vi "WVDIAL_Main_1.0.vi"() -> ()   [LabVIEW 2012]
uses:
  <vilib>/DAQmx/write.llb/DAQmx Write (Digital 1D Bool NChan 1Samp 1Line).vi
  <vilib>/DAQmx/miscellaneous.llb/DAQmx Fill In Error Info.vi
  under_development/AMCS_Data.vi
  <vilib>/Analysis/baseanly.llb/Mean (DBL).vi
  H2O_DIAL/LabVIEW-2012/Scalar_Data.vi
  H2O_DIAL/LabVIEW-2012/Bristol WM V2_31b/CLDevIFace.dll
  <vilib>/Analysis/NI_AALBase.lvlib
panel:
  out "AMCS_Profile":i32
  out "FileHour":i32=18
  out "L_Count":i32=12
  out "sigma_off_total":dbl[](array[numeric])=[4.888035870829203e-25, 4.854608115475229e-25, 4.821315130033936e-25, 4.788157195692115e-25, 4.755134589463832e-25, 4.722247583943701e-25, 4.689496446877888e-25, 4.656881440910823e-25, 4.6244028232034e-25, 4.592060845167014e-25, 4.55985575212019e-25, 4.527787783052784e-25, 4.495857170275024e-25, 4.4640641392417e-25, 4.432408908236268e-25, 4.400891688098754e-25, 4.369512682080274e-25, 4.338272085590705e-25, 4.307170085904759e-25, 4.276206862115827e-25, 4.245382584820222e-25, 4.214697415991576e-25, 4.184151508878279e-25, 4.153745007733512e-25, 4.123478047759034e-25, 4.093350754997215e-25, 4.0633632461153848e-25, 4.0335156284150834e-25, 4.0038079996697135e-25, 3.9742404480868766e-25, 3.9448130521677145e-25, 3.915525880745368e-25, 3.886378992858531e-25, 3.8573724377461643e-25, 3.8285062548278185e-25, 3.7997804736545024e-25, 3.7711951139370566e-25, 3.7427501855176308e-25, 3.7144456884042655e-25, 3.686281612771603e-25, 3.658257939015542e-25, 3.6303746377467797e-25, 3.602631669916555e-25, 3.5750289867515567e-25, 3.5475665299476097e-25, 3.5202442316525487e-25, 3.4930620145687864e-25, 3.466019792025494e-25, 3.4391174681118262e-25, 3.412354937708723e-25, 3.385732086655022e-25, 3.3592487917865697e-25, 3.3329049211414267e-25, 3.306700333974482e-25, 3.280634880983416e-25, 3.2547084043508965e-25, 3.228920737922699e-25, 3.203271707354926e-25, 3.1777611302055785e-25, 3.1523888161216317e-25, 3.127154566968838e-25, 3.102058176967416e-25, 3.0770994328759967e-25, 3.0522781141008815e-25, 3.0275939928903318e-25, 3.0030468344607627e-25, 2.9786363971981933e-25, 2.9543624327416916e-25, 2.930224686195949e-25, 2.906222896311306e-25, 2.882356795584999e-25, 2.8586261104367467e-25, 2.835030561394528e-25, 2.811569863239953e-25, 2.788243725123392e-25, 2.7650518508047145e-25, 2.741993938722939e-25, 2.719069682202312e-25, 2.696278769575161e-25, 2.673620884356008e-25, 2.651095705348542e-25, 2.628702906852776e-25, 2.6064421587391947e-25, 2.584313126623251e-25, 2.562315472013588e-25, 2.540448852422533e-25, 2.518712921495533e-25, 2.4971073291533783e-25, 2.475631721705256e-25, 2.454285741983474e-25, 2.433069029434547e-25, 2.411981220251513e-25, 2.3910219474927565e-25, 2.370190841148622e-25, 2.3494875282985535e-25, 2.3289116331441013e-25, 2.3084627771705737e-25, 2.2881405791714577e-25, 2.2679446553956784e-25, 2.2478746195897673e-25, 2.22793008307951e-25, 2.208110654850464e-25, 2.188415941625169e-25, 2.168845547931586e-25, 2.149399076143407e-25, 2.1300761265550973e-25, 2.110876297449633e-25, 2.0917991851171733e-25, 2.072844383934657e-25, 2.054011486389122e-25, 2.0353000831508104e-25, 2.016709763077787e-25, 1.998240113264655e-25, 1.979890719093385e-25, 1.9616611642341368e-25, 1.943551030698017e-25, 1.925559898865328e-25, 1.9076873474916518e-25, 1.8899329537437417e-25, 1.8722962932379024e-25, 1.8547769400210756e-25, 1.8373744666260693e-25, 1.8200884440825555e-25, 1.8029184419330962e-25, 1.785864028250439e-25, 1.768924769659363e-25, 1.7521002313557632e-25, 1.735389977127581e-25, 1.7187935693766226e-25, 1.702310569139568e-25, 1.6859405361114919e-25, 1.6696830286658545e-25, 1.6535376038945889e-25, 1.6375038176257498e-25, 1.621581224454772e-25, 1.6057693777875647e-25, 1.5900678298637916e-25, 1.5744761318177563e-25, 1.558993833699771e-25, 1.543620484527584e-25, 1.5283556323523553e-25, 1.513198824282104e-25, 1.498149606572178e-25, 1.4832075246641388e-25, 1.4683721232497087e-25, 1.4536429463567547e-25, 1.4390195374017408e-25, 1.424501439277071e-25, 1.4100881944445769e-25, 1.3957793449837002e-25, 1.381574432716146e-25, 1.3674729992776922e-25, 1.353474586215468e-25, 1.3395787350844606e-25, 1.325784987569173e-25, 1.3120928855546477e-25, 1.2985019712580151e-25, 1.2850117873277534e-25, 1.2716218769548856e-25, 1.2583317839794236e-25, 1.2451410530256942e-25, 1.2320492295860694e-25, 1.2190558601549445e-25, 1.2061604923388985e-25, 1.1933626749670006e-25, 1.1806619582041493e-25, 1.1680578936635882e-25, 1.1555500345124245e-25, 1.1431379355845816e-25, 1.130821153462839e-25, 1.11859924660529e-25, 1.106471775420178e-25, 1.094438302366916e-25, 1.0824983920307019e-25, 1.0706516112017506e-25, 1.0588975289648329e-25, 1.0472357167332237e-25, 1.0356657483440625e-25, 1.024187200079566e-25, 1.0127996507244631e-25, 1.0015026816012569e-25, 9.902958765939357e-26, 9.791788221702149e-26, 9.68151107381336e-26, 9.572123238770103e-26, 9.463620658860708e-26, 9.355999302019208e-26, 9.249255161638679e-26, 9.143384256042965e-26, 9.038382628274446e-26, 8.934246345371541e-26, 8.830971497843464e-26, 8.728554198992872e-26, 8.62699058411531e-26, 8.526276809671997e-26, 8.426409052334914e-26, 8.327383508075767e-26, 8.229196391044237e-26, 8.131843932536565e-26, 8.035322379788044e-26, 7.939627994867628e-26, 7.844757053335767e-26, 7.750705843063878e-26, 7.65747066289159e-26, 7.565047821351042e-26, 7.47343363532067e-26, 7.382624428699225e-26, 7.292616531039518e-26, 7.203406276287137e-26, 7.114990001406464e-26, 7.027364045059868e-26, 6.940524746389362e-26, 6.85446844368123e-26, 6.769191473247965e-26, 6.684690168165317e-26, 6.600960857107768e-26, 6.517999863394936e-26, 6.435803503717334e-26, 6.354368087372936e-26, 6.273689915185572e-26, 6.193765278681275e-26, 6.114590459282069e-26, 6.036161727495792e-26, 5.958475342308923e-26, 5.881527550516134e-26, 5.805314586163766e-26, 5.729832670099857e-26, 5.655078009533302e-26, 5.581046797662917e-26, 5.507735213469193e-26, 5.435139421405333e-26, 5.36325557132649e-26, 5.292079798345033e-26, 5.221608222852683e-26, 5.1518369505608076e-26, 5.0827620725253844e-26, 5.014379665432141e-26, 4.9466857916821155e-26, 4.879676499724133e-26, 4.8133478243835596e-26, 4.7476957871630115e-26, 4.6827163967351294e-26, 4.618405649298157e-26, 4.554759529166947e-26, 4.491774009265494e-26, 4.4294450516974745e-26, 4.3677686083139524e-26, 4.306740621440293e-26, 4.2463570244387956e-26, 4.1866137424661286e-26, 4.127506693180156e-26, 4.069031787434629e-26, 4.011184930095246e-26, 3.953962020783545e-26, 3.8973589546741365e-26, 3.84137162332915e-26, 3.785995915494e-26, 3.7312277179583384e-26, 3.677062916385059e-26, 3.623497396187796e-26, 3.5705270434125054e-26, 3.518147745597146e-26, 3.4663553926918453e-26, 3.4151458779350305e-26, 3.3645150987763337e-26, 3.3144589578214325e-26, 3.264973363720337e-26, 3.216054232151887e-26, 3.1676974867802074e-26, 3.119899060201809e-26, 3.072654894964087e-26, 3.025960944534977e-26, 2.979813174386497e-26, 2.9342075629720175e-26, 2.889140102874887e-26, 2.8446068018571114e-26, 2.800603684031854e-26]
  out "sigma_on_total":dbl[](array[numeric])=[3.490042879585289e-23, 3.4896341790922685e-23, 3.4889762071158304e-23, 3.488068250151699e-23, 3.486909676211499e-23, 3.48549993542674e-23, 3.4838385609191393e-23, 3.4819251695340833e-23, 3.479759462007997e-23, 3.477341223906918e-23, 3.4746703260906816e-23, 3.47174672467967e-23, 3.4685704618961385e-23, 3.465141665984221e-23, 3.461460551401806e-23, 3.457527419211947e-23, 3.453342656969817e-23, 3.448906738624602e-23, 3.4442202246214284e-23, 3.4392837616682326e-23, 3.434098082430858e-23, 3.428664005432775e-23, 3.422982434615018e-23, 3.417054358917814e-23, 3.4108808516072814e-23, 3.4044630702817483e-23, 3.397802255409811e-23, 3.390899730392353e-23, 3.383756900435442e-23, 3.376375251923111e-23, 3.368756351057052e-23, 3.360901843775463e-23, 3.3528134537865166e-23, 3.344492982272624e-23, 3.335942306183597e-23, 3.3271633776370865e-23, 3.318158221993735e-23, 3.3089289371486604e-23, 3.299477691788866e-23, 3.2898067243876535e-23, 3.279918341157314e-23, 3.269814915144566e-23, 3.259498884386024e-23, 3.24897275031573e-23, 3.238239076130052e-23, 3.227300485415394e-23, 3.21615965972714e-23, 3.204819337748524e-23, 3.193282312695606e-23, 3.181551430802064e-23, 3.169629589879774e-23, 3.157519736729644e-23, 3.1452248655446696e-23, 3.132748016189897e-23, 3.120092272051889e-23, 3.107260757867697e-23, 3.094256638256482e-23, 3.081083115312845e-23, 3.0677434265982754e-23, 3.054240843226174e-23, 3.0405786681460624e-23, 3.0267602333919474e-23, 3.012788898770482e-23, 2.99866804931177e-23, 2.984401093546342e-23, 2.9699914613734513e-23, 2.955442601832349e-23, 2.940757981602586e-23, 2.925941082278427e-23, 2.9109953991996763e-23, 2.895924438752617e-23, 2.8807317167162414e-23, 2.865420756317372e-23, 2.849995086407571e-23, 2.834458239150023e-23, 2.818813748548795e-23, 2.803065148592016e-23, 2.787215971116496e-23, 2.771269744109115e-23, 2.755229990137636e-23, 2.739100224507032e-23, 2.7228839532475316e-23, 2.706584671843548e-23, 2.690205863490408e-23, 2.673750997388079e-23, 2.657223527172833e-23, 2.6406268893866064e-23, 2.6239645021831286e-23, 2.607239763477325e-23, 2.5904560500280996e-23, 2.5736167156696623e-23, 2.5567250898853516e-23, 2.539784477107411e-23, 2.5227981549794207e-23, 2.5057693731555458e-23, 2.4887013522394087e-23, 2.471597282956038e-23, 2.454460324501361e-23, 2.437293603900355e-23, 2.4201002150211167e-23, 2.402883217538624e-23, 2.385645635851179e-23, 2.3683904585127427e-23, 2.351120637608329e-23, 2.3338390871505237e-23, 2.3165486834754068e-23, 2.2992522636352133e-23, 2.2819526251359127e-23, 2.2646525256153023e-23, 2.2473546815634482e-23, 2.230061768719921e-23, 2.2127764207900367e-23, 2.195501229556526e-23, 2.1782387440441194e-23, 2.160991470701159e-23, 2.143761872556912e-23, 2.1265523693862868e-23, 2.109365337122134e-23, 2.0922031077433445e-23, 2.0750679694496088e-23, 2.0579621658458087e-23, 2.0408878965264313e-23, 2.0238473165015015e-23, 2.0068425366661072e-23, 1.9898756232137357e-23, 1.9729485980000502e-23, 1.9560634386795936e-23, 1.9392220786262192e-23, 1.9224264070473828e-23, 1.9056782690457042e-23, 1.8889794661029254e-23, 1.8723317558719184e-23, 1.855736852629747e-23, 1.8391964275893473e-23, 1.8227121088478705e-23, 1.806285481900235e-23, 1.7899180898616018e-23, 1.773611433861678e-23, 1.7573669732317703e-23, 1.741186125936493e-23, 1.7250702690911692e-23, 1.7090207391268152e-23, 1.6930388321237217e-23, 1.6771258046596068e-23, 1.661282873734126e-23, 1.6455112174985683e-23, 1.6298119756367283e-23, 1.614186249828583e-23, 1.598635104155938e-23, 1.5831595657904855e-23, 1.567760625211793e-23, 1.552439236910916e-23, 1.5371963196965152e-23, 1.522032757473284e-23, 1.5069493995606855e-23, 1.4919470612189036e-23, 1.477026524242552e-23, 1.4621885376172283e-23, 1.4474338176755096e-23, 1.4327630490148282e-23, 1.4181768849089416e-23, 1.403675947667607e-23, 1.3892608295456937e-23, 1.3749320929216795e-23, 1.3606902710831856e-23, 1.3465358687081003e-23, 1.332469362175979e-23, 1.3184912006315121e-23, 1.304601805945408e-23, 1.2908015735995458e-23, 1.2770908731077424e-23, 1.2634700487137352e-23, 1.2499394195353328e-23, 1.2364992805313888e-23, 1.2231499026968916e-23, 1.2098915337982155e-23, 1.1967243987797148e-23, 1.1836487002238083e-23, 1.1706646189619215e-23, 1.1577723145735427e-23, 1.1449719257807597e-23, 1.1322635710406168e-23, 1.1196473489796478e-23, 1.1071233389221606e-23, 1.0946916011717084e-23, 1.0823521778637897e-23, 1.0701050929498414e-23, 1.0579503530345327e-23, 1.0458879477268549e-23, 1.0339178499011404e-23, 1.0220400163641383e-23, 1.0102543881484885e-23, 9.985608910260597e-24, 9.869594358367067e-24, 9.754499189862458e-24, 9.640322227217557e-24, 9.527062156995094e-24, 9.414717532061861e-24, 9.303286777093004e-24, 9.192768189885375e-24, 9.083159948714375e-24, 8.974460112323461e-24, 8.866666625126608e-24, 8.759777321083854e-24, 8.653789926727215e-24, 8.548702063774183e-24, 8.444511253202335e-24, 8.341214918838909e-24, 8.238810389419842e-24, 8.137294903148705e-24, 8.036665608577946e-24, 7.936919569739024e-24, 7.838053767973498e-24, 7.740065104792213e-24, 7.642950405338446e-24, 7.546706420091712e-24, 7.451329828211826e-24, 7.356817239808839e-24, 7.263165198494959e-24, 7.170370184815645e-24, 7.078428616460998e-24, 6.987336853161977e-24, 6.897091197425113e-24, 6.8076878974105e-24, 6.719123148241058e-24, 6.631393095931324e-24, 6.54449383712704e-24, 6.4584214234832185e-24, 6.3731718616386814e-24, 6.288741117137584e-24, 6.205125113814784e-24, 6.1223197384036285e-24, 6.040320840135283e-24, 5.959124233842455e-24, 5.878725700858363e-24, 5.79912099094532e-24, 5.720305824157253e-24, 5.64227589189973e-24, 5.565026858473326e-24, 5.4885543637702884e-24, 5.412854022527149e-24, 5.3379214276707424e-24, 5.263752150713538e-24, 5.190341743319676e-24, 5.1176857383675426e-24, 5.045779651873086e-24, 4.974618983303745e-24, 4.9041992172131e-24, 4.8345158245928204e-24, 4.765564263342602e-24, 4.697339979783611e-24, 4.629838410103098e-24, 4.563054980342238e-24, 4.496985108006421e-24, 4.431624203399418e-24, 4.36696766956464e-24, 4.3030109039670755e-24, 4.2397492991573704e-24, 4.177178243062485e-24, 4.115293120908651e-24, 4.054089314905932e-24, 3.993562205740054e-24, 3.933707172949696e-24, 3.8745195958165464e-24, 3.815994853553171e-24, 3.7581283271459395e-24, 3.700915398498208e-24, 3.644351452219004e-24, 3.5884318755724674e-24, 3.533152059539341e-24, 3.4785073989091114e-24, 3.4244932929904e-24, 3.371105146433994e-24, 3.3183383692901385e-24, 3.2661883776563498e-24, 3.2146505942936803e-24, 3.1637204489385725e-24]
  out "background start":u32=269
  in  "Tab Control 2":enum32{"WV ND far", "WV ND near"}(tab)
  out "Water Vapor Number Density":dbl[][](graph)=[[0.5267745722096372, 1.0816655502265025, 0.7857849169072013, 0.7477019555239035, 1.1563560837736724, 1.3171998032055208, 1.3231734283890237, 1.0229480459758586, 0.8099310805147446, 1.0288102942698314, 1.0490255634819494, 0.8954092055648583, 0.9324215101778409, 0.8762260068675822, 0.7790591099414911, 0.8327406457641141, 0.7704082202159364, 0.5844811914297862, 0.6547568349937917, 0.8309364506920026, 0.8146764873524291, 0.7795089686669525, 0.7138471934895959, 0.6391289574628901, 0.6939700094906176, 0.7387482811512458, 0.5462573277969212, 0.33740432735257525, 0.524099558332941, 0.5415332827292677, 0.25587531060911606, 0.32034867927546745, 0.3575458365147231, 0.19987909534956147, -0.04398480306339893, -0.3018841632955589, -0.08562036624041874, 0.3956793663354093, 0.316745841175725, -0.17952793102078793, 0.10063267322036752, 0.11266719606812724, 0.029212134890287074, -0.005416362214295599, -0.001903108817248135, 0.024827606151215636, 0.09438149063711843, 0.13636686041364063, 0.09853184491889724, 0.02006830264986938, -0.1100190870486176, -0.011423208972600938, 0.22560075143987507, 0.23855203986244836, 0.18772422030911864, 0.1248592220030643, -0.1159789262566526, -0.09672114603628404, -0.002076973429409002, 0.07764150511111109, 0.08671851842324418, 0.010370500718089025, -0.04877001832258952, -0.09879008518513611, 0.196069456255276, 0.16890990444127219, 0.2027158700169282, 0.47342868266577487, 0.2732503005639838, -0.21673756779330117, -0.009709955271929215, 0.1780787605318169, -0.18035544514716292, -0.09516280572167025, -0.210624930189063, 0.15126704138773134, 0.37711181552750694, -0.2407750842687604, -0.06818293330208619, 0.4479847852605204, 0.15992717017361327, -0.026875771508593577, 0.33346537041116026, 0.6057422007030442, 0.2837007114383953, -0.387948288010905, -0.430868484135778, 0.1171368056605578, 0.2825750335377916, 0.25290766375296486, 0.3235685707096946, 0.294635786603805, 0.15630875076023204, -0.17215583026651332, 0.07190604755466319, 0.5111632653992029, 0.4545339946147383, 0.1397417212111138, -0.379868786050122, -0.8200386753384453, 0.9689769619728654, 1.2154721509976958, 0.027706077248837634, -0.451600315057674, -0.18393792610598184, 0.26802923421484454, 0.06982906738396868, 0.008175721206703183, 0.34464584312575747, 0.775324515204279, -0.9206634231342339, -1.054693026338104, 0.05417378371590325, 0.3787930859671527, 0.1528806900268664, -0.17890474033164738, -0.03290798453116943, 0.17150327086091385, 0.10226783329265791, 0.026323152799793855, 0.14546580088898983, 0.15324308143002588, 0.1999669318893245, -0.3505358779777044, -0.6040003896777243, -0.19197175189892304, 0.41483200698530504, 0.25996478520600325, 0.1901900371465814, -0.7004410472584591, 0.03417523868208899, 0.9773516762567699, 0.9501600424919857, 3.8179055985644914, -0.7387811622909695, -1.292310093419745, -3.4707865579805204, -4.806919839772366, -3.2236942041133716, -0.2798646999882494, -0.5041588894213339, 0.15387554509916093, -2.286184189921483, -6.1689901157875, 0.4414912597114918, -1.0941982539352222, 4.107096638589786, 7.0494086102953135, 5.093420412613982, -1.186817248260524, -2.4693646495361077, 17.233690686949487, 0.16757072698059172, 0.7104219413732543, 11.659803406100098, 0.9497546635922111, -4.150373043253479, -4.099503865718477, -20.766083051079526, -9.002561009044582, 8.821221493764776, -17.7174813523336, -1.1751756583085076, -6.409331662715958, -12.307070884759122, 3.2739376460348315, -0.16355277685023256, -1.7278023908845879, 20.244230401911185, 8.261047619107535, -11.304691487958216, -8.357847181177188, -0.683969220017551, 25.576749641541674, 0.03888795481451756, -3.5614818406988205, 7.989633180877991, 10.328796990583767, -2.196067163503004, -3.4876165534276327, -5.383896494369181, -15.158339724766968, -9.002865651652682, -16.098176364767838, 7.287929865782665, 1.9677812793929124, 5.186685665765197, -0.8233271906171977, 1.5188061622709401, 9.881681545336587, 13.354340316245327, 17.543981154187094, 2.971290702331586, -13.18169395475072, -15.400954328693494, -13.957629394095024, -31.075136408591785, -26.935662472931995, -8.138951564843802, -7.326056577513869, -3.502353752083309, 3.911699212234371, -4.294086845093831, 23.18118721705451, 14.987899790461576, 6.437164591458738, -2.523411218458799, 6.497127824545888, -1.9683154922323156, 0.7529285854770654, -25.600648943018182, -10.52685287943841, 20.134382483909995, -6.0244636268000615, 21.12692930038622, 2.144915244484192, 47.75224805371796, 3.818730797626004, -6.536865277783475, 13.099227893812442, 48.22712037716169, 45.290460164779205, 3.60781654357059, 15.912476957433306, -33.947777326737814, 21.4727068022259, -34.11700126806532, 5.3665409079956214, 33.86809985241948, -37.57424460030235, -85.7767439605924, -52.75415349112659, -34.88803865506797, -22.239237234636768, 19.69441058235572, -105.06374008086121, -8.755512075683884, -6.4485892955900175, -1.0583048975403269, 23.788435843550058, 62.07659802333474, 22.437904657032785, 7.423763482952456, -1.4124692383830593, -51.624147123828145, 45.16870976535536, 28.56129984362196, -2.639584028437023, -24.22307764432475, 7.240569189963771, -7.739305471169459, -37.35816143994053, 1.0244452934635038, -10.305504179883442, 16.74709280360141, 1.888878380765623, -16.968743658232242, 13.056677566409775, 17.44799599784629, -7.35298759849147, -0.1908743950074914, -11.436677267617473, 4.855902298247621, -10.394570497652436, 14.487727137462723, 26.002729568728288, -31.076998008605173, -112.89098296015568, -50.76728953266004, -8.064309931248644, -18.781235808776238, 16.929688279117574, -17.58011679033343, -5.052252895180237, -20.3864023129576, -12.830066550660884, 0.0, 0.0, 0.0, 0.0]]
  out "Water Vapor Number Density 2":dbl[][](graph)=[[1.1482348388286592, 2.017982964091594, 1.3682209057856505, 0.9162759140798291, 0.8730221012994673, 0.9800120948533376, 0.9568537175790923, 0.866174390917249, 0.8322568386031581, 0.9145888482232154, 0.9995806717132666, 0.9531087725615546, 1.0027170536110341, 0.9780362537283204, 0.8214444226402221, 0.7374418214571511, 0.728929939395368, 0.8703742010291748, 1.071802251618865, 1.067496178736125, 0.9632781842428743, 0.5850509830524605, 0.5299677426827336, 1.232228916363148, 1.1947823041340582, 0.5755124205878246, 0.24107527679833016, 0.36120813676368274, 1.857720171772897, 2.0226877693479377, 0.08008274693316024, 0.21246078901144208, -0.38825066117973206, -0.6512609902264878, 2.4697972044926857, 3.05183936691486, 1.3210540191735825, 1.5010114687713463, 1.5841384087891783, -1.5431482483032921, 0.7537197793292203, 0.0142388790717362, 0.6151589653849325, 0.7709348719560961, 0.14508807566929505, 0.8473160303976256, 2.9128420979360485, 1.2361887916417282, 0.30367357027724207, -0.31756832810140895, 0.5175885514437972, 3.1255462584899183, -0.04741866121062809, -0.4465986867615582, 1.973698376075153, 2.084298847160525, -1.1989514112505324, 3.207256643769982, 5.084149530819217, -0.9930683196577749, -1.4840633762509645, -1.7903252900489475, 0.09525360963538727, 2.021893560647792, -3.6857123070952897, -2.4863589570055713, 5.377983282689115, -4.4837626044312735, -7.170301852225106, -1.5988976164601776, -0.6472380955667218, -0.17486017044227684, -1.807472441762057, -5.807871907238444, -1.8194438056280375, -1.6378718054314585, -8.08715743525793, -3.5276357892740404, -1.448942460179607, -0.3828715269407209, -3.906520032128574, -6.188436108313037, -1.5053386433922895, 0.8478303538029819, -1.0624702577421266, -3.424309784862931, -4.162092350147047, -2.045289494277629, 0.3427998595393124, 6.183381896974018, 5.087306891745131, 4.657546326812751, 2.1698725029395725, 1.9822046828495878, 3.733444191959902, 4.407445010510418, 5.407381709221487, 5.77186598747299, 0.1744940060694488, -9.538408364233964, -5.225557667222109, -3.4750634711519623, -1.332858938900355, -0.43613205023126805, -5.567981458980698, -3.6656128441263354, 0.13805919420361193, 0.15591842248018312, 4.25351494330367, 8.58621786113748, 6.014221100385406, 5.493699084832289, 5.124620087499465, 2.220464139386139, 7.982407875894793, 8.860414085357473, 11.457583755603755, 11.990190824053256, 3.5235722536705074, 2.662910069631187, 3.734703453366167, 3.0373461568850852, 0.6773280687838767, -1.6342998299530764, -4.416478062077773, -9.14817150589161, -18.369883547739253, -16.998585716560267, -7.623625250864538, -34.78753621623293, -17.462034998576804, -16.181966218859696, -16.69591012751227, -10.342960592270106, -7.3153681405610085, -6.564954093999361, -4.874601216220289, -10.731216108408299, -7.353667743190857, 24.98585965038712, 4.387442673833919, 5.892704810900461, 0.7265435527596306, 1.6049835807593127, 14.828929983331067, 7.814113832945408, 11.56352961739801, 15.249123217630238, -1.9672780242029846, -3.238730845882112, -5.386418691339414, -3.256927254738442, 3.240335742201914, 1.0758432659412893, -10.791653002785928, -8.503377636088308, -13.626346267996807, -16.717338136517693, 2.092822808182948, -3.1255841458145244, 1.5041464075655948, 2.7461899514385597, -4.559881528359264, -7.512724382895494, -15.090641272222895, 0.4864987387567519, 5.860091651366822, 2.040121802031853, -8.644611780816092, -1.9955260024974544, 7.644719590093669, -4.2857183474271, 6.026072423617071, 12.338991043031633, 15.935813432274939, 6.935794704068874, 2.370316907310191, 12.804449889870984, 17.056330249490287, -7.141531043058103, 1.0309181815046982, 5.446204975309789, 2.929068924969034, -17.34022502189193, -4.520356657726189, -9.394904841373238, -5.704065411207677, -10.292661605158417, -1.6461826137905238, 13.596061247174136, -11.946912991702753, -1.0721465368957719, -2.315049684200968, -4.131898641063062, 18.2619381019155, 7.655880810498651, 14.32882718637709, 16.718018640743008, 6.9320430358992855, 7.933278564150358, 21.202651560733255, 12.54213142332888, 2.671162232018715, 9.435685473567505, -28.813035717756524, 0.2694192423490834, -9.46869876404097, -13.180732228133888, -17.101846176918887, -3.000370971183812, -19.892888505980086, -22.831318340260335, -19.702730534731067, 19.046722143789548, 9.278612919223075, 12.762128661997307, -16.82645445230673, -5.185296067643773, 4.971769835684121, -17.74768315072377, 9.174131935499624, 8.673827267138527, 18.97417971925629, 14.582965839362355, 9.173074771606416, -2.4830127571103247, 15.157228942776038, -3.1771316538481407, 20.188638904880687, 18.656336030733762, 7.1691301126291025, 21.64913513475193, -8.679041930587214, -20.824928136859096, 3.702289918633733, -8.050228239521887, 6.668136930501031, 3.540233933767305, -27.88252229180155, -4.517923708576304, -11.11151463093389, -42.3421237896053, 16.554738391364598, -0.29976193039047205, -15.090548270003252, -26.52314938964792, 8.921722883415631, -12.395945589138586, -2.9664183562583624, 28.894097539785346, -50.7751959690825, 14.215917783653273, 48.67748289843371, -13.981472248510729, -0.24275583657935043, 37.605111906152636, 40.03308160431177, 65.9972193016789, -31.176395411615765, -18.58261116176528, 75.01621451876315, 23.274997786719492, -19.37932577173951, 16.850317265784106, -11.2165756307649, -38.58812387391493, -105.91721045226694, -82.50134324417745, 48.5820651901375, -63.867352907328325, -28.14789674369646, -22.105991710093, -45.47034660589086, -13.255556485070557, 11.287337342159965, 17.814689816182348, 0.0, 0.0, 0.0, 0.0]] caption="Water Vapor Number Density"
  out "RingBuffer offline near":dbl[][](array[numeric])
  out "RingBuffer aerosol near":dbl[][](array[numeric])
  in  "LOWER DISPLAY TAB":T1(tab)=enum."Raw Counts far"
  out "NRB":dbl[][](graph)=[[0.00966033479932111, 0.027195908002200102, 0.00012534084631067143, 0.0002299139662858806, 0.00037820150832913377, 0.0005886583472799488, 0.0009404220364040007, 0.0015072912842579401, 0.0023358438081163297, 0.0032872937181813683, 0.00455665129407164, 0.0062647427585960785, 0.008357837083727199, 0.010660565396095646, 0.013078936151425151, 0.015466872769922287, 0.018037135401161412, 0.021332577302686045, 0.024089767965532607, 0.026816781528413887, 0.03010730387726353, 0.03309137070132408, 0.035865135040327595, 0.038321594053622864, 0.040813835620001314, 0.04245738157426946, 0.04407673957308234, 0.04695785113513908, 0.04791914724712515, 0.04746226016415504, 0.04845953561835384, 0.04879425868329584, 0.0486400429525818, 0.04807923477869758, 0.04814251466139775, 0.04810793443174457, 0.04685503122270601, 0.04762062594730987, 0.04803509765817138, 0.046175594679338544, 0.044460965750299605, 0.04501417164546444, 0.045062636793090055, 0.043976107037945, 0.043563648058121504, 0.04352891011695816, 0.043129774330031116, 0.04345346761335059, 0.04304918518157886, 0.04190336529265434, 0.041695314691605125, 0.04110088438296421, 0.04025541898004086, 0.03975491572536978, 0.0382604509453086, 0.03605405826501201, 0.03688567123319064, 0.03785613107966538, 0.036571983399793305, 0.03706514732277742, 0.038207986379640214, 0.038045704266900085, 0.03587855703300304, 0.0351000746806936, 0.03557430917918744, 0.03566500861893972, 0.03496561582376826, 0.0360171547269112, 0.03684718890396368, 0.033991905643973024, 0.031790661342134145, 0.03051285681902415, 0.030629302848660517, 0.032292147751852164, 0.032486202216154746, 0.02974761603892747, 0.027190243065387653, 0.02904532272325952, 0.03131388587368813, 0.031934642819108135, 0.02950789552835881, 0.027265496277769224, 0.02862046702355488, 0.026777379676977735, 0.028457783827368865, 0.03281325751645602, 0.031152468071345994, 0.03294361685880173, 0.03176876238034591, 0.024601486635277392, 0.021945160581454994, 0.02341318526869295, 0.02779971478932544, 0.031382000735252664, 0.031454232434717774, 0.05720221586563123, 0.22967498388491822, 0.9510227395678853, 2.1119385686025347, 2.676670216733895, 2.2115568417005607, 1.2990801737018083, 0.5077044140595494, 0.10459652743584678, 0.022692586198310667, 0.020330580865231453, 0.026857907595799334, 0.04168400733394855, 0.04574532879247362, 0.03721883908482395, 0.03006194171774844, 0.028524751842058396, 0.04386730590876011, 0.05550172009115171, 0.04945710486112076, 0.03975248154133065, 0.04551362519661975, 0.08018453542412719, 0.15536106525000654, 0.22812841351300397, 0.25610389240406606, 0.22788529863652693, 0.18364884221087582, 0.1932003071230838, 0.19044806456262492, 0.26750960179785915, 0.45761266702884473, 0.4905455206292651, 0.30942606018309043, 0.15725973786667324, 0.12180141332353024, 0.12347527105564035, 0.13562955188353212, 0.10846985185514085, 0.05253093056443529, 0.022624430385616387, 0.01787246073138078, 0.01750244387416274, 0.024915751940450582, 0.017796661333062406, -0.0006376163107507473, 0.010280402000023637, 0.01901987933413353, 0.0188281412960399, 0.02490402375397111, 0.012753722888290794, 0.003967068036500632, 0.0115308985485483, 0.022368245846969594, 0.016199424706321783, 0.002168591347604111, -0.0012520050243982888, 0.004685852481248283, 0.01209135160843883, 0.01650024955895803, 0.031113773705947225, 0.0379207176309806, 0.02598037286015007, 0.013867847967928667, 0.021262674110661562, 0.01737239150760298, 0.010477744854997934, 0.013399001630740232, 0.005383856138051768, 0.009514472292225217, 0.008563505227992546, 0.0011103499315003322, -0.002153724214534944, -0.0018635800265769922, 0.002429050927450199, -0.0036865374988006767, 0.002977307940900013, 0.015589988191279344, 0.0030469502169648745, 0.003251418667250475, 0.01048277603610767, -0.0015244813643492824, -0.007848876968540905, -0.0036852009506297156, 0.019564634882583143, 0.03681237705516316, 0.013224539726297502, -0.00014814460474804242, 0.00827476851975799, 0.003065870140649466, -0.0016834548591090606, -0.022391054460695663, -0.01500940196798429, 0.007940488489103548, 0.0054296574689305386, 0.012345756475117634, -0.012393501486067906, 0.0008650835533769395, 0.05415382822562538, 0.03515726576936434, 0.010238998945387065, 0.0260099973773606, 0.018470208562522086, 0.010554836454505239, 0.01840284432096861, 0.00987443652430123, 0.009521665895309318, 0.021921487217036056, 0.028351527896747192, 0.009574202129171185, -0.005350087387541653, -0.0020850490593699892, -0.009760604490086611, -0.024588070568491497, -0.01726469402339514, -0.008320935515068342, 0.0022864103118399276, 0.017109755143844475, 0.0066347577466083964, 0.010019832259967876, 5.159780963548357e-05, -0.020517855443308364, -0.0020497486054468664, 0.024452408268356172, 0.02574680242919132, 0.013827800654345853, -0.0013080985983945546, -0.0029697931894683205, 0.02558170257653174, 0.040647998285275266, 0.05004850853341707, 0.0641704661499282, 0.03311515869765881, 0.013687091981180738, 0.020827452991154405, 0.030746472978744513, 0.046192997568068384, 0.047492722316837425, 0.03548658303664799, 0.02601819375230289, 0.012072786967034522, 0.020561495773413797, 0.027626419854275688, -0.00025268500008399515, -0.0002548039425927088, 0.002633555430323123, -0.008031077396447879, -0.005485471785806571, 0.008625358922221972, -0.019516308335895818, -0.013652753821238938, 0.05573312001514799, 0.05244403510117128, 0.001782773950534994, 0.002488324096194588, 0.030030089581459644, 0.024300067708812014, 0.025201218119296827, 0.0307522302731298, 0.025960804724746253, 0.04029851162500861, 0.020160639558067944, -0.015753348236443386, 0.003412573205067065, 0.014279316781720553, -0.025161984761202537, -0.04623087103868022, -0.013310096115604273, 0.018190644013660544, 0.008620661162973784, 0.00868584551438053, -0.003468950556452362, -0.00548076417179556, -0.00472149134495073, -0.0063690823875805535, 0.005766629123306216, -0.008918380233906868, -0.019286812593432904, -0.004483504464045601, 0.03312011413462398, 0.00556015752018423, 0.015783370552987605, 0.0, 0.0, 0.0]] caption="Water Vapor Number Density"
  out "NRB 2":dbl[][](graph)=[[0.010066328750861737, 0.028437948160746983, 0.0002656381986401233, 0.0006683614001951439, 0.001499218193894854, 0.002573906423220097, 0.0037964163769247084, 0.005268321147310943, 0.007038776076792629, 0.009167370374030228, 0.011086348288138391, 0.012702595934183101, 0.014052312958287932, 0.01502926968691142, 0.01620019177314933, 0.016651469793176377, 0.017308096356940528, 0.018708481049867626, 0.01925210533123308, 0.01921984967320506, 0.01963137374954457, 0.02057302669413183, 0.0203932689814336, 0.021197783269397526, 0.02286003789601638, 0.02255968450417337, 0.02157423540759892, 0.022061575696229813, 0.0219683921875737, 0.022170430357128245, 0.02203756889068404, 0.021964782705618868, 0.021935588344671103, 0.02055660186057779, 0.019244556729830924, 0.01898052883438301, 0.019363530690844507, 0.02184739700764918, 0.02284107791255665, 0.017243700956712793, 0.018476276851429493, 0.020053927570951847, 0.017221012379873467, 0.017715271103476572, 0.018176307942604466, 0.018647713557250954, 0.017850928363072102, 0.015791748362570353, 0.01552423714696966, 0.016009583003722763, 0.014870624523226083, 0.015337771879127497, 0.016565656269019166, 0.019182302968780512, 0.020427085686063932, 0.02193555421017249, 0.020001548004371438, 0.011623494120125678, 0.012145272538100185, 0.017138341554770453, 0.01830064700708862, 0.015617883467987521, 0.014674175233444584, 0.013714877708238994, 0.013956645829494706, 0.013629633067923844, 0.011318173641317849, 0.009135196106928384, 0.008923741491916095, 0.015056087154273095, 0.016198382539608154, 0.011728906351649323, 0.011937051013496833, 0.013652670346290387, 0.012631741505294085, 0.0037753411093709053, 0.006076577913689129, 0.01219071406151726, 0.008502827219011432, 0.013796029108238895, 0.015730272887832856, 0.015099703090061766, 0.01252478787951747, 0.015765864490924625, 0.010493748822589372, 0.0042517657872661934, 0.005330483290491611, 0.007980317271828363, 0.013242474765623204, 0.010443195579020128, 0.007508877948002532, -0.0019900298367020682, 0.010810432169561702, 0.007167150953875807, -0.007299681549398742, 0.01608147384161722, 0.09653065968226052, 0.4034603273240936, 0.8969391711019737, 1.144018655394251, 0.9523875487546432, 0.5634249635618747, 0.21991186115911918, 0.04023230884237633, 0.012539809112822308, 0.008228997853127898, 0.013537305020805527, 0.024749546421945153, 0.009369711263715746, 0.020092864998752864, 0.02427211075311975, 0.009257510451995344, 0.007843352521215246, 0.02311605589126513, 0.01876189753650916, -0.005510005349236035, 0.006175405857220577, 0.027821651075074488, 0.045742948508924915, 0.06701383278998783, 0.09829031332607632, 0.09481207764096314, 0.07449268021980301, 0.09145640875019888, 0.07324218732419052, 0.08531770937357783, 0.21069563189769255, 0.23340071735542642, 0.10675348960445874, 0.04717403095378305, 0.04645433920489944, 0.0669689168010332, 0.07555172143042496, 0.05810260639269271, 0.03210932446443566, 0.004806577264486242, 0.010050760921159179, 0.009555277595392615, 0.02806224512128018, 0.028026431700330603, -0.006128090662517846, -0.014494622293070662, 0.0019783988981582367, 0.008771255388039282, 0.0010880188012935635, 0.01201419772046282, -0.0017988984160091212, -0.01254218133833262, -0.006468580450346505, -0.008707149568575727, -0.009336625443514482, -0.03687940348284756, -0.02393706475911046, -0.0009071129774714162, 0.011649053886461763, 0.048078315843038316, -0.008706920425415933, -0.020612836475661787, 0.028612335229884947, 0.00262074514151426, -0.002886866592347311, -0.004989478459701897, -0.02044371409579717, -0.026443805456398226, -0.020182839811158374, 0.019871389803458924, 0.03595682487694968, 0.043692330236875736, 0.025415977786176026, -0.0054944340605618345, 0.007763372974566596, 0.02333082552190612, 0.021750981437440576, -0.010353993677721786, -0.0016881572942306813, -0.0020559752707081116, -0.018643767640562803, -0.011904789160820078, -0.0077136048281018915, 0.046147141525947954, 0.0586407728583584, 0.04401058318905229, 0.042423252247648244, 0.0009902644134859077, -0.036537013684471036, -0.0168907497126951, 0.0444948045840488, 0.042784887563892086, -0.001969066667990667, 0.00450789714190633, 0.053806703173063776, 0.018496416366128622, -0.03012807069623865, -0.04123683388917122, 0.009026043529006144, 0.05882178356162903, 0.03060593590047507, 0.03951821724898995, 0.01831038924861832, 0.0065698785203179896, 0.03595220470359223, 0.037458493692738376, 0.0294851357866592, -0.004400763733580146, -0.0425002766000521, -0.03766499443460818, -0.02887338092094355, 0.0007787331060656494, 0.08138165437229349, 0.07471955527116045, 0.05965423968165909, 0.10775512645492454, 0.03271683422823081, 0.0036578756836891818, 0.070778762628496, 0.07590062555117986, 0.10653982854799669, 0.1206249822266633, 0.0723576648558154, -0.0029402195250157813, 0.05280416052630273, 0.09653392588866005, 0.04900861177828946, 0.04013479271303853, 0.031665928430877816, 0.01729540972796543, 0.04875347808851532, 0.07257834861145533, 0.058171273195694935, 0.112544776246243, 0.07179924518404701, 0.02730881686505033, 0.07854513405955846, 0.041334134713995364, -0.04684186832406001, -0.03283120827504304, 0.036397533896756075, 0.0290582346591594, 0.019663680351469735, 0.07069845912315902, 0.038616653825470075, 0.04091438086102416, 0.07546654380081748, 0.06336226703406236, 0.06523333757484899, 0.08380958327014561, 0.12430510230292885, 0.10074754901796039, 0.07679782498387155, 0.0412031680820322, -0.05946136892699566, -0.10743891043699216, -0.11189321959939734, -0.06887427245777454, 0.06444881466325471, 0.07159118663548872, 0.07698172808702168, 0.09181110190195946, 0.05667553433990292, 0.05217058618696721, 0.032263605996648514, 0.10008621176788239, 0.07867265818819105, 0.09573896736910993, 0.14584808057377227, 0.15690239811321666, 0.15086526732086353, -0.020926954743736202, -0.05934166245033883, 0.043958648374962946, 0.08063969867389074, -0.027382244199822086, -0.04351353051191394, 0.020776991074964182, 0.028585962585297366, 0.060503173623026964, -0.06292376305125755, 0.0, 0.0, 0.0]] caption="Water Vapor Number Density"
  out "raw counts":dbl[][](graph)=[[17708.0, 57593.0, 96.0, 68.0, 98.0, 45.0, 90.0, 79.0, 126.0, 118.0, 106.0, 119.0, 146.0, 182.0, 139.0, 195.0, 252.0, 186.0, 235.0, 200.0, 219.0, 235.0, 237.0, 242.0, 188.0, 199.0, 252.0, 255.0, 243.0, 259.0, 203.0, 173.0, 180.0, 142.0, 134.0, 177.0, 178.0, 141.0, 160.0, 190.0, 131.0, 127.0, 143.0, 120.0, 90.0, 92.0, 145.0, 93.0, 70.0, 76.0, 63.0, 131.0, 77.0, 66.0, 58.0, 70.0, 40.0, 40.0, 87.0, 29.0, 52.0, 42.0, 76.0, 27.0, 63.0, 59.0, 52.0, 73.0, 35.0, 85.0, 60.0, 8.0, -8.0, 25.0, 56.0, 44.0, 44.0, 34.0, 22.0, 21.0, 49.0, 42.0, 22.0, 13.0, -10.0, 37.0, 52.0, 39.0, 29.0, 31.0, 7.0, 5.0, 55.0, 56.0, 21.0, -10.0, 5.0, 518.0, 2657.0, 4826.0, 5565.0, 4534.0, 2200.0, 522.0, 23.0, -20.0, -16.0, -5.0, 14.0, 1.0, 12.0, -14.0, 27.0, -12.0, 19.0, 7.0, -13.0, 7.0, 18.0, 80.0, 99.0, 40.0, 39.0, 68.0, 70.0, 71.0, 120.0, 212.0, 182.0, 10.0, 0.0, 24.0, 0.0, 10.0, 20.0, 4.0, -3.0, -19.0, 13.0, 11.0, -5.0, 9.0, 25.0, -1.0, 30.0, 22.0, 2.0, 12.0, -6.0, 10.0, 1.0, -13.0, -15.0, -20.0, 6.0, 9.0, 34.0, 32.0, 15.0, 10.0, 16.0, -5.0, -3.0, 1.0, 1.0, -22.0, 0.0, -7.0, -43.0, -25.0, 21.0, -13.0, -9.0, -9.0, -9.0, 51.0, 26.0, 15.0, -10.0, -10.0, 27.0, 27.0, 1.0, -7.0, -24.0, -9.0, 25.0, -45.0, -16.0, -13.0, -1.0, -21.0, -20.0, -3.0, 35.0, 4.0, -11.0, 21.0, 19.0, -8.0, 4.0, 13.0, 22.0, -3.0, 4.0, 5.0, -29.0, -13.0, -39.0, 5.0, -20.0, -27.0, 8.0, 25.0, 9.0, -17.0, -4.0, -44.0, 25.0, 18.0, -12.0, 20.0, -8.0, -2.0, 19.0, -7.0, 13.0, 49.0, -18.0, 5.0, -4.0, 33.0, 17.0, 36.0, 29.0, 4.0, -1.0, 2.0, 30.0, -18.0, 19.0, -1.0, 34.0, -12.0, -18.0, -7.0, 4.0, 28.0, 8.0, 19.0, -17.0, -4.0, 17.0, 2.0, -8.0, 8.0, 7.0, -8.0, -15.0, 23.0, -9.0, 27.0, -3.0, 16.0, 4.0, 19.0, 17.0, -11.0, -1.0, 38.0, 11.0, -15.0, -3.0, -14.0, -22.0, 14.0, -18.0, 36.0, -27.0, 0.0]] caption="Water Vapor Number Density"
  out "raw counts near":dbl[][](graph)=[[15237.6, 56742.6, 103.59999999999991, 115.59999999999991, 179.5999999999999, 240.5999999999999, 248.5999999999999, 325.5999999999999, 338.5999999999999, 357.5999999999999, 281.5999999999999, 325.5999999999999, 305.5999999999999, 221.5999999999999, 194.5999999999999, 273.5999999999999, 253.5999999999999, 244.5999999999999, 274.5999999999999, 213.5999999999999, 116.59999999999991, 207.5999999999999, 108.59999999999991, 142.5999999999999, 113.59999999999991, 129.5999999999999, 149.5999999999999, 66.59999999999991, 108.59999999999991, 98.59999999999991, 195.5999999999999, 52.59999999999991, 51.59999999999991, 0.599999999999909, 82.59999999999991, 1.599999999999909, 132.5999999999999, -9.400000000000091, 120.59999999999991, -46.40000000000009, 5.599999999999909, 73.59999999999991, 6.599999999999909, 36.59999999999991, -13.400000000000091, -9.400000000000091, 128.5999999999999, 72.59999999999991, 35.59999999999991, 7.599999999999909, 56.59999999999991, -11.400000000000091, 58.59999999999991, 23.59999999999991, 29.59999999999991, 11.599999999999909, 113.59999999999991, 93.59999999999991, -50.40000000000009, 68.59999999999991, 38.59999999999991, 4.599999999999909, 54.59999999999991, 8.599999999999909, -91.40000000000009, 32.59999999999991, 60.59999999999991, -37.40000000000009, 15.599999999999909, -111.40000000000009, 73.59999999999991, 4.599999999999909, 70.59999999999991, 2.599999999999909, 1.599999999999909, -3.400000000000091, -74.40000000000009, 65.59999999999991, -33.40000000000009, 113.59999999999991, 0.599999999999909, 42.59999999999991, -53.40000000000009, -38.40000000000009, 89.59999999999991, -92.40000000000009, 48.59999999999991, -59.40000000000009, -64.40000000000009, 28.59999999999991, 0.599999999999909, -95.40000000000009, 24.59999999999991, 23.59999999999991, 2.599999999999909, -10.400000000000091, -79.40000000000009, 238.5999999999999, 1173.6, 2065.6, 2314.6, 1954.6, 950.5999999999999, 190.5999999999999, -53.40000000000009, -49.40000000000009, -71.40000000000009, -17.40000000000009, -108.40000000000009, 1.599999999999909, 63.59999999999991, -28.40000000000009, -21.40000000000009, -37.40000000000009, -61.40000000000009, -28.40000000000009, -2.400000000000091, 1.599999999999909, -51.40000000000009, 33.59999999999991, -91.40000000000009, 97.59999999999991, 96.59999999999991, 13.599999999999909, -30.40000000000009, -64.40000000000009, 66.59999999999991, 135.5999999999999, 25.59999999999991, -37.40000000000009, 2.599999999999909, 77.59999999999991, 22.59999999999991, -121.40000000000009, 66.59999999999991, -67.40000000000009, 16.59999999999991, -18.40000000000009, -16.40000000000009, 54.59999999999991, -27.40000000000009, -48.40000000000009, 14.599999999999909, -28.40000000000009, -62.40000000000009, -74.40000000000009, 2.599999999999909, 57.59999999999991, 48.59999999999991, 15.599999999999909, 20.59999999999991, -75.40000000000009, -5.400000000000091, 10.599999999999909, -120.40000000000009, -36.40000000000009, 45.59999999999991, -65.40000000000009, 1.599999999999909, -52.40000000000009, 3.599999999999909, 54.59999999999991, -49.40000000000009, 56.59999999999991, -53.40000000000009, 55.59999999999991, 31.59999999999991, -5.400000000000091, -50.40000000000009, -55.40000000000009, 46.59999999999991, 38.59999999999991, -21.40000000000009, 3.599999999999909, -50.40000000000009, -7.400000000000091, -23.40000000000009, -34.40000000000009, -64.40000000000009, 10.599999999999909, -0.40000000000009095, -136.4000000000001, 49.59999999999991, 79.59999999999991, -63.40000000000009, -88.40000000000009, -20.40000000000009, 100.59999999999991, -31.40000000000009, 22.59999999999991, 63.59999999999991, 20.59999999999991, 24.59999999999991, -43.40000000000009, 48.59999999999991, 85.59999999999991, -55.40000000000009, 0.599999999999909, 14.599999999999909, -51.40000000000009, -27.40000000000009, -41.40000000000009, -44.40000000000009, 54.59999999999991, 5.599999999999909, -11.400000000000091, 27.59999999999991, 74.59999999999991, -58.40000000000009, 92.59999999999991, 2.599999999999909, 83.59999999999991, -25.40000000000009, 34.59999999999991, -13.400000000000091, -2.400000000000091, -66.40000000000009, -7.400000000000091, -32.40000000000009, -21.40000000000009, -77.40000000000009, -14.400000000000091, -3.400000000000091, 78.59999999999991, -20.40000000000009, -7.400000000000091, 27.59999999999991, 89.59999999999991, 21.59999999999991, -12.400000000000091, 34.59999999999991, -45.40000000000009, 80.59999999999991, -50.40000000000009, -36.40000000000009, -56.40000000000009, -72.40000000000009, -42.40000000000009, 48.59999999999991, -23.40000000000009, -45.40000000000009, -59.40000000000009, 54.59999999999991, 117.59999999999991, 55.59999999999991, 15.599999999999909, -10.400000000000091, -20.40000000000009, 65.59999999999991, 47.59999999999991, 1.599999999999909, -111.40000000000009, -65.40000000000009, -43.40000000000009, -68.40000000000009, -74.40000000000009, 3.599999999999909, -92.40000000000009, -17.40000000000009, 44.59999999999991, 10.599999999999909, 29.59999999999991, -60.40000000000009, 14.599999999999909, 61.59999999999991, -37.40000000000009, 75.59999999999991, -36.40000000000009, -1.400000000000091, 20.59999999999991, -18.40000000000009, 70.59999999999991, 52.59999999999991, 32.59999999999991, -48.40000000000009, 59.59999999999991, 2.599999999999909, -146.4000000000001, -25.40000000000009, 0.0]] caption="Water Vapor Number Density"
  out "Aerosol Smoothed 2":dbl[](array[numeric])=[37670.00588235294, 29029.417647058825, 154.15294117647062, 218.06470588235297, 312.8294117647058, 372.7999999999999, 403.8882352941175, 429.03529411764697, 452.8294117647058, 477.6235294117646, 477.35882352941167, 459.6529411764705, 433.35882352941167, 399.74117647058813, 375.41764705882343, 339.24117647058813, 312.41764705882343, 301.24117647058824, 278.27058823529416, 250.77058823529413, 232.35882352941175, 221.88823529411764, 201.27058823529413, 192.15294117647062, 190.97647058823532, 174.2705882352941, 154.56470588235294, 146.9764705882353, 136.4470588235294, 128.68235294117648, 119.8, 112.06470588235294, 105.24117647058824, 92.91764705882352, 82.0941176470588, 76.53529411764703, 73.91764705882349, 79.06470588235291, 78.47647058823527, 56.32941176470585, 57.44705882352938, 59.417647058823505, 48.68235294117645, 47.82941176470585, 46.917647058823505, 46.06470588235291, 42.24117647058821, 35.82941176470585, 33.79999999999997, 33.47647058823526, 29.888235294117617, 29.65294117647056, 30.829411764705853, 34.38823529411762, 35.29999999999997, 36.56470588235291, 32.18235294117644, 18.06470588235291, 18.241176470588208, 24.88823529411762, 25.711764705882324, 21.241176470588208, 19.329411764705853, 17.505882352941146, 17.27058823529409, 16.358823529411737, 13.182352941176442, 10.329411764705853, 9.799999999999972, 16.06470588235291, 16.79999999999997, 11.829411764705853, 11.711764705882324, 13.03529411764703, 11.741176470588206, 3.4176470588235004, 5.358823529411736, 10.476470588235266, 7.123529411764677, 11.270588235294088, 12.53529411764703, 11.741176470588208, 9.505882352941148, 11.682352941176442, 7.594117647058795, 3.005882352941147, 3.6823529411764415, 5.388235294117618, 8.741176470588206, 6.741176470588206, 4.741176470588206, -1.2294117647059113, 6.53529411764703, 4.241176470588207, -4.229411764705911, 9.123529411764677, 53.623529411764686, 219.3, 476.79999999999995, 595.5058823529412, 486.3882352941175, 282.5647058823529, 108.29999999999998, 19.447058823529378, 5.947058823529383, 3.8294117647058536, 6.182352941176442, 11.094117647058795, 4.123529411764677, 8.682352941176442, 10.299999999999972, 3.858823529411736, 3.211764705882324, 9.29999999999997, 7.4176470588235, -2.141176470588264, 2.358823529411736, 10.447058823529382, 16.888235294117617, 24.329411764705853, 35.094117647058795, 33.29999999999997, 25.741176470588208, 31.094117647058795, 24.505882352941146, 28.09411764705879, 68.27058823529408, 74.44705882352937, 33.53529411764703, 14.594117647058795, 14.15294117647056, 20.094117647058795, 22.329411764705853, 16.917647058823498, 9.211764705882324, 1.358823529411736, 2.7999999999999714, 2.623529411764677, 7.594117647058795, 7.476470588235265, -1.6117647058823816, -3.758823529411793, 0.5058823529411478, 2.211764705882324, 0.27058823529408893, 2.9470588235293826, -0.4352941176470879, -2.9941176470588524, -1.5235294117647347, -2.0235294117647347, -2.141176470588264, -8.34705882352944, -5.347058823529441, -0.20000000000002882, 2.5352941176470303, 10.329411764705853, -1.8470588235294407, -4.3176470588235585, 5.917647058823501, 0.5352941176470303, -0.5823529411764994, -0.9941176470588524, -4.023529411764735, -5.141176470588264, -3.876470588235323, 3.770588235294089, 6.741176470588206, 8.094117647058795, 4.652941176470559, -0.9941176470588522, 1.3882352941176184, 4.123529411764677, 3.799999999999971, -1.7882352941176758, -0.2882352941176758, -0.34705882352944073, -3.111764705882382, -1.96470588235297, -1.2588235294117935, 7.4470588235293835, 9.358823529411737, 6.9470588235293835, 6.623529411764677, 0.1529411764705595, -5.582352941176499, -2.552941176470617, 6.652941176470559, 6.329411764705854, -0.2882352941176758, 0.6529411764705595, 7.711764705882324, 2.623529411764677, -4.229411764705912, -5.729411764705912, 1.241176470588206, 8.005882352941148, 4.123529411764677, 5.270588235294089, 2.417647058823501, 0.858823529411736, 4.652941176470559, 4.799999999999971, 3.7411764705882065, -0.5529411764706171, -5.288235294117676, -4.641176470588264, -3.523529411764734, 0.09411764705879477, 9.741176470588206, 8.858823529411735, 7.005882352941148, 12.53529411764703, 3.770588235294089, 0.41764705882350084, 8.005882352941148, 8.505882352941148, 11.829411764705855, 13.270588235294088, 7.888235294117618, -0.3176470588235585, 5.652941176470559, 10.241176470588206, 5.152941176470559, 4.1823529411764415, 3.2705882352940887, 1.770588235294089, 4.9470588235293835, 7.299999999999971, 5.799999999999971, 11.123529411764677, 7.035294117647029, 2.6529411764705597, 7.5647058823529125, 3.947058823529383, -4.4352941176470875, -3.082352941176499, 3.3882352941176186, 2.682352941176442, 1.7999999999999714, 6.417647058823501, 3.4764705882352653, 3.6529411764705593, 6.6823529411764415, 5.5647058823529125, 5.6823529411764415, 7.241176470588206, 10.65294117647056, 8.564705882352913, 6.476470588235266, 3.447058823529383, -4.9352941176470875, -8.84705882352944, -9.141176470588263, -5.5823529411765, 5.1823529411764415, 5.711764705882324, 6.094117647058795, 7.211764705882325, 4.4176470588235, 4.03529411764703, 2.4764705882352653, 7.623529411764677, 5.9470588235293835, 7.182352941176442, 10.858823529411737, 11.594117647058795, 11.064705882352913, -1.5235294117647347, -4.288235294117676, 3.1529411764705593, 5.741176470588206, -1.935294117647088, -3.0529411764706174, 1.4470588235293829, 1.9764705882352651, 4.152941176470559, -4.288235294117676]
  out "Off-Line Smoothed 2":dbl[](array[numeric])=[37328.52390109891, 28783.346703296702, 137.9373626373627, 209.6118131868131, 300.3302197802196, 353.8384615384614, 370.59945054945047, 389.7326923076923, 417.02527472527464, 435.19148351648334, 439.81785714285706, 430.36593406593397, 411.6365384615384, 389.01840659340655, 368.05137362637345, 344.90851648351634, 323.843956043956, 302.09807692307686, 279.4002747252746, 260.6186813186812, 245.25879120879108, 232.28763736263727, 217.4483516483516, 202.46071428571432, 188.85494505494518, 180.2560439560441, 169.7065934065935, 158.8604395604396, 149.65851648351656, 138.5142857142858, 129.47719780219788, 120.63516483516489, 111.5225274725275, 102.29587912087916, 91.92087912087916, 86.35631868131873, 82.3398351648352, 76.87005494505496, 73.15027472527476, 66.97857142857146, 61.50054945054948, 57.034890109890135, 51.67774725274724, 47.58296703296698, 44.63653846153839, 44.26565934065927, 40.87417582417576, 36.272527472527415, 33.65989010989004, 34.38104395604388, 33.42087912087905, 31.530769230769167, 30.67774725274719, 26.91263736263731, 25.85631868131864, 26.290384615384575, 26.04862637362634, 23.914010989010976, 21.40302197802198, 19.680494505494508, 18.69972527472528, 18.081593406593413, 18.886538461538464, 17.393406593406603, 14.71346153846154, 14.278021978021975, 13.48543956043956, 12.680494505494508, 12.573351648351654, 11.260164835164842, 9.375549450549457, 10.702472527472533, 10.97582417582418, 10.151648351648355, 10.793131868131873, 10.657142857142862, 10.712087912087913, 11.75329670329671, 9.486813186813194, 6.832967032967034, 7.338461538461539, 7.912637362637365, 8.49505494505495, 7.51978021978022, 6.874175824175822, 6.184615384615382, 3.692857142857138, 3.614560439560437, 5.187362637362634, 5.125549450549449, 4.37554945054945, 4.11318681318681, 4.685989010989007, 5.092582417582415, 6.7436813186813165, 17.673626373626362, 151.15302197802197, 445.54587912087914, 637.2368131868134, 552.2024725274727, 353.039010989011, 194.84807692307692, 84.31373626373625, 23.305494505494497, 5.4964285714285674, 2.756043956043952, 2.801373626373622, 4.195604395604393, 4.96208791208791, 4.224450549450546, 2.6296703296703274, 4.209340659340658, 9.224450549450554, 19.22994505494502, 29.056868131868065, 27.795879120879057, 25.022527472527408, 27.495054945054875, 28.532142857142787, 23.9112637362637, 19.194230769230764, 19.294505494505486, 20.008791208791198, 19.25741758241758, 16.121428571428577, 17.00879120879121, 23.316483516483515, 22.804120879120877, 12.951098901098899, 6.529395604395601, 4.754670329670327, 3.1804945054945044, 3.6914835164835145, 3.588461538461537, 1.1887362637362624, -0.006318681318682443, -0.6615384615384626, -0.37445054945055056, -0.2480769230769242, -0.8043956043956058, 0.5802197802197788, -0.32637362637362777, -0.9568681318681332, -0.6038461538461553, -1.5557692307692321, -1.4582417582417597, 0.9098901098901089, 2.6173076923076906, 0.7752747252747234, -1.0667582417582429, -1.1917582417582433, -1.1354395604395617, -1.4170329670329675, -1.5379120879120887, 0.478571428571427, 1.8412087912087896, 0.573351648351647, 2.022527472527472, 1.3604395604395596, -1.3277472527472542, -1.3881868131868147, 0.19972527472527324, 0.37142857142857, 0.2999999999999986, 1.5802197802197788, 1.2175824175824161, 0.757417582417581, 0.15989010989010827, 0.16675824175824044, 0.1543956043956034, 0.0815934065934053, 0.3879120879120865, -0.8016483516483531, -0.4980769230769245, -0.2535714285714299, -0.2851648351648365, 1.1049450549450535, 0.7931318681318666, 0.821978021978021, 2.56098901098901, 2.654395604395603, 2.272527472527471, 1.6461538461538447, 1.5115384615384606, 2.345329670329669, 0.17774725274725112, -2.915659340659342, -1.4651098901098916, 1.1324175824175806, -0.10796703296703469, -0.8634615384615398, -0.5626373626373641, -0.4568681318681333, 0.1557692307692292, 1.2807692307692293, 1.540384615384614, 0.32747252747252603, 1.1791208791208776, 1.8796703296703279, -0.13956043956044106, -1.437637362637364, -0.6010989010989025, -1.6189560439560453, -1.617582417582419, 1.0815934065934052, 2.0733516483516468, 1.0156593406593393, 0.6282967032967018, 1.6557692307692293, 0.1887362637362623, -0.2728021978021992, 2.039010989010988, 0.7560439560439551, -0.5722527472527488, -0.21236263736263883, -0.11346153846153995, 0.8439560439560425, 0.5651098901098887, 0.05274725274725131, -1.3359890109890125, 0.4085164835164823, 2.37142857142857, 0.2752747252747238, 0.805494505494504, 1.6983516483516468, 0.5939560439560425, 1.5156593406593393, 0.3370879120879109, -0.4953296703296717, 1.7752747252747239, 1.8659340659340646, 1.363186813186812, 1.7340659340659326, 0.29313186813186665, -1.0104395604395617, 0.6640109890109878, 0.6598901098901085, 0.34258241758241603, 0.5802197802197788, -1.3497252747252761, -1.0159340659340672, 0.9552197802197788, 1.6296703296703283, 0.8755494505494492, 0.5129120879120864, 1.5541208791208776, 0.7065934065934051, 0.10082417582417438, 0.801373626373625, 1.1351648351648338, 0.32884615384615246, -0.10247252747252888, 0.6901098901098887, -0.1821428571428586, 0.49917582417582274, 1.2821428571428557, 0.029395604395602966, 0.30686813186813044, 1.73131868131868, 0.8357142857142843, 0.9923076923076903, 2.4648351648351627, 2.1557692307692293, 0.6708791208791199, -0.19313186813186922, 1.4799450549450537, 1.702472527472526, 0.76153846153846, -0.8689560439560454, -0.992582417582419, -0.4293956043956058, -0.3002747252747267, -0.12857142857143, 0.2120879120879106, 0.6392857142857128, 0.19697802197802056, 0.5651098901098887]
  out "Off-Line Bin Readings 2":dbl[](array[numeric])=[17884.0, 59389.0, 2750.0, 2762.0, 2826.0, 2887.0, 2895.0, 2972.0, 2985.0, 3004.0, 2928.0, 2972.0, 2952.0, 2868.0, 2841.0, 2920.0, 2900.0, 2891.0, 2921.0, 2860.0, 2763.0, 2854.0, 2755.0, 2789.0, 2760.0, 2776.0, 2796.0, 2713.0, 2755.0, 2745.0, 2842.0, 2699.0, 2698.0, 2647.0, 2729.0, 2648.0, 2779.0, 2637.0, 2767.0, 2600.0, 2652.0, 2720.0, 2653.0, 2683.0, 2633.0, 2637.0, 2775.0, 2719.0, 2682.0, 2654.0, 2703.0, 2635.0, 2705.0, 2670.0, 2676.0, 2658.0, 2760.0, 2740.0, 2596.0, 2715.0, 2685.0, 2651.0, 2701.0, 2655.0, 2555.0, 2679.0, 2707.0, 2609.0, 2662.0, 2535.0, 2720.0, 2651.0, 2717.0, 2649.0, 2648.0, 2643.0, 2572.0, 2712.0, 2613.0, 2760.0, 2647.0, 2689.0, 2593.0, 2608.0, 2736.0, 2554.0, 2695.0, 2587.0, 2582.0, 2675.0, 2647.0, 2551.0, 2671.0, 2670.0, 2649.0, 2636.0, 2567.0, 2885.0, 3820.0, 4712.0, 4961.0, 4601.0, 3597.0, 2837.0, 2593.0, 2597.0, 2575.0, 2629.0, 2538.0, 2648.0, 2710.0, 2618.0, 2625.0, 2609.0, 2585.0, 2618.0, 2644.0, 2648.0, 2595.0, 2680.0, 2555.0, 2744.0, 2743.0, 2660.0, 2616.0, 2582.0, 2713.0, 2782.0, 2672.0, 2609.0, 2649.0, 2724.0, 2669.0, 2525.0, 2713.0, 2579.0, 2663.0, 2628.0, 2630.0, 2701.0, 2619.0, 2598.0, 2661.0, 2618.0, 2584.0, 2572.0, 2649.0, 2704.0, 2695.0, 2662.0, 2667.0, 2571.0, 2641.0, 2657.0, 2526.0, 2610.0, 2692.0, 2581.0, 2648.0, 2594.0, 2650.0, 2701.0, 2597.0, 2703.0, 2593.0, 2702.0, 2678.0, 2641.0, 2596.0, 2591.0, 2693.0, 2685.0, 2625.0, 2650.0, 2596.0, 2639.0, 2623.0, 2612.0, 2582.0, 2657.0, 2646.0, 2510.0, 2696.0, 2726.0, 2583.0, 2558.0, 2626.0, 2747.0, 2615.0, 2669.0, 2710.0, 2667.0, 2671.0, 2603.0, 2695.0, 2732.0, 2591.0, 2647.0, 2661.0, 2595.0, 2619.0, 2605.0, 2602.0, 2701.0, 2652.0, 2635.0, 2674.0, 2721.0, 2588.0, 2739.0, 2649.0, 2730.0, 2621.0, 2681.0, 2633.0, 2644.0, 2580.0, 2639.0, 2614.0, 2625.0, 2569.0, 2632.0, 2643.0, 2725.0, 2626.0, 2639.0, 2674.0, 2736.0, 2668.0, 2634.0, 2681.0, 2601.0, 2727.0, 2596.0, 2610.0, 2590.0, 2574.0, 2604.0, 2695.0, 2623.0, 2601.0, 2587.0, 2701.0, 2764.0, 2702.0, 2662.0, 2636.0, 2626.0, 2712.0, 2694.0, 2648.0, 2535.0, 2581.0, 2603.0, 2578.0, 2572.0, 2650.0, 2554.0, 2629.0, 2691.0, 2657.0, 2676.0, 2586.0, 2661.0, 2708.0, 2609.0, 2722.0, 2610.0, 2645.0, 2667.0, 2628.0, 2717.0, 2699.0, 2679.0, 2598.0, 2706.0, 2649.0, 2500.0, 2621.0]
  out "On-Line Smoothed 2":dbl[](array[numeric])=[37645.22032967034, 29055.970329670334, 123.55824175824173, 171.80686813186816, 233.59120879120883, 263.8549450549451, 263.41950549450553, 262.6846153846154, 268.57609890109893, 268.28076923076924, 259.99093406593414, 241.47582417582427, 219.5623626373627, 197.91263736263735, 177.11181318681315, 158.72307692307686, 143.25879120879117, 128.9153846153846, 114.72307692307692, 101.75879120879121, 90.2793956043956, 81.35494505494505, 72.57472527472527, 66.81785714285714, 59.73681318681318, 52.51840659340658, 47.576098901098895, 43.675000000000004, 40.94972527472528, 36.72582417582419, 29.414010989011004, 26.125549450549464, 25.131043956043953, 21.69285714285713, 21.52390109890109, 19.536263736263727, 15.109065934065926, 12.871428571428567, 11.787637362637359, 9.68186813186813, 8.488186813186811, 9.57884615384615, 8.771153846153842, 6.349450549450545, 6.337087912087906, 5.563736263736258, 5.198351648351645, 6.007417582417578, 4.036263736263733, 3.4469780219780173, 4.305494505494503, 3.529395604395604, 1.317857142857141, 2.0046703296703265, 3.154395604395601, 3.8027472527472503, 2.592582417582415, 0.926373626373624, 2.5939560439560423, 2.4085164835164816, 0.9717032967032938, -0.7810439560439595, -1.4239010989011025, 0.30961538461538096, -0.18214285714286027, -3.073626373626377, -2.5214285714285736, 1.1008241758241746, 1.4236263736263715, -0.5571428571428595, -2.4170329670329695, -1.3813186813186842, -0.08324175824176039, -1.2961538461538487, -3.04203296703297, -4.3387362637362665, -2.561263736263739, -1.1148351648351675, -2.2755494505494527, -3.8826923076923103, -3.889560439560442, -2.0241758241758268, -2.0241758241758268, -4.127197802197805, -3.4719780219780247, -2.8936813186813213, -4.2041208791208815, -4.2151098901098925, -2.334615384615387, -2.0873626373626397, -3.481593406593409, -4.072252747252749, -5.743956043956047, -6.145054945054947, -3.0750000000000024, -0.8524725274725298, 25.151648351648358, 88.79038461538462, 129.11593406593406, 109.07060439560439, 69.45659340659341, 36.95659340659341, 13.692857142857143, 3.280769230769228, -2.2082417582417606, -3.967857142857145, -2.8936813186813213, -2.8181318681318706, -1.636813186813189, -1.0063186813186835, -3.4651098901098925, -2.853846153846157, 1.5499999999999965, 2.813736263736261, 2.9813186813186787, 2.312362637362636, 3.4744505494505464, 3.022527472527469, 1.8247252747252714, 2.7931318681318658, 1.8398351648351625, 0.7656593406593376, -0.09972527472527709, 0.07197802197802022, 0.5431318681318654, -0.6093406593406625, -0.97747252747253, -0.9445054945054976, -0.6436813186813217, -1.0928571428571459, -1.4596153846153876, -1.6409340659340683, -3.697252747252749, -1.8909340659340677, -0.3620879120879146, -3.2027472527472556, -3.6931318681318706, -1.470604395604398, -1.3181318681318703, -2.466483516483519, -1.4142857142857166, -1.0543956043956069, -3.6862637362637383, -5.654670329670331, -3.807142857142859, -1.0461538461538487, -1.6574175824175847, -2.4032967032967054, -3.2384615384615407, -2.1931318681318706, 0.08846153846153602, -0.5585164835164858, -0.34423076923077156, 0.36043956043955816, -1.6326923076923099, -2.743956043956046, -3.202747252747255, -3.804395604395607, -2.4582417582417606, -2.011813186813189, -1.304395604395607, -0.6409340659340684, -1.834615384615387, -2.716483516483519, -3.4376373626373655, -3.603846153846157, -2.9239010989011014, -0.18076923076923324, 0.7615384615384593, -1.066758241758244, -1.569505494505497, -1.1711538461538484, -1.3002747252747278, -2.8346153846153874, -2.8538461538461566, -1.263186813186816, -1.0969780219780247, -2.183516483516486, -1.290659340659343, -1.9431318681318703, -2.716483516483519, -2.0461538461538487, -1.8318681318681342, -0.9115384615384639, -1.2934065934065955, -2.184890109890112, -2.5241758241758268, -1.5640109890109914, -1.0873626373626397, -1.265934065934068, -1.8428571428571452, -2.246703296703299, -1.265934065934068, -0.4939560439560462, -1.0543956043956066, -2.209615384615387, -1.720604395604398, -1.5997252747252768, -2.761813186813188, -2.4417582417582433, -0.2590659340659366, 0.7917582417582393, -0.63269230769231, -0.5200549450549474, -0.37582417582417826, -1.0365384615384639, 0.297252747252745, -0.1642857142857167, -1.5804945054945083, -0.7054945054945082, -1.8167582417582442, -2.4431318681318706, -0.9760989010989033, -0.9582417582417605, 0.5980769230769206, -0.08873626373626631, -2.738461538461541, -2.2989010989011014, -0.47747252747252983, -0.6134615384615405, -0.884065934065936, -0.7851648351648375, -2.1052197802197825, -2.3469780219780243, -2.7961538461538487, -3.0681318681318706, -1.9225274725274748, -0.5475274725274748, -0.6038461538461561, -0.23983516483516715, 1.628296703296701, -0.6725274725274748, -2.689010989010991, -1.0131868131868154, -0.2673076923076946, -0.5461538461538484, -0.42802197802198033, -0.0804945054945077, -1.3510989010989034, -1.25769230769231, 0.6516483516483492, 0.959340659340657, -1.3813186813186837, -1.9060439560439584, -1.345604395604398, -1.849725274725277, -1.121703296703299, 0.6667582417582394, 0.5307692307692284, -1.1395604395604417, -0.680769230769233, 0.6956043956043934, -0.3524725274725299, -0.8950549450549474, 1.5348901098901075, 0.24368131868131626, -1.264560439560442, 0.709340659340657, 0.06236263736263492, -2.1120879120879144, -2.021428571428574, -1.4293956043956069, -0.11620879120879357, -0.055769230769233125, -2.892307692307695, -0.9870879120879146, 0.6461538461538439, 0.40302197802197565, 0.12967032967032732, 0.8260989010988987, 1.2972527472527449, -1.2714285714285738, -2.187637362637365, -1.61758241758242, 0.6475274725274702, 3.2725274725274702, 1.0513736263736233]
  out "On-Line Bin Readings 2":dbl[](array[numeric])=[18280.0, 59794.0, 2762.0, 2660.0, 2847.0, 2742.0, 2784.0, 2926.0, 2855.0, 2911.0, 2810.0, 2758.0, 2732.0, 2752.0, 2850.0, 2745.0, 2650.0, 2652.0, 2748.0, 2732.0, 2826.0, 2748.0, 2667.0, 2645.0, 2640.0, 2728.0, 2703.0, 2716.0, 2667.0, 2623.0, 2597.0, 2636.0, 2596.0, 2557.0, 2723.0, 2639.0, 2606.0, 2654.0, 2675.0, 2644.0, 2674.0, 2635.0, 2640.0, 2622.0, 2703.0, 2683.0, 2568.0, 2734.0, 2645.0, 2622.0, 2685.0, 2721.0, 2666.0, 2625.0, 2658.0, 2653.0, 2615.0, 2677.0, 2631.0, 2556.0, 2637.0, 2593.0, 2664.0, 2561.0, 2691.0, 2668.0, 2588.0, 2613.0, 2600.0, 2735.0, 2662.0, 2645.0, 2620.0, 2693.0, 2692.0, 2648.0, 2715.0, 2648.0, 2614.0, 2686.0, 2632.0, 2558.0, 2658.0, 2650.0, 2696.0, 2625.0, 2632.0, 2627.0, 2578.0, 2648.0, 2572.0, 2634.0, 2660.0, 2547.0, 2457.0, 2647.0, 2642.0, 2600.0, 2903.0, 3014.0, 3056.0, 3122.0, 2921.0, 2776.0, 2599.0, 2606.0, 2666.0, 2636.0, 2644.0, 2665.0, 2661.0, 2675.0, 2678.0, 2641.0, 2645.0, 2661.0, 2679.0, 2605.0, 2620.0, 2739.0, 2638.0, 2627.0, 2583.0, 2637.0, 2606.0, 2617.0, 2662.0, 2735.0, 2595.0, 2671.0, 2596.0, 2637.0, 2625.0, 2713.0, 2722.0, 2748.0, 2654.0, 2696.0, 2711.0, 2622.0, 2651.0, 2635.0, 2622.0, 2658.0, 2661.0, 2593.0, 2633.0, 2633.0, 2568.0, 2631.0, 2676.0, 2664.0, 2637.0, 2758.0, 2708.0, 2627.0, 2613.0, 2595.0, 2608.0, 2614.0, 2531.0, 2613.0, 2567.0, 2616.0, 2608.0, 2682.0, 2660.0, 2710.0, 2588.0, 2686.0, 2625.0, 2612.0, 2596.0, 2622.0, 2643.0, 2730.0, 2668.0, 2628.0, 2676.0, 2724.0, 2600.0, 2649.0, 2612.0, 2586.0, 2664.0, 2709.0, 2593.0, 2619.0, 2620.0, 2589.0, 2577.0, 2673.0, 2617.0, 2735.0, 2626.0, 2615.0, 2705.0, 2698.0, 2648.0, 2783.0, 2632.0, 2617.0, 2675.0, 2689.0, 2732.0, 2615.0, 2716.0, 2660.0, 2605.0, 2628.0, 2705.0, 2665.0, 2654.0, 2721.0, 2621.0, 2633.0, 2659.0, 2762.0, 2722.0, 2759.0, 2622.0, 2565.0, 2682.0, 2690.0, 2689.0, 2557.0, 2664.0, 2629.0, 2622.0, 2713.0, 2652.0, 2667.0, 2641.0, 2563.0, 2609.0, 2637.0, 2619.0, 2732.0, 2603.0, 2650.0, 2637.0, 2692.0, 2666.0, 2664.0, 2706.0, 2666.0, 2696.0, 2616.0, 2751.0, 2584.0, 2612.0, 2715.0, 2652.0, 2578.0, 2650.0, 2650.0, 2699.0, 2710.0, 2597.0, 2632.0, 2622.0, 2721.0, 2635.0, 2656.0, 2645.0, 2714.0, 2678.0, 2594.0, 2771.0, 2706.0, 2652.0, 2664.0, 2693.0, 2633.0, 2675.0, 2572.0, 2667.0, 2700.0, 2662.0]
  in  "stop":bool
  in  "Reset Average":bool=TRUE
  in  "Save Data?":bool=TRUE
  in  "Collect Data?":bool=TRUE
  in  "Tab Control":T2(tab)=enum."OD"
  out "Water Vapor Number Density  2":cluster{"Y":dbl[], "Y":dbl[]}[](graph)
  out "Absolute Humidity":cluster{"Y":dbl[], "Y":dbl[]}[](graph)
  out "NRB plot":cluster{"Y":dbl[], "Y":dbl[]}[](graph)
  in  "background length":i32=10
  out "Correction":cluster{"Y":dbl[], "Y":dbl[]}[](graph)
  in  "dead time":dbl=3.7e-08
  out "Optical Depth":cluster{"Y":dbl[], "Y":dbl[]}[](graph) caption="XY Graph"
  out "RingBuffer offline far":dbl[][](array[numeric])
  out "RingBuffer aerosol far":dbl[][](array[numeric])
  in  "Weather":T3(tab)=enum."Pulse Energy (Micro Joule)"
  out "Temperature (C)":dbl(graph)=21.93147130647131
  out "Pressure (mb)":dbl(graph)=836.0714285714286
  out "Relative Humdity (%)":dbl(graph)=18.27075702075702
  out "Pulse Energy (Micro Joule)":cluster{dbl}(graph)={5.057142857142857}
  in  "PRF (kHz)":dbl=7.0
  out "?":cluster{"mean":dbl, "mean":dbl}(graph)={"mean"=72800.0, "mean"=529280.0}
  out "Index":i32=13
  out "Aerosol Smoothed":dbl[](array[numeric])=[37200.06470588235, 28512.652941176468, 74.03529411764707, 76.38823529411766, 80.41764705882353, 86.91764705882353, 102.00588235294119, 125.1529411764706, 153.2117647058824, 174.6235294117647, 200.0058823529412, 231.0058823529412, 262.535294117647, 288.6823529411764, 308.47647058823526, 320.5941176470588, 331.15294117647056, 349.29999999999995, 354.00588235294117, 355.65294117647056, 362.15294117647056, 362.6823529411764, 359.65294117647056, 352.94705882352935, 346.44705882352935, 333.2411764705882, 320.8294117647058, 317.8294117647058, 302.38823529411764, 279.9176470588235, 267.6823529411764, 252.97647058823526, 237.15294117647056, 220.85882352941175, 208.71176470588236, 197.1529411764706, 181.8, 175.18235294117648, 167.77058823529416, 153.32941176470592, 140.53529411764708, 135.59411764705885, 129.5058823529412, 120.71176470588237, 114.3294117647059, 109.3294117647059, 103.77058823529414, 100.24117647058826, 95.30000000000001, 89.09411764705884, 85.21176470588236, 80.80000000000001, 76.18235294117648, 72.4764705882353, 67.24117647058824, 61.1235294117647, 60.358823529411765, 59.82941176470589, 55.858823529411765, 54.74117647058824, 54.59411764705882, 52.62352941176471, 48.06470588235294, 45.56470588235294, 44.77058823529411, 43.535294117647055, 41.417647058823526, 41.41764705882352, 41.15294117647059, 36.88823529411765, 33.535294117647055, 31.3, 30.564705882352943, 31.358823529411765, 30.711764705882352, 27.38823529411765, 24.38823529411765, 25.38823529411765, 26.68235294117647, 26.53529411764706, 23.91764705882353, 21.564705882352943, 22.094117647058823, 20.18235294117647, 20.947058823529414, 23.594117647058823, 21.88823529411765, 22.623529411764707, 21.329411764705885, 16.15294117647059, 14.094117647058825, 14.711764705882356, 17.094117647058823, 18.88823529411765, 18.535294117647062, 33.00588235294118, 129.71176470588236, 524.6529411764706, 1136.4764705882353, 1408.829411764706, 1143.358823529412, 660.8882352941176, 254.0647058823529, 51.41764705882354, 10.947058823529414, 9.623529411764707, 12.476470588235296, 19.00588235294118, 20.476470588235294, 16.358823529411765, 12.976470588235294, 12.094117647058825, 18.27058823529412, 22.711764705882352, 19.88823529411765, 15.711764705882356, 17.68235294117647, 30.623529411764707, 58.32941176470588, 84.21176470588236, 92.9764705882353, 81.38823529411766, 64.53529411764706, 66.8, 64.8, 89.56470588235294, 150.74117647058824, 159.06470588235294, 98.82941176470588, 49.47647058823529, 37.741176470588236, 37.682352941176475, 40.77058823529411, 32.1235294117647, 15.329411764705883, 6.505882352941178, 5.064705882352943, 4.888235294117648, 6.858823529411766, 4.829411764705884, -0.17058823529411588, 2.7117647058823544, 4.947058823529413, 4.829411764705884, 6.300000000000002, 3.182352941176472, 0.9764705882352959, 2.8000000000000016, 5.358823529411766, 3.829411764705884, 0.5058823529411782, -0.2882352941176453, 1.064705882352943, 2.711764705882355, 3.6529411764705895, 6.800000000000001, 8.182352941176472, 5.5352941176470605, 2.917647058823531, 4.4176470588235315, 3.5647058823529427, 2.1235294117647077, 2.682352941176472, 1.064705882352943, 1.8588235294117665, 1.65294117647059, 0.2117647058823547, -0.4058823529411747, -0.34705882352941, 0.4470588235294135, -0.6705882352941159, 0.5352941176470605, 2.7705882352941194, 0.5352941176470606, 0.5647058823529428, 1.8000000000000016, -0.25882352941176295, -1.3176470588235278, -0.6117647058823514, 3.2117647058823544, 5.976470588235296, 2.123529411764708, -0.023529411764704133, 1.3000000000000016, 0.47647058823529587, -0.25882352941176295, -3.405882352941175, -2.258823529411763, 1.1823529411764724, 0.8000000000000017, 1.8000000000000016, -1.7882352941176456, 0.12352941176470722, 7.6529411764705895, 4.917647058823531, 1.4176470588235313, 3.5647058823529427, 2.505882352941178, 1.4176470588235313, 2.4470588235294137, 1.3000000000000016, 1.241176470588237, 2.829411764705884, 3.6235294117647077, 1.2117647058823549, -0.6705882352941158, -0.25882352941176295, -1.1999999999999984, -2.9941176470588218, -2.0823529411764685, -0.994117647058822, 0.27058823529411924, 2.0058823529411782, 0.7705882352941195, 1.1529411764705901, 0.005882352941178226, -2.317647058823528, -0.22941176470588065, 2.711764705882355, 2.829411764705884, 1.5058823529411782, -0.14117647058823357, -0.3176470588235276, 2.7117647058823544, 4.2705882352941185, 5.211764705882354, 6.623529411764707, 3.388235294117649, 1.3882352941176488, 2.0941176470588254, 3.0647058823529427, 4.564705882352943, 4.6529411764705895, 3.447058823529413, 2.5058823529411782, 1.15294117647059, 1.9470588235294133, 2.594117647058825, -0.023529411764704078, -0.023529411764704078, 0.24117647058823707, -0.7294117647058805, -0.4941176470588218, 0.7705882352941194, -1.729411764705881, -1.1999999999999986, 4.858823529411766, 4.5352941176470605, 0.15294117647059002, 0.21176470588235496, 2.535294117647061, 2.0352941176470605, 2.094117647058825, 2.5352941176470605, 2.1235294117647077, 3.2705882352941194, 1.6235294117647077, -1.258823529411763, 0.27058823529411913, 1.1235294117647074, -1.9647058823529395, -3.582352941176469, -1.023529411764704, 1.3882352941176488, 0.65294117647059, 0.6529411764705898, -0.25882352941176323, -0.4058823529411748, -0.3470588235294101, -0.4647058823529395, 0.41764705882353115, -0.6411764705882335, -1.3764705882352923, -0.31764705882352773, 2.329411764705884, 0.38823529411764857, 1.0941176470588252]
  out "Off-Line  Bin Readings":dbl[](array[numeric])=[18072.0, 57957.0, 460.0, 432.0, 462.0, 409.0, 454.0, 443.0, 490.0, 482.0, 470.0, 483.0, 510.0, 546.0, 503.0, 559.0, 616.0, 550.0, 599.0, 564.0, 583.0, 599.0, 601.0, 606.0, 552.0, 563.0, 616.0, 619.0, 607.0, 623.0, 567.0, 537.0, 544.0, 506.0, 498.0, 541.0, 542.0, 505.0, 524.0, 554.0, 495.0, 491.0, 507.0, 484.0, 454.0, 456.0, 509.0, 457.0, 434.0, 440.0, 427.0, 495.0, 441.0, 430.0, 422.0, 434.0, 404.0, 404.0, 451.0, 393.0, 416.0, 406.0, 440.0, 391.0, 427.0, 423.0, 416.0, 437.0, 399.0, 449.0, 424.0, 372.0, 356.0, 389.0, 420.0, 408.0, 408.0, 398.0, 386.0, 385.0, 413.0, 406.0, 386.0, 377.0, 354.0, 401.0, 416.0, 403.0, 393.0, 395.0, 371.0, 369.0, 419.0, 420.0, 385.0, 354.0, 369.0, 882.0, 3021.0, 5190.0, 5929.0, 4898.0, 2564.0, 886.0, 387.0, 344.0, 348.0, 359.0, 378.0, 365.0, 376.0, 350.0, 391.0, 352.0, 383.0, 371.0, 351.0, 371.0, 382.0, 444.0, 463.0, 404.0, 403.0, 432.0, 434.0, 435.0, 484.0, 576.0, 546.0, 374.0, 364.0, 388.0, 364.0, 374.0, 384.0, 368.0, 361.0, 345.0, 377.0, 375.0, 359.0, 373.0, 389.0, 363.0, 394.0, 386.0, 366.0, 376.0, 358.0, 374.0, 365.0, 351.0, 349.0, 344.0, 370.0, 373.0, 398.0, 396.0, 379.0, 374.0, 380.0, 359.0, 361.0, 365.0, 365.0, 342.0, 364.0, 357.0, 321.0, 339.0, 385.0, 351.0, 355.0, 355.0, 355.0, 415.0, 390.0, 379.0, 354.0, 354.0, 391.0, 391.0, 365.0, 357.0, 340.0, 355.0, 389.0, 319.0, 348.0, 351.0, 363.0, 343.0, 344.0, 361.0, 399.0, 368.0, 353.0, 385.0, 383.0, 356.0, 368.0, 377.0, 386.0, 361.0, 368.0, 369.0, 335.0, 351.0, 325.0, 369.0, 344.0, 337.0, 372.0, 389.0, 373.0, 347.0, 360.0, 320.0, 389.0, 382.0, 352.0, 384.0, 356.0, 362.0, 383.0, 357.0, 377.0, 413.0, 346.0, 369.0, 360.0, 397.0, 381.0, 400.0, 393.0, 368.0, 363.0, 366.0, 394.0, 346.0, 383.0, 363.0, 398.0, 352.0, 346.0, 357.0, 368.0, 392.0, 372.0, 383.0, 347.0, 360.0, 381.0, 366.0, 356.0, 372.0, 371.0, 356.0, 349.0, 387.0, 355.0, 391.0, 361.0, 380.0, 368.0, 383.0, 381.0, 353.0, 363.0, 402.0, 375.0, 349.0, 361.0, 350.0, 342.0, 378.0, 346.0, 400.0, 337.0]
  out "Off-Line Smoothed":dbl[](array[numeric])=[37318.48516483516, 28568.595054945043, 72.0483516483517, 74.17884615384622, 84.30109890109898, 92.84093406593416, 102.44120879120888, 120.40274725274728, 147.23241758241755, 175.94945054945046, 206.38076923076915, 237.39313186813177, 264.77087912087893, 291.3354395604393, 316.207692307692, 338.2667582417579, 358.0923076923074, 374.6348901098898, 387.8491758241755, 397.47554945054924, 403.549725274725, 405.8615384615382, 405.1458791208789, 401.0950549450547, 392.6472527472524, 381.7489010989008, 370.08956043956016, 356.51813186813155, 339.5153846153843, 321.63351648351613, 304.3752747252744, 286.32307692307666, 269.7310439560438, 254.21868131868115, 237.50989010988997, 221.43983516483507, 207.01813186813177, 194.44807692307688, 182.3958791208791, 171.5167582417582, 159.19120879120877, 146.9563186813187, 138.01126373626374, 129.52087912087913, 121.69670329670332, 115.2461538461539, 109.7447802197803, 104.15824175824184, 98.2914835164836, 92.82994505494514, 88.85467032967043, 85.50714285714295, 81.19258241758249, 77.67884615384622, 74.54697802197809, 70.31071428571434, 66.75576923076929, 63.55521978021983, 60.780494505494545, 58.676098901098925, 56.28736263736266, 53.47829670329672, 50.471428571428596, 48.04835164835167, 46.06483516483518, 44.11291208791211, 42.7379120879121, 40.84368131868132, 39.00302197802198, 37.79148351648352, 35.73653846153846, 34.30796703296703, 32.739285714285714, 30.90137362637362, 30.242032967032955, 29.51675824175822, 28.688461538461517, 27.49203296703295, 26.261263736263718, 24.976923076923057, 23.902747252747236, 23.58543956043954, 22.946703296703276, 22.299725274725255, 21.707692307692287, 20.10604395604394, 18.960439560439546, 18.821703296703284, 18.470054945054933, 18.270879120879105, 17.328571428571415, 16.261263736263725, 16.215934065934057, 16.97280219780219, 19.29010989010988, 47.01675824175825, 365.0895604395605, 1051.5002747252747, 1483.4673076923073, 1279.6980769230768, 823.9631868131871, 458.2516483516483, 200.10604395604392, 56.29285714285714, 13.82994505494505, 8.540109890109889, 8.772252747252747, 9.726923076923075, 11.331318681318681, 12.373901098901095, 12.961813186813178, 18.42472527472526, 31.901373626373626, 51.71181318681323, 68.43983516483524, 69.73653846153856, 65.58681318681329, 67.92472527472536, 68.92197802197809, 60.68021978021982, 51.44120879120882, 49.21043956043958, 49.498901098901115, 47.31208791208793, 41.39725274725275, 43.310714285714276, 56.50439560439561, 55.33131868131869, 32.24340659340658, 14.524999999999997, 11.412362637362637, 11.691208791208787, 13.149999999999995, 12.460439560439559, 7.913736263736267, 4.275000000000003, 3.1458791208791244, 3.1760989010989062, 3.2777472527472575, 3.023626373626377, 2.525000000000002, 2.529120879120881, 2.185714285714287, 2.277747252747254, 2.9467032967032982, 2.70357142857143, 2.8354395604395624, 3.042857142857145, 2.6184065934065948, 2.242032967032968, 1.9824175824175838, 2.049725274725276, 2.257142857142859, 1.7942307692307708, 1.6293956043956053, 2.1870879120879128, 2.0675824175824187, 2.2489010989011, 2.1912087912087923, 1.431593406593407, 1.4934065934065934, 2.068956043956045, 2.7695054945054975, 1.6802197802197827, -0.005219780219780708, 0.2653846153846147, 1.077197802197802, 1.5263736263736263, 1.0332417582417586, 0.5359890109890115, 1.6458791208791212, 2.222802197802198, 2.046978021978022, 1.4631868131868127, 0.5208791208791199, 1.2159340659340652, 1.483791208791208, 1.0098901098901092, 1.1898351648351648, 1.5167582417582424, 1.3972527472527472, 1.2255494505494502, 1.5483516483516486, 1.5579670329670336, 1.2420329670329668, 1.2021978021978015, 0.5565934065934064, 0.10192307692307713, 0.5085164835164838, 0.6500000000000002, 1.228296703296704, 1.3697802197802205, 1.3890109890109892, 1.7214285714285715, 2.1280219780219785, 1.8107142857142857, 0.7969780219780216, 1.1087912087912086, 1.1184065934065934, 1.2241758241758238, 1.4384615384615382, 0.722802197802198, 0.3024725274725277, 0.07445054945054966, 0.2612637362637366, 0.5442307692307695, 1.0263736263736272, 0.40824175824175896, 0.19120879120879147, 1.2846153846153847, 1.4343406593406596, 0.6142857142857147, -0.14807692307692286, 0.3519230769230772, 0.6184065934065935, 0.4288461538461538, 0.05247252747252748, 0.5002747252747255, 1.3052197802197802, 1.0153846153846153, 0.8491758241758244, 0.4961538461538462, 0.5840659340659339, 1.0579670329670328, 0.37802197802197823, 0.14175824175824195, 0.4920329670329673, 0.7008241758241759, 1.6060439560439566, 1.7763736263736267, 1.1898351648351646, 1.2887362637362636, 0.6596153846153848, 0.659615384615384, 0.714560439560439, 0.12527472527472555, -0.002472527472527325, -0.3184065934065933, -0.10137362637362611, 0.7543956043956045, 1.3684065934065934, 0.0016483516483521976, -0.6096153846153842, 0.5524725274725276, 0.8656593406593407, 0.3587912087912086, 0.5538461538461539, 1.4741758241758247, 0.5538461538461543, -0.1412087912087909, 0.12664835164835195, 0.10741758241758262, 0.4769230769230771, 0.6802197802197805, 0.7131868131868135, -0.1494505494505492, -0.27032967032967004, 0.11153846153846178, -0.22912087912087886, 0.29697802197802237, 0.19807692307692343, -0.07252747252747227, 0.7118131868131871, 0.9164835164835167, 0.7516483516483518, 0.29697802197802214, 0.3010989010989011, 0.03598901098901092, -0.6178571428571428, -0.34725274725274713, -0.3898351648351647, -0.2524725274725272, -0.045054945054944756, -0.0024725274725272903, 0.18159340659340684, 0.4123626373626377, 0.29423076923076963]
  out "On-Line  Smoothed":dbl[](array[numeric])=[37948.59450549449, 29052.410439560423, 69.3870879120879, 67.46538461538461, 74.86236263736262, 78.16868131868128, 80.74148351648348, 88.49835164835159, 101.2483516483516, 116.38846153846148, 130.56703296703287, 141.25796703296692, 150.37747252747243, 158.11785714285708, 163.19752747252738, 167.80879120879112, 170.63571428571422, 170.66730769230762, 170.8170329670329, 170.5821428571428, 166.2552197802197, 160.05054945054934, 153.64395604395597, 146.13708791208785, 138.5107142857142, 130.37884615384607, 121.71675824175816, 113.02307692307687, 105.68791208791205, 98.5670329670329, 89.90357142857137, 83.11923076923074, 77.66181318681316, 71.48461538461538, 65.99835164835166, 61.04642857142858, 57.77445054945056, 55.2236263736264, 51.33489010989014, 46.85961538461541, 43.43653846153848, 40.856868131868154, 38.30741758241761, 35.85274725274728, 33.365109890109906, 31.458516483516497, 29.17967032967034, 28.006593406593417, 27.259340659340673, 25.428296703296716, 24.268956043956063, 23.484615384615402, 21.55054945054946, 20.164560439560447, 19.51346153846154, 19.005219780219782, 18.681043956043958, 17.182417582417585, 15.189285714285713, 14.404945054945053, 14.101373626373622, 13.856868131868126, 14.102747252747246, 13.029945054945047, 12.072527472527469, 11.507967032967025, 11.47912087912087, 10.976373626373618, 9.977747252747244, 9.71401098901098, 8.24423076923076, 8.268956043956036, 8.356868131868126, 6.832142857142851, 7.04505494505494, 8.414560439560434, 7.709890109890106, 6.836263736263733, 7.229120879120876, 6.6686813186813145, 6.039560439560437, 5.360989010989011, 5.025824175824177, 5.466758241758243, 5.21813186813187, 4.76346153846154, 4.760714285714286, 4.726373626373627, 4.435164835164837, 3.8362637362637386, 3.9104395604395625, 4.295054945054947, 4.204395604395606, 3.977747252747254, 4.171428571428573, 10.141208791208792, 81.0065934065934, 235.8239010989011, 335.5766483516484, 287.59725274725275, 181.43653846153842, 99.91456043956042, 43.75109890109891, 12.513461538461542, 3.420054945054947, 2.4543956043956072, 1.3980769230769245, 1.4392857142857152, 2.52857142857143, 3.225000000000001, 3.031318681318683, 3.6755494505494526, 6.810164835164832, 11.437912087912085, 14.984615384615388, 15.281318681318687, 14.296428571428578, 14.421428571428574, 15.110989010989012, 13.881593406593403, 11.415934065934056, 10.437912087912078, 10.692032967032956, 9.92967032967032, 8.78681318681318, 9.40906593406593, 11.796428571428569, 11.249725274725272, 6.661813186813186, 3.6521978021978043, 2.99835164835165, 2.6247252747252756, 2.5354395604395603, 2.4420329670329672, 1.5972527472527478, 1.1219780219780215, 0.653571428571428, 0.5010989010989009, 0.5285714285714284, 0.2758241758241757, 0.7799450549450548, 0.7799450549450548, 1.02032967032967, 1.5107142857142861, 1.352747252747253, 0.7620879120879119, 0.6824175824175821, 0.4859890109890106, 0.7662087912087913, 0.9832417582417583, 0.5560439560439557, 0.8211538461538458, 0.3967032967032964, -0.2214285714285716, -0.22417582417582435, 0.7895604395604392, 0.8596153846153842, -0.008516483516483812, -0.586813186813187, -0.4920329670329671, -0.03324175824175846, 0.6082417582417579, 1.1206043956043954, 0.4887362637362636, 0.05054945054945029, 0.5684065934065933, 0.07390109890109886, -0.2901098901098904, 0.35686813186813143, 0.6398351648351644, 0.5175824175824172, 0.3706043956043954, 0.8678571428571428, 0.6164835164835162, 0.09038461538461492, 0.4804945054945054, 0.8994505494505495, 0.9049450549450547, 0.47225274725274696, 0.0189560439560435, 0.42829670329670283, 0.39258241758241735, -0.1637362637362639, 0.11098901098901076, 0.31428571428571406, 0.7840659340659344, 0.7222527472527476, 0.8884615384615385, 0.8129120879120879, 0.1425824175824174, 0.12884615384615364, -0.3354395604395606, 0.07802197802197794, 0.16593406593406582, 0.45027472527472523, 0.264835164835165, -0.1307692307692307, 0.5478021978021976, 0.9392857142857141, 1.6412087912087916, 1.355494505494506, 1.1906593406593406, 1.3225274725274727, 0.3046703296703297, -0.18571428571428586, 0.25109890109890093, 0.3225274725274723, 0.13434065934065909, 0.27857142857142836, -0.09780219780219807, 0.21538461538461517, 0.420054945054945, -0.6912087912087913, -0.5414835164835166, 0.5368131868131868, 0.18653846153846138, 0.31291208791208774, 0.5848901098901098, -0.19807692307692312, -0.1925824175824176, 0.01620879120879103, -0.2653846153846156, 0.014835164835164671, 0.9159340659340658, 0.5642857142857142, 0.016208791208791234, 0.017582417582417603, 0.007967032967032828, -0.1664835164835166, 0.0697802197802197, 0.6604395604395603, -0.07994505494505505, -0.4467032967032969, -0.2832417582417585, 0.03956043956043953, 0.37747252747252746, -0.17197802197802217, -0.4906593406593408, -0.24065934065934086, -0.2695054945054946, -0.1609890109890112, 0.6576923076923074, 0.9365384615384611, 0.47637362637362607, -0.08269230769230788, -0.1678571428571433, 0.22499999999999945, 0.40906593406593394, 0.6686813186813187, -0.0620879120879122, -0.74478021978022, -0.847802197802198, -0.09505494505494527, 0.6824175824175822, 0.4502747252747251, -0.046978021978022144, 0.19890109890109886, 0.3925824175824175, -0.25576923076923097, 0.2799450549450548, 0.3348901098901098, 0.387087912087912, 0.4873626373626373, 0.4365384615384615, 0.1865384615384614, -0.16510989010989022, 0.23324175824175822, 0.1989010989010988, -0.5263736263736266, -0.5771978021978024, 0.2895604395604395, 0.2771978021978021, -0.1554945054945056, 0.37747252747252735, 0.7401098901098899, 0.42142857142857126, -0.6664835164835164]
  out "On-Line Bin Readings":dbl[](array[numeric])=[18414.0, 58735.0, 405.0, 441.0, 407.0, 421.0, 413.0, 430.0, 426.0, 464.0, 433.0, 470.0, 449.0, 471.0, 460.0, 459.0, 453.0, 484.0, 468.0, 431.0, 434.0, 471.0, 436.0, 428.0, 439.0, 481.0, 455.0, 477.0, 444.0, 410.0, 432.0, 406.0, 423.0, 440.0, 416.0, 413.0, 430.0, 445.0, 388.0, 396.0, 438.0, 401.0, 415.0, 419.0, 369.0, 387.0, 364.0, 405.0, 413.0, 381.0, 379.0, 412.0, 410.0, 391.0, 382.0, 413.0, 371.0, 408.0, 417.0, 348.0, 370.0, 351.0, 391.0, 389.0, 364.0, 370.0, 376.0, 375.0, 360.0, 370.0, 386.0, 384.0, 370.0, 375.0, 371.0, 373.0, 373.0, 363.0, 379.0, 363.0, 346.0, 394.0, 373.0, 344.0, 339.0, 406.0, 377.0, 379.0, 379.0, 409.0, 401.0, 357.0, 402.0, 387.0, 362.0, 353.0, 339.0, 419.0, 996.0, 1423.0, 1623.0, 1390.0, 867.0, 500.0, 346.0, 355.0, 357.0, 385.0, 380.0, 364.0, 378.0, 404.0, 405.0, 354.0, 380.0, 366.0, 381.0, 329.0, 385.0, 373.0, 350.0, 369.0, 371.0, 353.0, 371.0, 374.0, 392.0, 445.0, 429.0, 352.0, 377.0, 395.0, 369.0, 366.0, 342.0, 380.0, 356.0, 384.0, 360.0, 357.0, 396.0, 361.0, 376.0, 372.0, 335.0, 341.0, 380.0, 365.0, 368.0, 403.0, 387.0, 429.0, 362.0, 410.0, 377.0, 319.0, 329.0, 344.0, 371.0, 383.0, 378.0, 366.0, 356.0, 363.0, 353.0, 371.0, 387.0, 369.0, 374.0, 387.0, 369.0, 329.0, 368.0, 417.0, 322.0, 394.0, 378.0, 338.0, 369.0, 340.0, 352.0, 336.0, 359.0, 381.0, 384.0, 369.0, 351.0, 389.0, 397.0, 373.0, 394.0, 379.0, 350.0, 383.0, 350.0, 368.0, 380.0, 398.0, 377.0, 383.0, 414.0, 307.0, 374.0, 356.0, 354.0, 420.0, 369.0, 361.0, 373.0, 347.0, 385.0, 366.0, 373.0, 380.0, 364.0, 349.0, 373.0, 365.0, 347.0, 382.0, 379.0, 388.0, 412.0, 357.0, 369.0, 371.0, 380.0, 399.0, 351.0, 371.0, 370.0, 363.0, 371.0, 368.0, 366.0, 376.0, 370.0, 368.0, 348.0, 317.0, 378.0, 353.0, 367.0, 362.0, 363.0, 385.0, 389.0, 389.0, 376.0, 399.0, 378.0, 396.0, 354.0, 426.0, 364.0, 372.0, 322.0, 326.0, 366.0, 359.0, 359.0, 406.0, 364.0, 382.0, 377.0, 375.0, 356.0, 380.0, 363.0, 335.0, 340.0, 343.0, 364.0, 358.0, 366.0, 361.0, 355.0, 359.0, 351.0]
  out "Range Corrected Altitude Array":dbl[](array[numeric])=[5625.0, 22500.0, 50625.0, 90000.0, 140625.0, 202500.0, 275625.0, 360000.0, 455625.0, 562500.0, 680625.0, 810000.0, 950625.0, 1102500.0, 1265625.0, 1440000.0, 1625625.0, 1822500.0, 2030625.0, 2250000.0, 2480625.0, 2722500.0, 2975625.0, 3240000.0, 3515625.0, 3802500.0, 4100625.0, 4410000.0, 4730625.0, 5062500.0, 5405625.0, 5760000.0, 6125625.0, 6502500.0, 6890625.0, 7290000.0, 7700625.0, 8122500.0, 8555625.0, 9000000.0, 9455625.0, 9922500.0, 10400625.0, 10890000.0, 11390625.0, 11902500.0, 12425625.0, 12960000.0, 13505625.0, 14062500.0, 14630625.0, 15210000.0, 15800625.0, 16402500.0, 17015625.0, 17640000.0, 18275625.0, 18922500.0, 19580625.0, 20250000.0, 20930625.0, 21622500.0, 22325625.0, 23040000.0, 23765625.0, 24502500.0, 25250625.0, 26010000.0, 26780625.0, 27562500.0, 28355625.0, 29160000.0, 29975625.0, 30802500.0, 31640625.0, 32490000.0, 33350625.0, 34222500.0, 35105625.0, 36000000.0, 36905625.0, 37822500.0, 38750625.0, 39690000.0, 40640625.0, 41602500.0, 42575625.0, 43560000.0, 44555625.0, 45562500.0, 46580625.0, 47610000.0, 48650625.0, 49702500.0, 50765625.0, 51840000.0, 52925625.0, 54022500.0, 55130625.0, 56250000.0, 57380625.0, 58522500.0, 59675625.0, 60840000.0, 62015625.0, 63202500.0, 64400625.0, 65610000.0, 66830625.0, 68062500.0, 69305625.0, 70560000.0, 71825625.0, 73102500.0, 74390625.0, 75690000.0, 77000625.0, 78322500.0, 79655625.0, 81000000.0, 82355625.0, 83722500.0, 85100625.0, 86490000.0, 87890625.0, 89302500.0, 90725625.0, 92160000.0, 93605625.0, 95062500.0, 96530625.0, 98010000.0, 99500625.0, 101002500.0, 102515625.0, 104040000.0, 105575625.0, 107122500.0, 108680625.0, 110250000.0, 111830625.0, 113422500.0, 115025625.0, 116640000.0, 118265625.0, 119902500.0, 121550625.0, 123210000.0, 124880625.0, 126562500.0, 128255625.0, 129960000.0, 131675625.0, 133402500.0, 135140625.0, 136890000.0, 138650625.0, 140422500.0, 142205625.0, 144000000.0, 145805625.0, 147622500.0, 149450625.0, 151290000.0, 153140625.0, 155002500.0, 156875625.0, 158760000.0, 160655625.0, 162562500.0, 164480625.0, 166410000.0, 168350625.0, 170302500.0, 172265625.0, 174240000.0, 176225625.0, 178222500.0, 180230625.0, 182250000.0, 184280625.0, 186322500.0, 188375625.0, 190440000.0, 192515625.0, 194602500.0, 196700625.0, 198810000.0, 200930625.0, 203062500.0, 205205625.0, 207360000.0, 209525625.0, 211702500.0, 213890625.0, 216090000.0, 218300625.0, 220522500.0, 222755625.0, 225000000.0, 227255625.0, 229522500.0, 231800625.0, 234090000.0, 236390625.0, 238702500.0, 241025625.0, 243360000.0, 245705625.0, 248062500.0, 250430625.0, 252810000.0, 255200625.0, 257602500.0, 260015625.0, 262440000.0, 264875625.0, 267322500.0, 269780625.0, 272250000.0, 274730625.0, 277222500.0, 279725625.0, 282240000.0, 284765625.0, 287302500.0, 289850625.0, 292410000.0, 294980625.0, 297562500.0, 300155625.0, 302760000.0, 305375625.0, 308002500.0, 310640625.0, 313290000.0, 315950625.0, 318622500.0, 321305625.0, 324000000.0, 326705625.0, 329422500.0, 332150625.0, 334890000.0, 337640625.0, 340402500.0, 343175625.0, 345960000.0, 348755625.0, 351562500.0, 354380625.0, 357210000.0, 360050625.0, 362902500.0, 365765625.0, 368640000.0, 371525625.0, 374422500.0, 377330625.0, 380250000.0, 383180625.0, 386122500.0, 389075625.0, 392040000.0, 395015625.0, 398002500.0, 401000625.0, 404010000.0, 407030625.0, 410062500.0, 413105625.0, 416160000.0, 419225625.0, 422302500.0, 425390625.0, 428490000.0, 431600625.0, 434722500.0, 437855625.0, 441000000.0]
  out "Altitude Array (km)":dbl[](array[numeric])=[0.075, 0.15, 0.22499999999999998, 0.3, 0.375, 0.45, 0.5249999999999999, 0.6, 0.6749999999999999, 0.7499999999999999, 0.825, 0.8999999999999999, 0.9749999999999999, 1.05, 1.125, 1.2, 1.275, 1.3499999999999999, 1.4249999999999998, 1.5, 1.575, 1.65, 1.7249999999999999, 1.7999999999999998, 1.8749999999999998, 1.95, 2.025, 2.1, 2.1750000000000003, 2.25, 2.325, 2.4, 2.475, 2.5500000000000003, 2.625, 2.7, 2.775, 2.85, 2.9250000000000003, 3.0, 3.075, 3.15, 3.225, 3.3000000000000003, 3.375, 3.45, 3.525, 3.6, 3.675, 3.75, 3.825, 3.9, 3.975, 4.05, 4.125, 4.2, 4.275, 4.35, 4.425, 4.5, 4.575, 4.65, 4.725, 4.8, 4.875, 4.95, 5.025, 5.1, 5.175, 5.25, 5.325, 5.4, 5.475, 5.55, 5.625, 5.7, 5.775, 5.85, 5.925, 6.0, 6.075, 6.15, 6.225, 6.3, 6.375, 6.45, 6.525, 6.6, 6.675, 6.75, 6.825, 6.9, 6.975, 7.05, 7.125, 7.2, 7.2749999999999995, 7.35, 7.425, 7.5, 7.575, 7.6499999999999995, 7.725, 7.8, 7.875, 7.95, 8.024999999999999, 8.1, 8.174999999999999, 8.249999999999998, 8.325, 8.399999999999999, 8.475, 8.549999999999999, 8.624999999999998, 8.7, 8.774999999999999, 8.85, 8.924999999999999, 8.999999999999998, 9.075, 9.149999999999999, 9.225, 9.299999999999999, 9.374999999999998, 9.45, 9.524999999999999, 9.6, 9.674999999999999, 9.749999999999998, 9.825, 9.899999999999999, 9.975, 10.049999999999999, 10.124999999999998, 10.2, 10.274999999999999, 10.35, 10.424999999999999, 10.499999999999998, 10.575, 10.649999999999999, 10.725, 10.799999999999999, 10.874999999999998, 10.95, 11.024999999999999, 11.1, 11.174999999999999, 11.249999999999998, 11.325, 11.399999999999999, 11.475, 11.549999999999999, 11.624999999999998, 11.7, 11.774999999999999, 11.85, 11.924999999999999, 11.999999999999998, 12.075, 12.149999999999999, 12.225, 12.299999999999999, 12.374999999999998, 12.45, 12.524999999999999, 12.6, 12.674999999999999, 12.749999999999998, 12.825, 12.899999999999999, 12.975, 13.049999999999999, 13.124999999999998, 13.2, 13.274999999999999, 13.35, 13.424999999999999, 13.499999999999998, 13.575, 13.649999999999999, 13.725, 13.799999999999999, 13.874999999999998, 13.95, 14.024999999999999, 14.1, 14.174999999999999, 14.249999999999998, 14.325, 14.399999999999999, 14.474999999999998, 14.549999999999999, 14.624999999999998, 14.7, 14.774999999999999, 14.849999999999998, 14.924999999999999, 14.999999999999998, 15.075, 15.149999999999999, 15.224999999999998, 15.299999999999999, 15.374999999999998, 15.45, 15.524999999999999, 15.599999999999998, 15.674999999999999, 15.749999999999998, 15.825, 15.899999999999999, 15.974999999999998, 16.05, 16.125, 16.2, 16.275, 16.349999999999998, 16.424999999999997, 16.5, 16.575, 16.65, 16.724999999999998, 16.799999999999997, 16.875, 16.95, 17.025, 17.099999999999998, 17.174999999999997, 17.25, 17.325, 17.4, 17.474999999999998, 17.549999999999997, 17.625, 17.7, 17.775, 17.849999999999998, 17.924999999999997, 18.0, 18.075, 18.15, 18.224999999999998, 18.299999999999997, 18.375, 18.45, 18.525, 18.599999999999998, 18.674999999999997, 18.75, 18.825, 18.9, 18.974999999999998, 19.049999999999997, 19.125, 19.2, 19.275, 19.349999999999998, 19.424999999999997, 19.5, 19.575, 19.65, 19.724999999999998, 19.799999999999997, 19.875, 19.95, 20.025, 20.099999999999998, 20.174999999999997, 20.25, 20.325, 20.4, 20.474999999999998, 20.549999999999997, 20.625, 20.7, 20.775, 20.849999999999998, 20.924999999999997, 21.0]
  in  "Instrument Control":T4(tab)
  out "Readings":T5={"OnLineTEC"=19.5939884, "OnLineLD"=0.148085952, "OffLineTEC"=17.2781925, "OffLineLD"=0.152316406, "EtalonTEC"=27.988678, "TSOA-TEC"=18.008997, "Pro8000"=TRUE, "OnLine TEC"=TRUE, "OnLine LD"=TRUE, "OffLine TEC"=TRUE, "OffLine LD"=TRUE, "Etalon TEC"=TRUE, "TSOA TEC"=TRUE} {"OffLineLD" format="%.4g"; "OnLineLD" format="%.4g"; "TSOA-TEC" format="%.3g"; "EtalonTEC" format="%.3g"; "OffLineTEC" format="%.3g"; "OnLineTEC" format="%.3g"}
  in  "Settings":T6={"Module"=enum."On Line LD", "OnLineTEC"=19.62, "OnLineLD"=0.14788300000000185, "OffLineTEC"=17.28, "OffLineLD"=0.15256600000000475, "EtalonTEC"=28.0, "TSOA-TEC"=18.0} {"OffLineLD" min=0.0 max=0.175 step=0.001 format="%.3p"; "OnLineLD" min=0.0 max=0.175 step=0.001 format="%.3p"; "TSOA-TEC" format="%.2g"; "EtalonTEC" format="%.2g"; "OffLineTEC" min=0.0 max=30.0 step=0.1 format="%.2g"; "OnLineTEC" min=0.0 max=30.0 step=0.1 format="%.2g"}
  in  "Pulse B Polarity":enum32{"Low", "High"}(ring)=enum."High"
  in  "Pulse A Delay(ns)":u32=1040 min=80 max=327600
  in  "Pulse B Delay(ns)":u32=170000 min=80 max=327600 step=1
  in  "Accumulation Delay(ns)":u32=10 min=10 max=1270 step=1
  in  "Sync Pulse Polarity":enum32{"Low", "High"}(ring)=enum."High"
  in  "Pulse A Polarity":enum32{"Low", "High"}(ring)=enum."High"
  in  "Number of Bins":u32=280 min=2 max=4095 step=1
  in  "Number of Accumulates":u32=10000 min=1 max=32767 step=1
  in  "Time Resolution Per Bin(ns)":u32=500 min=5 max=1063 step=1
  out "WM Switch":bool
  in  "Cancel online":bool
  in  "Cancel Offline":bool
  in  "Lambda On Set (nm)":dbl=828.193 format="%.5f"
  out "Lambda On Read (nm)":dbl=828.1929805462469 format="%.5f"
  out "Lambda Off Read (nm)":dbl=828.2924989434316 format="%.5f"
  in  "Lambda Off Set (nm)":dbl=828.29245 format="%#.5f"
  in  "Bristol In":i32=5
  out "Bristol Out":i32=9
  in  "AB_DIF":dbl=5e-05 format="%#_15g"
  in  "NONAB_DIF":dbl=5e-05 format="%#_15g"
  out "Wavelength Lock Online":bool=TRUE
  out "Wavelength Lock Offline":bool=TRUE
  out "WL Difference":dbl=-1.94537531115202e-05 format="%_7g"
  out "WL Difference off":dbl=4.894343157957337e-05 format="%_7g"
  in  "calculate absorption cross sections":bool
  in  "Smoothing Range":dbl=150.0
  in  "Total DIAL Integration Time (Minutes)":i32=4
  in  "Data Reads (number of loops)":i32=1
  in  "Total Aerosol Integration Time (Minutes)":dbl=0.05
  in  "Scalar Wait Time":u32=1300
  out "Smoothed Bins":dbl=2.0
  out "OphirPM":T7={"Ophir-Ref"=refnum, "Ophir-Device"=1008, "Ophir-Channel"=0}
  out "Average Diode Power":dbl(knob)=0.00177 scale=0.0..0.002 scale format="%.1p"
  out "Ophir Samples":i32=24
  in  "Switch Comm Port":refnum<visa-resource-name>="COM3"
  out "FF_On_Ref":refnum<file>
  out "FF_On_Ptr":i64=64064 format="%.2p"
  out "FF_Off_Ref":refnum<file>
  out "FF_Off_Ptr":i64=64064 format="%.2p"
  out "NF_On_Ref":refnum<file>
  out "NF_On_Ptr":i64=64064 format="%.2p"
  out "NF_Off_Ref":refnum<file>
  out "NF_Off_Ptr":i64=64064 format="%.2p"
  out "DataOpen":bool=TRUE
  out "File Path_Far Field (out)":string="D:\\Micropulse_DIAL_data\\160216FF\\18"
  out "File Path_Near Field (out)":string="D:\\Micropulse_DIAL_data\\160216NF\\18"
  in  "Data File DIR (in)":string="D:\\Micropulse_DIAL_data\\"
  in  "WS visa":refnum<visa-resource-name>="LufftWS"
  out "TRHP":T8
  in  "bins":u32=280 min=2 max=4095 step=1
  out "y offset":u32=10
  in  "ns scale":u32=500
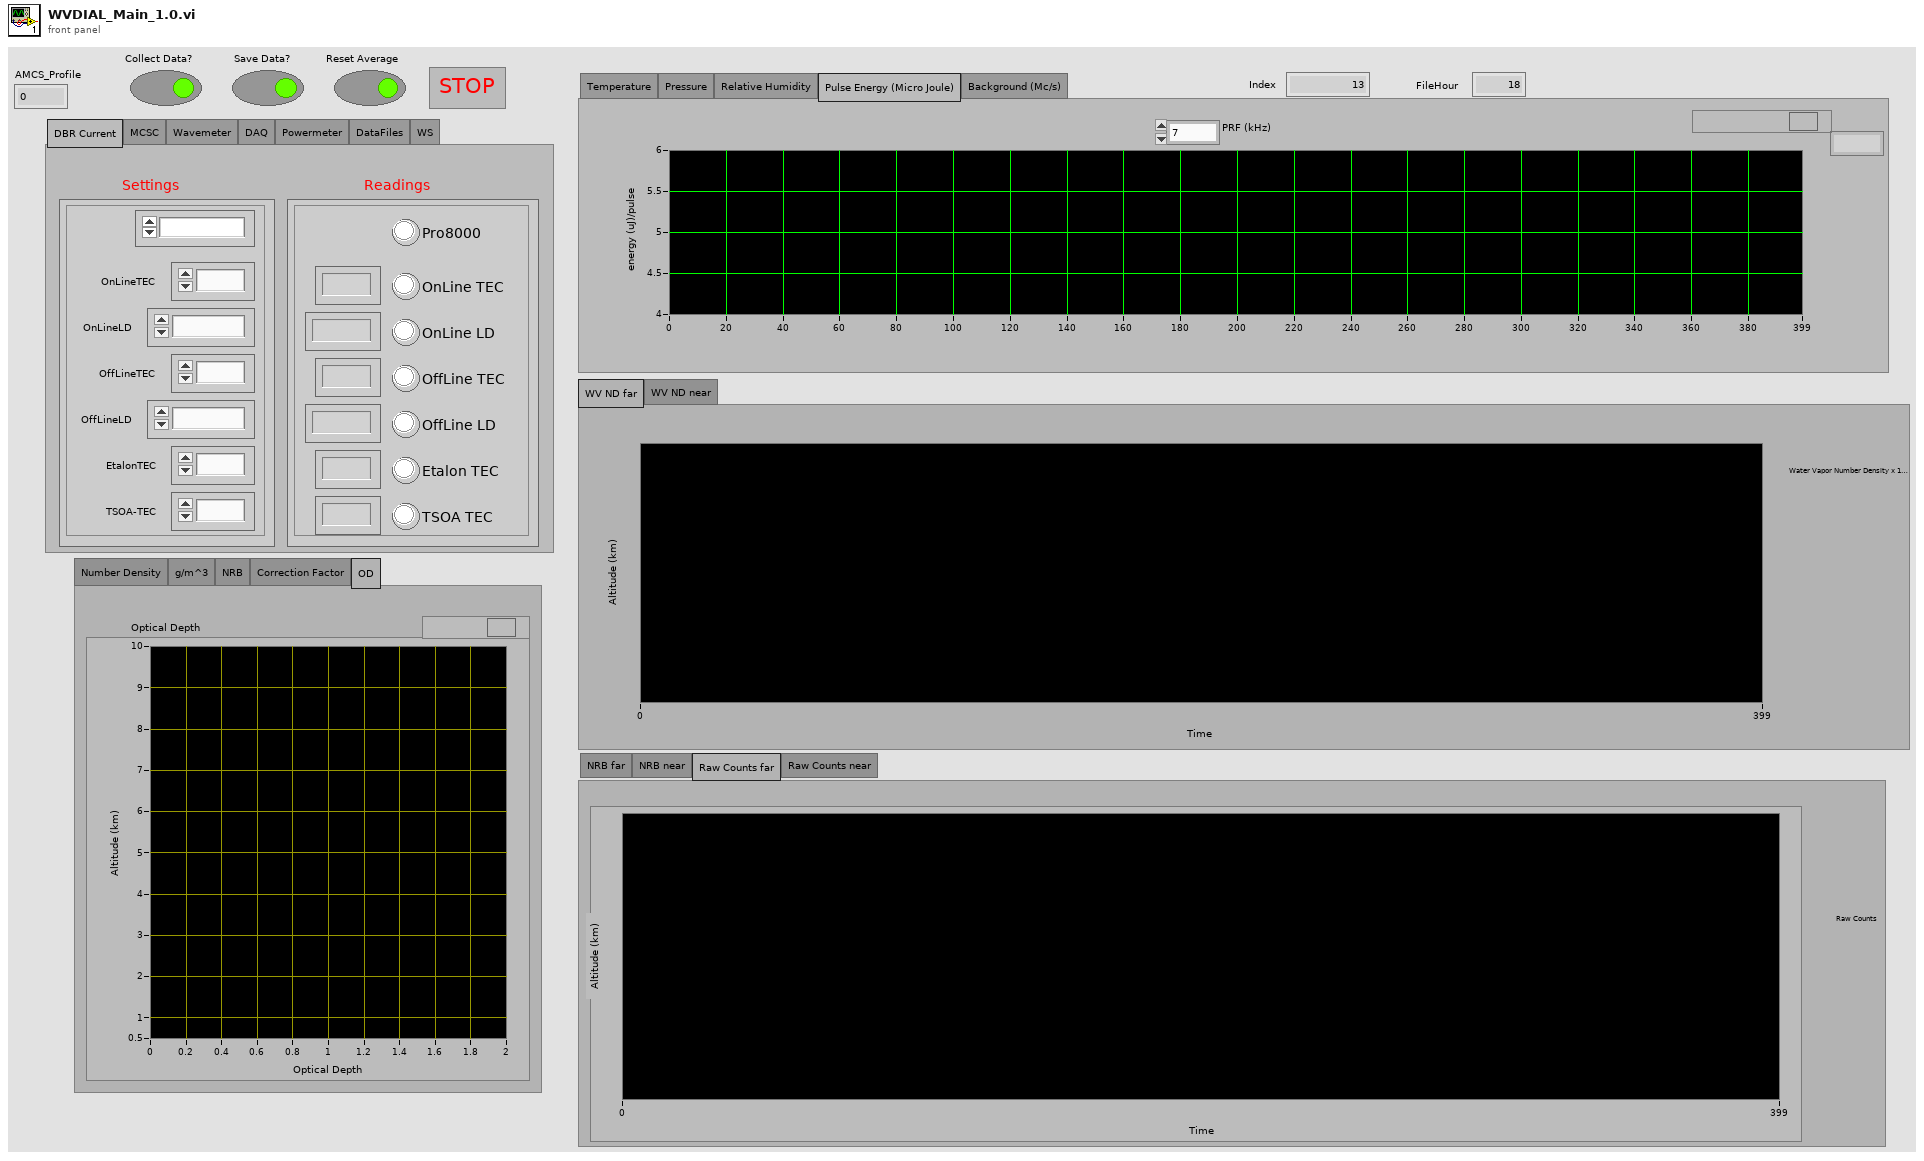
[diagram p1: front panel]
types:
  T1 = enum32{"NRB far", "NRB near", "Raw Counts far", "Raw Counts near"}
  T2 = enum32{"Number Density", "g/m^3", "NRB", "Correction Factor", "OD"}
  T3 = enum32{"Temperature", "Pressure", "Relative Humidity", "Pulse Energy (Micro Joule)", "Background (Mc/s)"}
  T4 = enum32{"DBR Current", "MCSC", "Wavemeter", "DAQ", "Powermeter", "DataFiles", "WS"}
  T5 = cluster{"OnLineTEC":dbl, "OnLineLD":dbl, "OffLineTEC":dbl, "OffLineLD":dbl, "EtalonTEC":dbl, "TSOA-TEC":dbl, "Pro8000":bool, "OnLine TEC":bool, "OnLine LD":bool, "OffLine TEC":bool, "OffLine LD":bool, "Etalon TEC":bool, "TSOA TEC":bool}
  T6 = cluster{"Module":enum16{"On Line TEC", "On Line LD", "Off Line TEC", "Off Line LD", "Etalon TEC", "TSOA TEC"}, "OnLineTEC":dbl, "OnLineLD":dbl, "OffLineTEC":dbl, "OffLineLD":dbl, "EtalonTEC":dbl, "TSOA-TEC":dbl}
  T7 = cluster{"Ophir-Ref":refnum<k7>, "Ophir-Device":i32, "Ophir-Channel":i32}
  T8 = cluster{"Temp":dbl, "RelH":dbl, "Press":dbl, "AbH":dbl}
  T9 = enum16{"Open_TL", "Close_TL", "Verify_ID", "TEC_Sensor", "SET", "READ", "ON", "OFF", "Set_Limits", "Read_Limits", "Enable_Status", "Read_Status"}
  T10 = enum16{"open", "replace", "create", "open or create", "replace or create", "replace or create with confirmation"}
  T11 = enum16{"On Line TEC", "On Line LD", "Off Line TEC", "Off Line LD", "Etalon TEC", "TSOA TEC"}
  T12 = typedef "LVDateTimeRec.ctl" = cluster{"fractional second":dbl, "second":i32, "minute":i32, "hour":i32, "day of month":i32, "month":i32, "year":i32, "day of week":i32, "day of year":i32, "DST":i32}
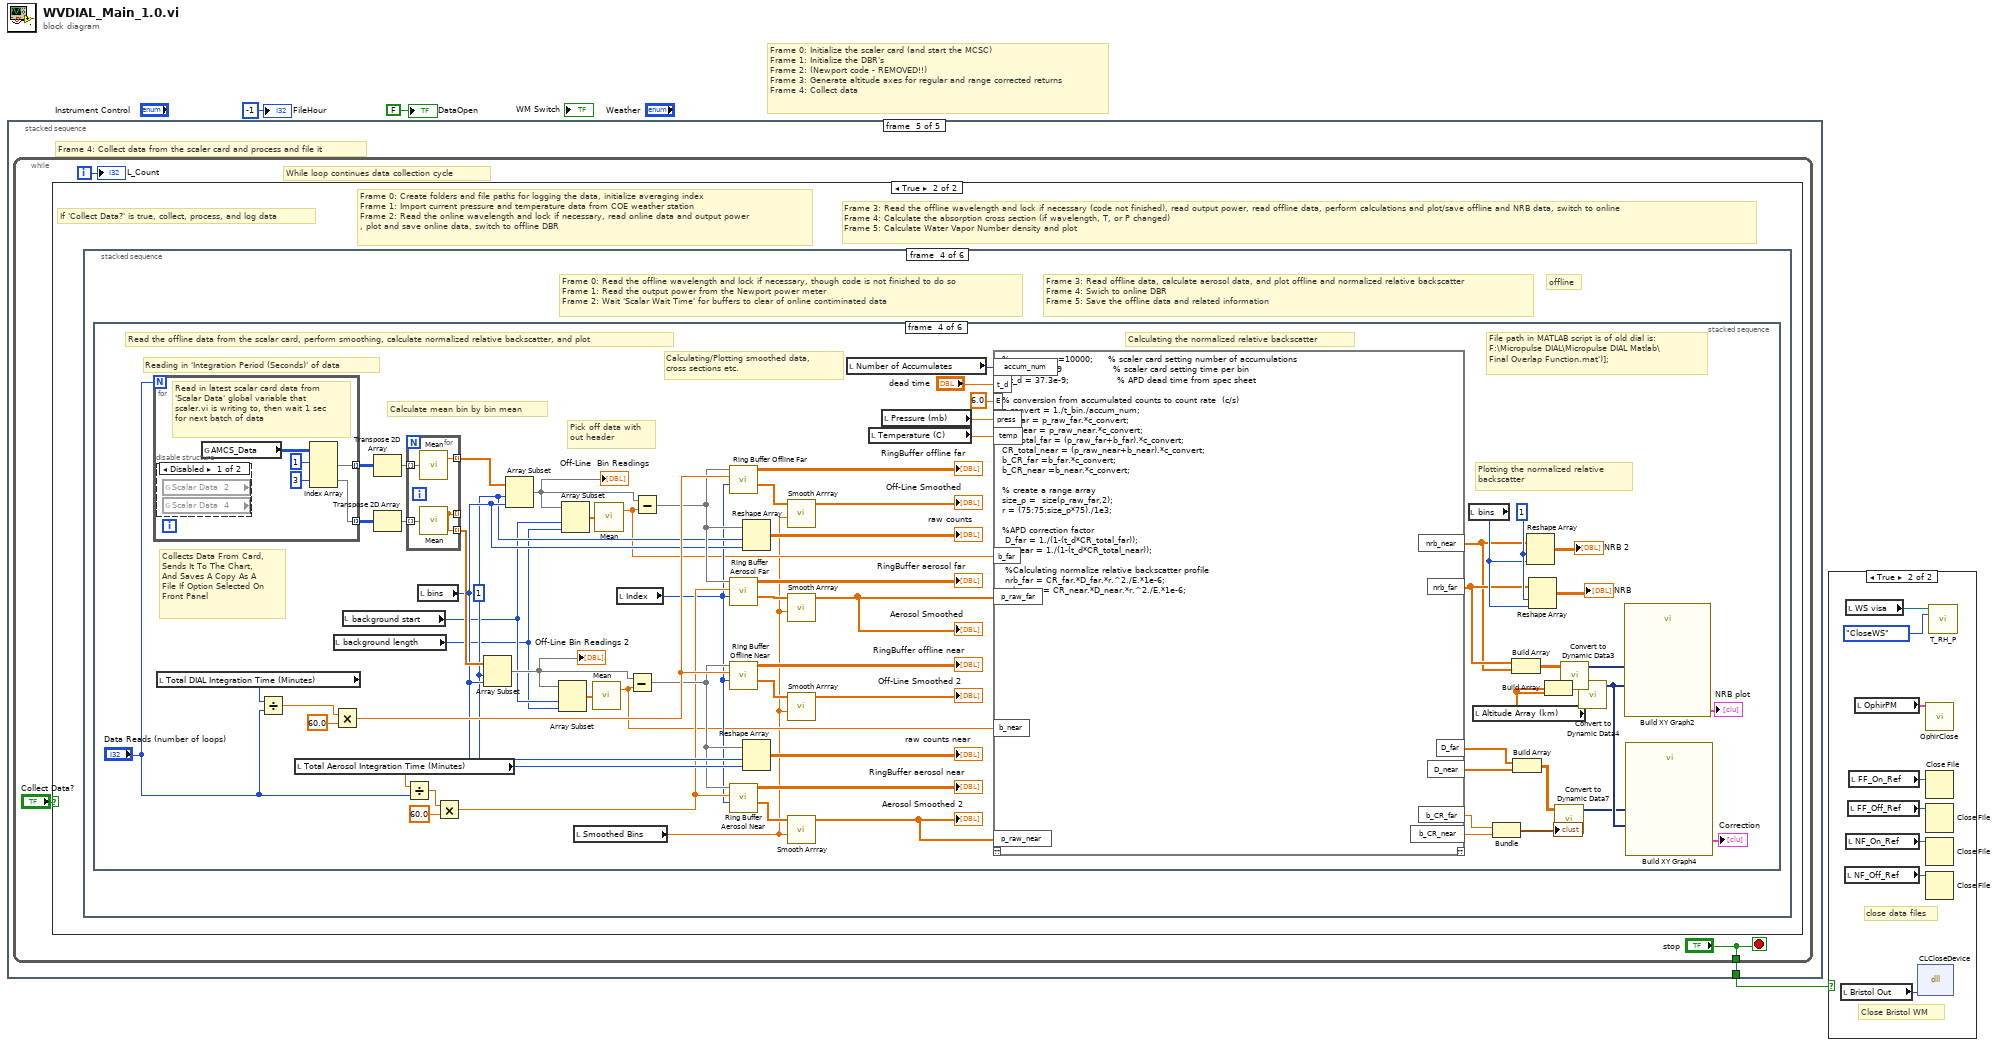
[diagram p0: block diagram]
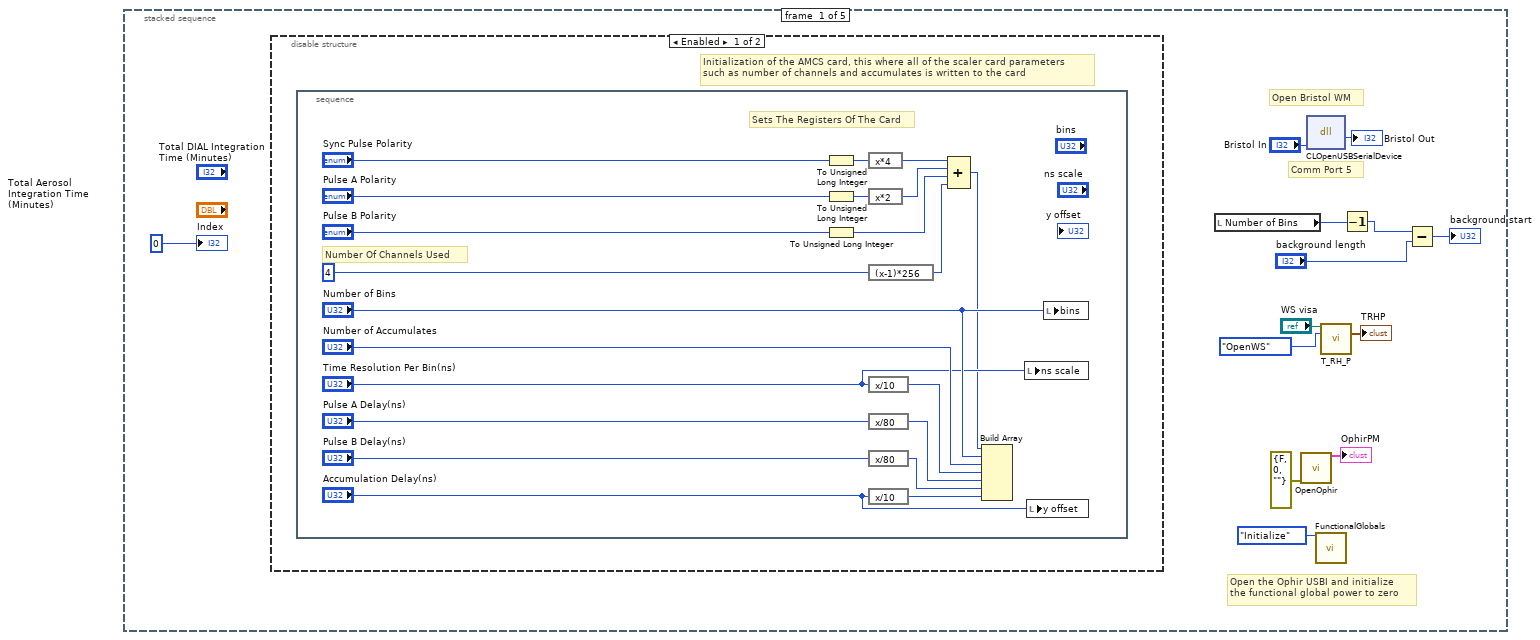
[diagram p3: hidden frame]
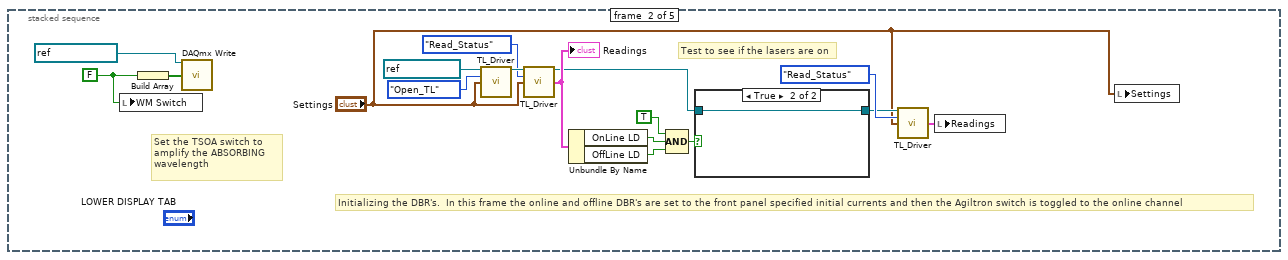
[diagram p5: hidden frame]
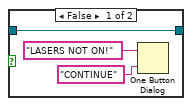
[diagram p6: hidden frame]
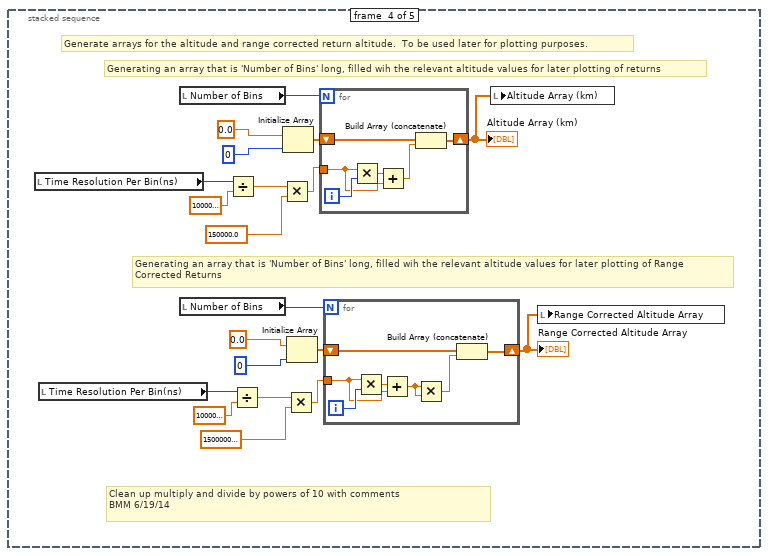
[diagram p8: hidden frame]
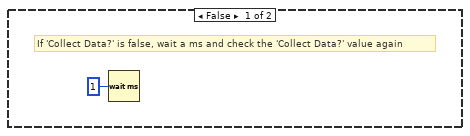
[diagram p9: hidden frame]
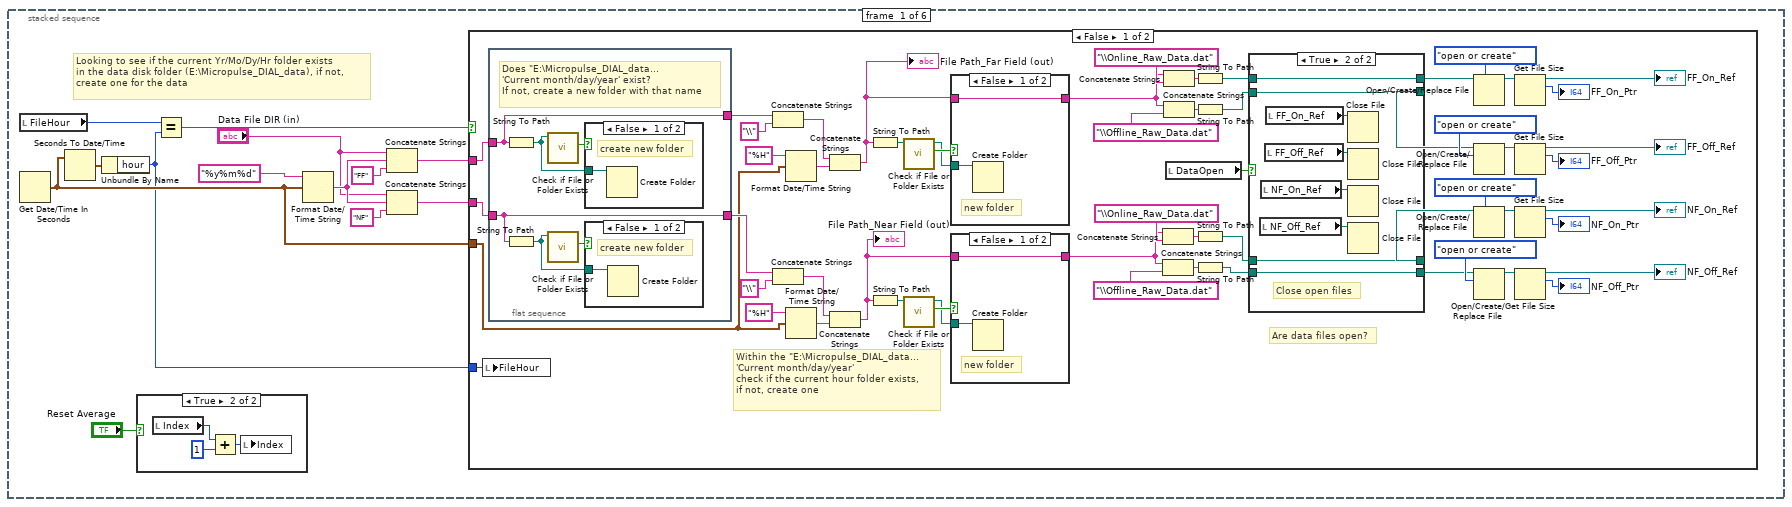
[diagram p10: hidden frame]
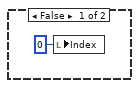
[diagram p17: hidden frame]
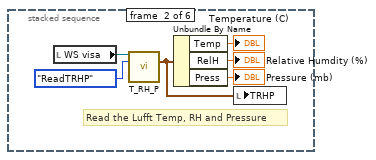
[diagram p18: hidden frame]
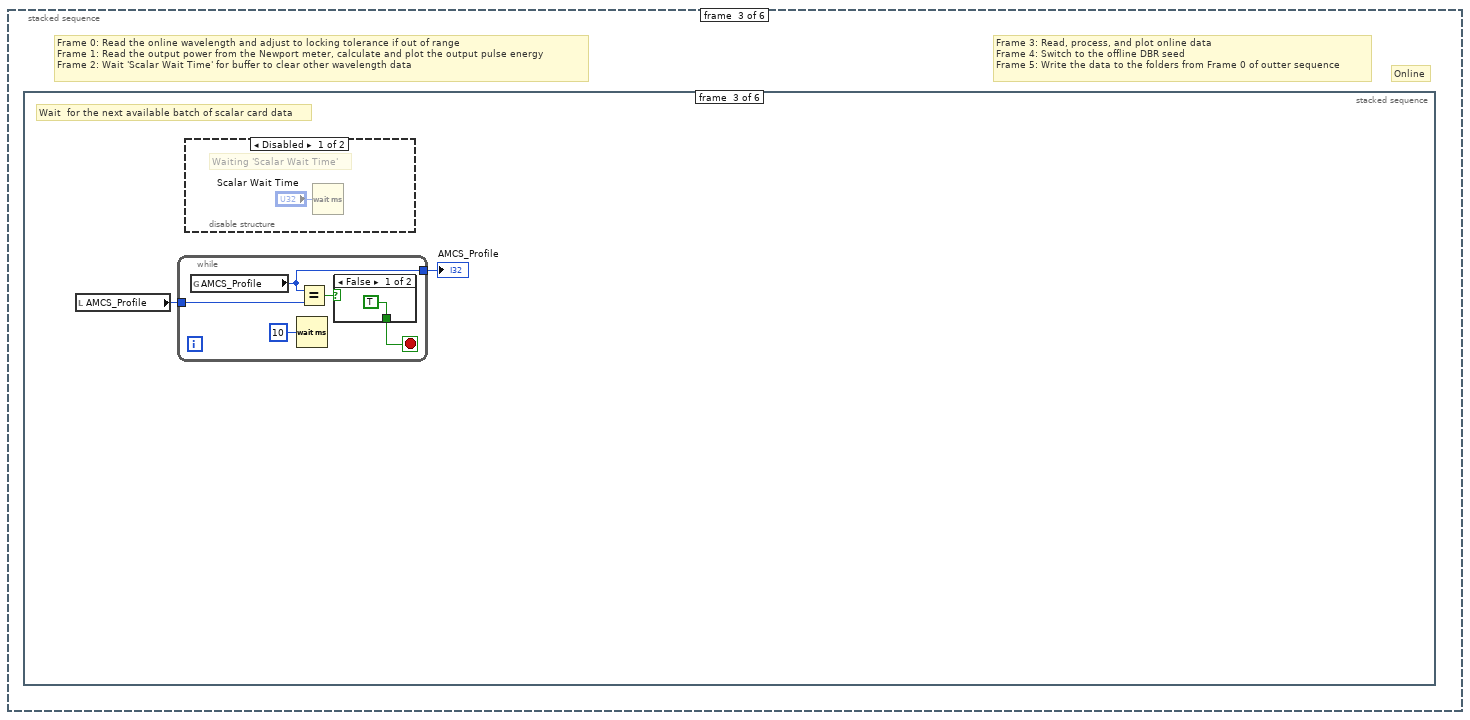
[diagram p19: hidden frame]
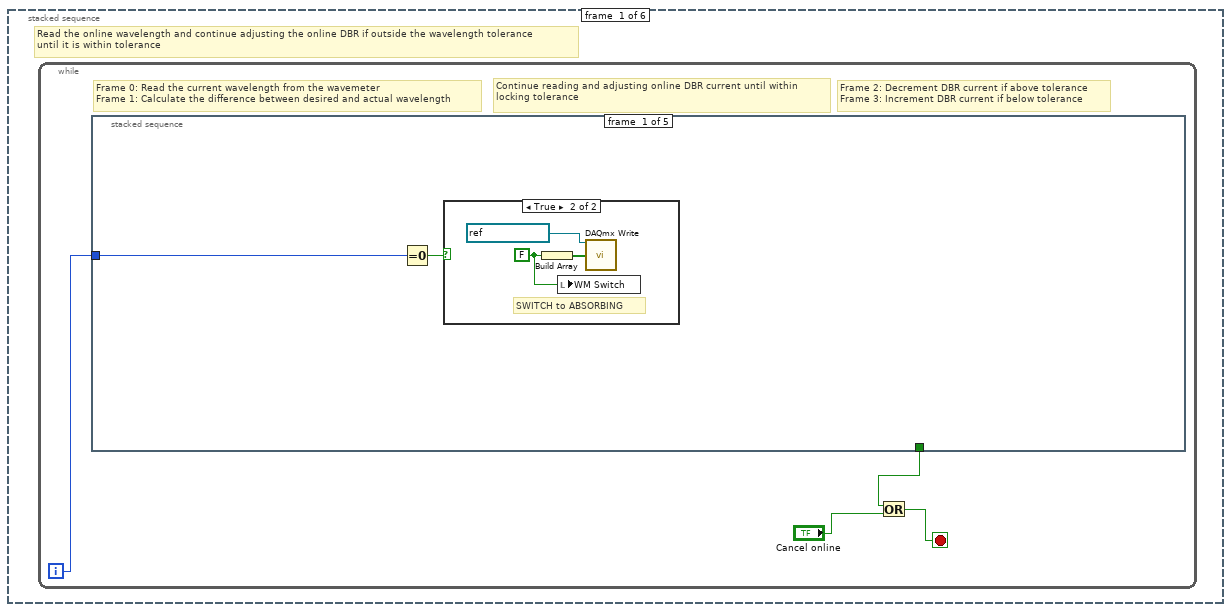
[diagram p20: hidden frame]
diagram:
  # "Frame 0: Initialize the scaler card (and start the MCSC)\nFrame 1: Initialize the DBR's\nFrame 2: (Newport code - REMOVED!!)\nFrame 3: Generate altitude axes for regular and range corrected returns\nFrame 4: Collect data"
  n1 = stacked-sequence {
    tunnel: [_ _ _ _ w92] -> w3
    frame #0 {
      # "Open the Ophir USBI and initialize\nthe functional global power to zero"
      # "Comm Port 5"
      # "Open Bristol WM"
      n2 = disable-structure shown="Enabled" {
        frame Enabled {
          # "Initialization of the AMCS card, this where all of the scaler card parameters\nsuch as number of channels and accumulates is written to the card"
          n3 = stacked-sequence {
            frame #0 {
              # "Sets The Registers Of The Card"
              # "Number Of Channels Used"
              n4 = To Unsigned Long Integer(number="Sync Pulse Polarity") -> (unsigned 32bit integer=w17:u32)
              n5 = To Unsigned Long Integer(number="Pulse A Polarity") -> (unsigned 32bit integer=w21:u32)
              n6 = To Unsigned Long Integer(number="Pulse B Polarity") -> (unsigned 32bit integer=w19:u32)
              n7 = expression code="x*4"(w17) -> (w26:u32)
              n8 = expression code="x*2"(w21) -> (w25:u32)
              n9 = expression code="(x-1)*256"(u32 4 ("Number of Channels Used")) -> (w24:u32)
              n10 = expression code="x/10"("Time Resolution Per Bin(ns)") -> (w28:u32)
              n11 = expression code="x/80"("Pulse A Delay(ns)") -> (w35:u32)
              n12 = expression code="x/80"("Pulse B Delay(ns)") -> (w37:u32)
              n13 = expression code="x/10"("Accumulation Delay(ns)") -> (w36:u32)
              n14 = Compound Arithmetic op=ADD(w26, w25, w19, w24) -> (w23:u32)
              n15 = Build Array(w23, "Number of Bins", "Number of Accumulates", w28, w35, w37, w36) -> ()  [unwired: 1 out]
              n16 = local write "ns scale"("Time Resolution Per Bin(ns)") -> ()
              n17 = local write "y offset"("Accumulation Delay(ns)") -> ()
              n18 = local write "bins"("Number of Bins") -> ()
            }
          }
        }
        frame Disabled {
        }
      }
      n19 = local read "Number of Bins"() -> (w13:u32)
      n20 = call "OpenOphir.vi"("error in (no error)"=errorcluster {"status"=FALSE, "code"=0, "source"=""}) -> ("OphirPM"=→"OphirPM":T7)  [unwired: 13 in, 1 out]
      n21 = dll-call lib="C:/H2O_DIAL/LabVIEW-2012/Bristol WM V2_31b/CLDevIface.dll" fn="CLOpenUSBSerialDevice"("commPort"="Bristol In") -> ("return type"=→"Bristol Out":i32)  [unwired: 4 in, 2 out]
      n22 = call "FunctionalGlobals.vi"("FG_Control"=enum16{"Initialize", "PowerRead", "PowerWrite"}."Initialize") -> ()  [unwired: 14 in, 1 out]
      n23 = call "T_RH_P.vi"("VISA in"="WS visa", "WS_Commands"=enum16{"OpenWS", "ReadTRHP", "CloseWS"}."OpenWS") -> ("TRHP"=→"TRHP":T8)  [unwired: 11 in, 2 out]
      n24 = Decrement(x=w13) -> (x-1=w12:u32)
      n25 = Subtract(x=w12, y="background length") -> (x-y=→"background start":u32)
      "Index" <- 0 ("Index")
    }
    frame #1 {
      w38 = FALSE ("Boolean")
      # "Test to see if the lasers are on"
      # "Set the TSOA switch to\namplify the ABSORBING\nwavelength"
      # "Initializing the DBR's.  In this frame the online and offline DBR's are set to the front panel specified initial currents and then the Agiltron switch is toggled to the online channel"
      n26 = local write "WM Switch"(w38) -> ()
      n27 = Build Array(w38) -> (w40:bool[])
      n28 = call-poly <vilib>:"DAQmx Write.vi"("task/channels in"=refnum<k21> "BristolWM", "data"=w40) -> ()  [unwired: 11 in, 3 out]
      n29 = call "TL_Driver.vi"("Device In"=refnum<visa-resource-name> "ThorLabs", "Commands"=T9."Open_TL", "Settings"="Settings") -> ("Device Out"=w52:refnum<visa-resource-name>)  [unwired: 9 in, 3 out]
      n30 = call "TL_Driver.vi"("Device In"=w52, "Commands"=T9."Read_Status", "Settings"="Settings") -> ("Device Out"=w49:refnum<visa-resource-name>, "Readings"=w50:T5)  [unwired: 9 in, 2 out]
      "Readings" <- w50
      n31 = Unbundle By Name(w50) -> ("OnLine LD"=w44:bool, "OffLine LD"=w45:bool)
      n32 = Compound Arithmetic op=AND(TRUE, w44, w45) -> (w43:bool)
      n33 = case shown="True" w43 {
        tunnel: w49 -> [w55 w58]
        tunnel: [w55 w58] -> w47
        frame False {
          n34 = One Button Dialog(message="LASERS NOT ON!", button name ("OK")="CONTINUE") -> ()  [unwired: 1 out]
        }
        frame True {
        }
      }
      n35 = call "TL_Driver.vi"("Device In"=w47, "Commands"=T9."Read_Status", "Settings"="Settings") -> ("Readings"=w39:T5)  [unwired: 9 in, 3 out]
      n36 = local write "Readings"(w39) -> ()
      n37 = local write "Settings"("Settings") -> ()
    }
    frame #2 {
      # "NEWPORT CODE REMOVED!!!!"
    }
    frame #3 {
      # "Clean up multiply and divide by powers of 10 with comments\nBMM 6/19/14"
      # "Generating an array that is 'Number of Bins' long, filled wih the relevant altitude values for later plotting of Range \nCorrected Returns"
      # "Generating an array that is 'Number of Bins' long, filled wih the relevant altitude values for later plotting of returns"
      # "Generate arrays for the altitude and range corrected return altitude.  To be used later for plotting purposes."
      n38 = local read "Time Resolution Per Bin(ns)"() -> (w71:u32)
      n39 = local read "Time Resolution Per Bin(ns)"() -> (w61:u32)
      n40 = local read "Number of Bins"() -> (w74:u32)
      n41 = local read "Number of Bins"() -> (w64:u32)
      n42 = Divide(x=w71, y=1000000000.0) -> (x/y=w69:dbl)
      n43 = Divide(x=w61, y=1000000000.0) -> (x/y=w59:dbl)
      n44 = Multiply(x=w69, y=150000.0) -> (x*y=w72:dbl)
      n45 = Initialize Array(0.0, 0) -> (w77:dbl[])
      n46 = Multiply(x=w59, y=150000000.0) -> (x*y=w62:dbl)
      n47 = Initialize Array(0.0, 0) -> (w67:dbl[])
      n48 = for {
        N: w74 -> [_]
        shift-right: [w90] -> w75
        shift-left: w77 -> [w91]
        tunnel: w72 -> [w87]
        i -> [w89]
        n49 = Multiply(x=w87, y=w89) -> (x*y=w88:dbl)
        n50 = Add(x=w88, y=w87) -> (x+y=w86:dbl)
        n51 = Build Array (concatenate)(w91, w86) -> (w90:dbl[])
      }
      "Altitude Array (km)" <- w75
      n52 = for {
        N: w64 -> [_]
        shift-right: [w84] -> w65
        shift-left: w67 -> [w85]
        tunnel: w62 -> [w80]
        i -> [w83]
        n53 = Multiply(x=w80, y=w83) -> (x*y=w81:dbl)
        n54 = Add(x=w81, y=w80) -> (x+y=w79:dbl)
        n55 = Multiply(x=w79, y=w79) -> (x*y=w82:dbl)
        n56 = Build Array (concatenate)(w85, w82) -> (w84:dbl[])
      }
      "Range Corrected Altitude Array" <- w65
      n57 = local write "Altitude Array (km)"(w75) -> ()
      n58 = local write "Range Corrected Altitude Array"(w65) -> ()
    }
    frame #4 {
      # "Frame 4: Collect data from the scaler card and process and file it"
      n59 = while {
        tunnel: ["stop"] -> w92
        i -> [w93]
        stop <- "stop" stop-if-true
        # "While loop continues data collection cycle"
        n60 = case shown="True" "Collect Data?" {
          frame False {
            # "If 'Collect Data?' is false, wait a ms and check the 'Collect Data?' value again"
            n61 = Wait (ms)(milliseconds to wait=u32 1) -> ()  [unwired: 1 out]
          }
          frame True {
            # "Frame 3: Read the offline wavelength and lock if necessary (code not finished), read output power, read offline data, perform calculations and plot/save offline and NRB data, switch to online\nFrame 4: Calculate the absorption cross section (if wavelength, T, or P changed)\nFrame 5: Calculate Water Vapor Number density and plot"
            # "Frame 0: Create folders and file paths for logging the data, initialize averaging index\nFrame 1: Import current pressure and temperature data from COE weather station\nFrame 2: Read the online wavelength and lock if necessary, read online data and output power\n, plot and save online data, switch to offline DBR"
            # "If 'Collect Data?' is true, collect, process, and log data"
            n62 = stacked-sequence {
              frame #0 {
                # "Looking to see if the current Yr/Mo/Dy/Hr folder exists\nin the data disk folder (E:\\Micropulse_DIAL_data), if not,\ncreate one for the data"
                n63 = local read "FileHour"() -> (w106:i32)
                n64 = Get Date/Time In Seconds() -> (seconds since 1Jan1904=w98:timestamp)
                n65 = Seconds To Date/Time(time stamp (now)=w98) -> (date time rec=w108:T12)  [unwired: 1 in]
                n66 = Unbundle By Name(w108) -> ("hour"=w97:i32)
                n67 = case shown="True" "Reset Average" {
                  frame False {
                    n68 = local write "Index"(0 ("Index")) -> ()
                  }
                  frame True {
                    n69 = local read "Index"() -> (w196:i32)
                    n70 = Add(x=w196, y=1) -> (x+y=w195:i32)
                    n71 = local write "Index"(w195) -> ()
                  }
                }
                n72 = Equal?(x=w106, y=w97) -> (x = y?=w107:bool)
                n73 = Format Date/Time String(time format string (%c)="%y%m%d", seconds (now)=w98) -> (date/time string=w102:string)  [unwired: 1 in]
                n74 = Concatenate Strings("Data File DIR (in)", w102, "FF" ("string")) -> (w104:string)
                n75 = Concatenate Strings("Data File DIR (in)", w102, "NF" ("string")) -> (w99:string)
                n76 = case shown="False" w107 {
                  tunnel: w104 -> [w166 _]
                  tunnel: w99 -> [w165 _]
                  tunnel: w98 -> [w152 _]
                  tunnel: w97 -> [w128 _]
                  frame False {
                    # "Are data files open?"
                    # "Within the \"E:\\Micropulse_DIAL_data...\n'Current month/day/year' \ncheck if the current hour folder exists,\nif not, create one"
                    n77 = local write "FileHour"(w128) -> ()
                    n78 = flat-sequence {
                      tunnel: [w186] -> w153
                      tunnel: w166 -> [w185]
                      tunnel: w165 -> [w186]
                      tunnel: [w185] -> w154
                      frame #0 {
                        # "Does \"E:\\Micropulse_DIAL_data...\n'Current month/day/year' exist?\nIf not, create a new folder with that name"
                        n79 = String To Path(string=w185) -> (path=w190:path)
                        n80 = String To Path(string=w186) -> (path=w188:path)
                        n81 = call <vilib>:"Check if File or Folder Exists.vi"("path"=w190) -> ("file or folder exists?"=w189:bool)  [unwired: 8 in, 2 out]
                        n82 = call <vilib>:"Check if File or Folder Exists.vi"("path"=w188) -> ("file or folder exists?"=w187:bool)  [unwired: 8 in, 2 out]
                        n83 = case shown="False" w189 {
                          tunnel: w190 -> [w192 _]
                          frame False {
                            # "create new folder"
                            n84 = Create Folder(path (use dialog)=w192) -> ()  [unwired: 2 in, 3 out]
                          }
                          frame True {
                            # "Folder exists\ndo nothing"
                          }
                        }
                        n85 = case shown="False" w187 {
                          tunnel: w188 -> [w191 _]
                          frame False {
                            # "create new folder"
                            n86 = Create Folder(path (use dialog)=w191) -> ()  [unwired: 2 in, 3 out]
                          }
                          frame True {
                            # "Folder exists\ndo nothing"
                          }
                        }
                      }
                    }
                    n87 = Concatenate Strings(w154, "\\" ("string")) -> (w161:string)
                    n88 = Concatenate Strings(w153, "\\" ("string")) -> (w156:string)
                    n89 = Format Date/Time String(time format string (%c)="%H", seconds (now)=w152) -> (date/time string=w164:string)  [unwired: 1 in]
                    n90 = Format Date/Time String(time format string (%c)="%H", seconds (now)=w152) -> (date/time string=w159:string)  [unwired: 1 in]
                    n91 = Concatenate Strings(w161, w164) -> (w124:string)
                    "File Path_Far Field (out)" <- w124
                    n92 = Concatenate Strings(w156, w159) -> (w125:string)
                    "File Path_Near Field (out)" <- w125
                    n93 = String To Path(string=w124) -> (path=w162:path)
                    n94 = String To Path(string=w125) -> (path=w157:path)
                    n95 = call <vilib>:"Check if File or Folder Exists.vi"("path"=w162) -> ("file or folder exists?"=w151:bool, "dup path"=w149:path)  [unwired: 8 in, 1 out]
                    n96 = call <vilib>:"Check if File or Folder Exists.vi"("path"=w157) -> ("file or folder exists?"=w150:bool, "dup path"=w148:path)  [unwired: 8 in, 1 out]
                    n97 = case shown="False" w151 {
                      tunnel: w149 -> [w183 _]
                      tunnel: w124 -> [w182 w184]
                      tunnel: [w182 w184] -> w122
                      frame False {
                        # "new folder"
                        n98 = Create Folder(path (use dialog)=w183) -> ()  [unwired: 2 in, 3 out]
                      }
                      frame True {
                        # "Folder exists\ndo nothing"
                      }
                    }
                    n99 = case shown="False" w150 {
                      tunnel: w148 -> [w180 _]
                      tunnel: w125 -> [w179 w181]
                      tunnel: [w179 w181] -> w123
                      frame False {
                        # "new folder"
                        n100 = Create Folder(path (use dialog)=w180) -> ()  [unwired: 2 in, 3 out]
                      }
                      frame True {
                        # "Folder exists\ndo nothing"
                      }
                    }
                    n101 = Concatenate Strings(w123, "\\Online_Raw_Data.dat" ("string")) -> (w142:string)
                    n102 = Concatenate Strings(w123, "\\Offline_Raw_Data.dat" ("string")) -> (w141:string)
                    n103 = Concatenate Strings(w122, "\\Online_Raw_Data.dat" ("string")) -> (w147:string)
                    n104 = Concatenate Strings(w122, "\\Offline_Raw_Data.dat" ("string")) -> (w146:string)
                    n105 = local read "DataOpen"() -> (w139:bool)
                    n106 = String To Path(string=w147) -> (path=w138:path)
                    n107 = String To Path(string=w146) -> (path=w137:path)
                    n108 = String To Path(string=w142) -> (path=w136:path)
                    n109 = String To Path(string=w141) -> (path=w135:path)
                    n110 = case shown="True" w139 {
                      tunnel: w138 -> [w170 w174]
                      tunnel: [w170 w174] -> w132
                      tunnel: w137 -> [w169 w173]
                      tunnel: [w169 w173] -> w131
                      tunnel: w136 -> [w168 w172]
                      tunnel: [w168 w172] -> w130
                      tunnel: [w167 w171] -> w129
                      tunnel: w135 -> [w167 w171]
                      frame False {
                        # "No files open\ndo nothing"
                      }
                      frame True {
                        # "Close open files"
                        n111 = local read "NF_Off_Ref"() -> (w176:refnum<file>)
                        n112 = local read "NF_On_Ref"() -> (w175:refnum<file>)
                        n113 = local read "FF_Off_Ref"() -> (w178:refnum<file>)
                        n114 = local read "FF_On_Ref"() -> (w177:refnum<file>)
                        n115 = Close File(refnum=w177) -> ()  [unwired: 1 in, 2 out]
                        n116 = Close File(refnum=w178) -> ()  [unwired: 1 in, 2 out]
                        n117 = Close File(refnum=w175) -> ()  [unwired: 1 in, 2 out]
                        n118 = Close File(refnum=w176) -> ()  [unwired: 1 in, 2 out]
                      }
                    }
                    n119 = Open/Create/Replace File(file path (use dialog)=w132, operation (0:open)=T10."open or create") -> (refnum out=w118:refnum<file>)  [unwired: 4 in, 2 out]
                    n120 = Open/Create/Replace File(file path (use dialog)=w131, operation (0:open)=T10."open or create") -> (refnum out=w119:refnum<file>)  [unwired: 4 in, 2 out]
                    n121 = Open/Create/Replace File(file path (use dialog)=w130, operation (0:open)=T10."open or create") -> (refnum out=w120:refnum<file>)  [unwired: 4 in, 2 out]
                    n122 = Open/Create/Replace File(file path (use dialog)=w129, operation (0:open)=T10."open or create") -> (refnum out=w121:refnum<file>)  [unwired: 4 in, 2 out]
                    n123 = Get File Size(file=w118) -> (refnum out=→"FF_On_Ref":refnum<file>, size (in bytes)=→"FF_On_Ptr":i64)  [unwired: 1 in, 1 out]
                    n124 = Get File Size(file=w119) -> (refnum out=→"FF_Off_Ref":refnum<file>, size (in bytes)=→"FF_Off_Ptr":i64)  [unwired: 1 in, 1 out]
                    n125 = Get File Size(file=w120) -> (refnum out=→"NF_On_Ref":refnum<file>, size (in bytes)=→"NF_On_Ptr":i64)  [unwired: 1 in, 1 out]
                    n126 = Get File Size(file=w121) -> (refnum out=→"NF_Off_Ref":refnum<file>, size (in bytes)=→"NF_Off_Ptr":i64)  [unwired: 1 in, 1 out]
                  }
                  frame True {
                    # "Don't need to do anything!"
                  }
                }
              }
              frame #1 {
                # "Read the Lufft Temp, RH and Pressure"
                n127 = local read "WS visa"() -> (w202:refnum<visa-resource-name>)
                n128 = call "T_RH_P.vi"("VISA in"=w202, "WS_Commands"=enum16{"OpenWS", "ReadTRHP", "CloseWS"}."ReadTRHP") -> ("TRHP"=w197:T8)  [unwired: 11 in, 2 out]
                n129 = Unbundle By Name(w197) -> ("Temp"=→"Temperature (C)":dbl, "RelH"=→"Relative Humdity (%)":dbl, "Press"=→"Pressure (mb)":dbl)
                n130 = local write "TRHP"(w197) -> ()
              }
              frame #2 {
                # "Frame 3: Read, process, and plot online data\nFrame 4: Switch to the offline DBR seed\nFrame 5: Write the data to the folders from Frame 0 of outter sequence"
                # "Frame 0: Read the online wavelength and adjust to locking tolerance if out of range\nFrame 1: Read the output power from the Newport meter, calculate and plot the output pulse energy\nFrame 2: Wait 'Scalar Wait Time' for buffer to clear other wavelength data"
                # "Online"
                n131 = stacked-sequence {
                  frame #0 {
                    # "Read the online wavelength and continue adjusting the online DBR if outside the wavelength tolerance\nuntil it is within tolerance"
                    n132 = while {
                      i -> [w206]
                      stop <- w204 stop-if-true
                      # "Frame 2: Decrement DBR current if above tolerance\nFrame 3: Increment DBR current if below tolerance"
                      # "Frame 0: Read the current wavelength from the wavemeter\nFrame 1: Calculate the difference between desired and actual wavelength"
                      # "Continue reading and adjusting online DBR current until within locking tolerance"
                      n133 = stacked-sequence {
                        tunnel: w206 -> [w208 _ _ _ _]
                        tunnel: [_ _ w215 _ _] -> w205
                        frame #0 {
                          n134 = Equal To 0?(x=w208) -> (x = 0?=w207:bool)
                          n135 = case shown="True" w207 {
                            frame False {
                            }
                            frame True {
                              w209 = FALSE ("Boolean")
                              # "SWITCH to ABSORBING"
                              n136 = Build Array(w209) -> (w210:bool[])
                              n137 = local write "WM Switch"(w209) -> ()
                              n138 = call-poly <vilib>:"DAQmx Write.vi"("task/channels in"=refnum<k21> "BristolWM", "data"=w210) -> ()  [unwired: 11 in, 3 out]
                            }
                          }
                        }
                        frame #1 {
                          # "Read Bristol WM"
                          n139 = local read "Bristol Out"() -> (w212:i32)
                          n140 = dll-call lib="C:/H2O_DIAL/LabVIEW-2012/Bristol WM V2_31b/CLDevIface.dll" fn="CLGetLambdaReading"("devHandle"=w212) -> ("return type"=→"Lambda On Read (nm)":dbl)  [unwired: 4 in, 2 out]
                        }
                        frame #2 {
                          # "If WL difference is within tolerance, stop looping, and illuminate 'Wavelength Lock Online' indicator"
                          # "Calculating the difference between the actual and desired online wavelength"
                          n141 = local read "Lambda On Read (nm)"() -> (w222:dbl)
                          n142 = local read "AB_DIF"() -> (w219:dbl)
                          n143 = Subtract(x=w222, y="Lambda On Set (nm)") -> (x-y=w214:dbl)
                          "WL Difference" <- w214
                          n144 = Multiply(x=-1.0, y=w219) -> (x*y=w220:dbl)
                          n145 = Greater?(x=w214, y=w220) -> (0:w216:bool)
                          n146 = Less?(x=w214, y=w219) -> (x < y?=w217:bool)
                          n147 = And(x=w216, y=w217) -> (x .and. y?=w215:bool)
                          "Wavelength Lock Online" <- w215
                        }
                        frame #3 {
                          # "If the wavelength difference is greater that 0.0002 nm, decrement the \nDBR current by 0.01 mA"
                          n148 = local read "WL Difference"() -> (w225:dbl)
                          n149 = Greater Or Equal?(x=w225, y="AB_DIF") -> (x >= y?=w223:bool)
                          n150 = case shown="True" w223 {
                            frame False {
                              # "Wavelength difference is not greater than 0.0002 nm, do nothing"
                            }
                            frame True {
                              # "Generating a command string\nto decrement the current"
                              # "WL difference is greater than 0.0002 nm,\ndecrement the DBR current by 0.01 mA"
                              n151 = local read "Settings"() -> (w230:T6)
                              n152 = Unbundle By Name(w230) -> ("OnLineLD"=w232:dbl)
                              n153 = Subtract(x=w232, y=3e-06) -> (x-y=w233:dbl)
                              n154 = Bundle By Name(cluster=w230, "OnLineLD"=w233, "Module"=T11."On Line LD") -> (w228:T6)
                              n155 = call "TL_Driver.vi"("Device In"=refnum<visa-resource-name> "ThorLabs", "Commands"=T9."SET", "Settings"=w228) -> ("Readings"=w226:T5)  [unwired: 9 in, 3 out]
                              n156 = local write "Settings"(w228) -> ()
                              n157 = local write "Readings"(w226) -> ()
                            }
                          }
                        }
                        frame #4 {
                          # "If the wavelength difference is less that 0.0002 nm, increment the \nDBR current by 0.01 mA"
                          n158 = local read "WL Difference"() -> (w239:dbl)
                          n159 = local read "AB_DIF"() -> (w237:dbl)
                          n160 = Multiply(x=-1.0, y=w237) -> (x*y=w235:dbl)
                          n161 = Less Or Equal?(x=w239, y=w235) -> (x <= y?=w238:bool)
                          n162 = case shown="True" w238 {
                            frame False {
                              # "WL difference is no <= to -0.0002 nm, do nothing"
                            }
                            frame True {
                              # "WL difference is < -0.0002,\nincrement the DBR current by 0.01 mA"
                              # "Generating a command string\nto decrement the current"
                              n163 = local read "Settings"() -> (w244:T6)
                              n164 = Unbundle By Name(w244) -> ("OnLineLD"=w246:dbl)
                              n165 = Add(x=w246, y=3e-06) -> (x+y=w247:dbl)
                              n166 = Bundle By Name(cluster=w244, "OnLineLD"=w247, "Module"=T11."On Line LD") -> (w241:T6)
                              n167 = call "TL_Driver.vi"("Device In"=refnum<visa-resource-name> "ThorLabs", "Commands"=T9."SET", "Settings"=w241) -> ("Readings"=w240:T5)  [unwired: 9 in, 3 out]
                              n168 = local write "Settings"(w241) -> ()
                              n169 = local write "Readings"(w240) -> ()
                            }
                          }
                        }
                      }
                      n170 = Or(x=w205, y="Cancel online") -> (x .or. y?=w204:bool)
                    }
                  }
                  frame #1 {
                    # "Plotting the online and offling pulse energies"
                    # "Converting to pulse energy, assumes 5 percent pickoff"
                    # "Reading the output power of the laser transmitter from the Ophir power meter, once read, convert to corresponding pulse energy and plot"
                    n171 = local read "OphirPM"() -> (w253:T7)
                    n172 = call "OphirRead.vi"("OphirPM"=w253) -> ("Power (W)"=w249:dbl, "Ophir Samples"=→"Ophir Samples":i32)  [unwired: 12 in, 1 out]
                    "Average Diode Power" <- w249
                    n173 = Multiply(x=w249, y=1000.0) -> (x*y=w257:dbl)
                    n174 = Divide(x=w257, y=0.05) -> (x/y=w255:dbl)
                    n175 = Divide(x=w255, y="PRF (kHz)") -> (x/y=w250:dbl)
                    n176 = Bundle(w250) -> (→"Pulse Energy (Micro Joule)":cluster{dbl})  [unwired: 1 in]
                  }
                  frame #2 {
                    # "Wait  for the next available batch of scalar card data"
                    n177 = local read "AMCS_Profile"() -> (w259:i32)
                    n178 = while {
                      tunnel: [w266] -> w260
                      tunnel: w259 -> [w262]
                      stop <- w264 stop-if-true
                      n179 = global read "AMCS_Data.vi" "AMCS_Profile"() -> (w266:i32)
                      n180 = Wait (ms)(milliseconds to wait=u32 10) -> ()  [unwired: 1 out]
                      n181 = Equal?(x=w266, y=w262) -> (x = y?=w265:bool)
                      n182 = case shown="False" w265 {
                        tunnel: [TRUE FALSE] -> w264
                        frame False {
                        }
                        frame True {
                        }
                      }
                    }
                    "AMCS_Profile" <- w260
                    n183 = disable-structure shown="Disabled" {
                      frame Disabled {
                        # "Waiting 'Scalar Wait Time'"
                        n184 = Wait (ms)(milliseconds to wait="Scalar Wait Time") -> ()  [unwired: 1 out]
                      }
                      frame Enabled {
                      }
                    }
                  }
                  frame #3 {
                    # "convert time per range bin to meters\nand calculate smoothed bins using\nsmoothing range"
                    # "Plotting online cross section and smoothed online data"
                    # "Calculate the bin by bin mean of the data"
                    # "Collect 'Integration Period (Seconds)' number\nof scalar data"
                    # "Reading, processing, and plotting the online data"
                    n185 = local read "Data Reads (number of loops)"() -> (w294:i32)
                    n186 = for {
                      N: w294 -> [_]
                      tunnel: [w314] -> w306 mode=indexing
                      tunnel: [w315] -> w286 mode=indexing
                      # "Scalar Data is retrieved from Global \nVariable that scaler.vi is writing to,"
                      n187 = disable-structure shown="Disabled" {
                        frame Disabled {
                          n188 = global read "Scalar_Data.vi" "Scalar Data  3"() -> ()  [unwired: 1 out]
                          n189 = global read "Scalar_Data.vi" "Scalar Data"() -> ()  [unwired: 1 out]
                        }
                        frame Enabled {
                        }
                      }
                      n190 = global read "AMCS_Data.vi" "AMCS_Data"() -> (w317:u16[][])
                      n191 = Index Array(array=w317, index (row) #2=2 ("index (row)")) -> (element #1=w314:u16[], element #2=w315:u16[])  [unwired: 3 in]
                    }
                    n192 = Transpose 2D Array(2D array=w306) -> (transposed array=w310:u16[][])
                    n193 = Transpose 2D Array(2D array=w286) -> (transposed array=w292:u16[][])
                    n194 = for {
                      tunnel: w310 -> [w319] mode=indexing
                      tunnel: [w318] -> w311 mode=indexing
                      n195 = call-poly <vilib>:"Mean.vi"("X"=w319) -> ("mean"=w318:dbl)  [unwired: 1 out]
                    }
                    n196 = for {
                      tunnel: w292 -> [w313] mode=indexing
                      tunnel: [w312] -> w293 mode=indexing
                      n197 = call-poly <vilib>:"Mean.vi"("X"=w313) -> ("mean"=w312:dbl)  [unwired: 1 out]
                    }
                    n198 = local read "bins"() -> (w285:u32)
                    n199 = Array Subset(array=w311, index=1 ("dimension size"), length=w285) -> (w298:dbl[])
                    n200 = Array Subset(array=w293, index=1 ("dimension size"), length=w285) -> (w290:dbl[])
                    n201 = local read "background length"() -> (w275:i32)
                    n202 = local read "background start"() -> (w276:u32)
                    n203 = Array Size(array=w298) -> (size(s)=w295:i32)
                    n204 = Array Size(array=w290) -> (size(s)=w287:i32)
                    n205 = Initialize Array(1.0 ("element"), w295) -> (w297:dbl[])
                    n206 = Initialize Array(1.0 ("element"), w287) -> (w289:dbl[])
                    n207 = Multiply(x=w298, y=w297) -> (x*y=w299:dbl[])
                    "On-Line Bin Readings" <- w299
                    n208 = Multiply(x=w290, y=w289) -> (x*y=w279:dbl[])
                    "On-Line Bin Readings 2" <- w279
                    n209 = local read "Total DIAL Integration Time (Minutes)"() -> (w302:i32)
                    n210 = local read "Time Resolution Per Bin(ns)"() -> (w271:u32)
                    n211 = Array Subset(array=w299, index=w276, length=w275) -> (w308:dbl[])
                    n212 = Array Subset(array=w279, index=w276, length=w275) -> (w281:dbl[])
                    n213 = call-poly <vilib>:"Mean.vi"("X"=w308) -> ("mean"=w307:dbl)  [unwired: 1 out]
                    n214 = call-poly <vilib>:"Mean.vi"("X"=w281) -> ("mean"=w282:dbl)  [unwired: 1 out]
                    n215 = Divide(x=w302, y=w294) -> (x/y=w300:dbl)
                    n216 = local read "Index"() -> (w280:i32)
                    n217 = Subtract(x=w299, y=w307) -> (x-y=w304:dbl[])
                    n218 = Subtract(x=w279, y=w282) -> (x-y=w283:dbl[])
                    n219 = To Double Precision Float(number=w271) -> (double precision float=w272:dbl)
                    n220 = Multiply(x=w300, y=60.0) -> (x*y=w277:dbl)
                    n221 = Multiply(x=w272, y=0.15) -> (x*y=w274:dbl)
                    n222 = call "Ring Buffer Online Far.vi"("Index"=w280, "Profiles to Average"=w277, "Input Array"=w304) -> ("AvgArray"=w303:dbl[])  [unwired: 7 in, 1 out]
                    n223 = call "Ring Buffer Online Near.vi"("Index"=w280, "Profiles to Average"=w277, "Input Array"=w283) -> ("AvgArray"=w284:dbl[])  [unwired: 7 in, 1 out]
                    n224 = Divide(x="Smoothing Range", y=w274) -> (x/y=w269:dbl)
                    "Smoothed Bins" <- w269
                    n225 = call "Smooth Arrray.vi"("smooth size"=w269, "Raw Array"=w303) -> ("Smoothed Array"=→"On-Line  Smoothed":dbl[])  [unwired: 9 in]
                    n226 = call "Smooth Arrray.vi"("smooth size"=w269, "Raw Array"=w284) -> ("Smoothed Array"=→"On-Line Smoothed 2":dbl[])  [unwired: 9 in]
                    n227 = disable-structure shown="Disabled" {
                      frame Disabled {
                        n228 = script code="format long;\ncounts=sum(Online);\nif counts >=0.5e6\ntime=time;\nelse\ntime=time\nend"() -> ()  [unwired: 3 in, 2 out]
                      }
                      frame Enabled {
                      }
                    }
                  }
                  frame #4 {
                    # "CODE REMOVED!!"
                    # "Toggling the Agiltron switch to the offline DBR seed laser"
                  }
                  frame #5 {
                    # "Save the recently collected online data if 'Save Data?' is true"
                    n229 = case shown="True" "Save Data?" {
                      frame False {
                        # "'Save Data?' is false, do nothing"
                      }
                      frame True {
                        # "'Save Data?' is true, save onfline data to the Data Disk"
                        # "Write only one copy of data at this time"
                        # "Retrieve Julian Date"
                        n230 = local read "Readings"() -> (w328:T5)
                        n231 = local read "Time Resolution Per Bin(ns)"() -> (w326:u32)
                        n232 = local read "Number of Accumulates"() -> (w324:u32)
                        n233 = local read "Number of Bins"() -> (w325:u32)
                        n234 = local write "DataOpen"(TRUE ("DataOpen")) -> ()
                        n235 = local read "Lambda On Read (nm)"() -> (w350:dbl)
                        n236 = local read "On-Line Bin Readings 2"() -> (w348:dbl[])
                        n237 = local read "On-Line Bin Readings"() -> (w352:dbl[])
                        n238 = local read "Average Diode Power"() -> (w349:dbl)
                        n239 = Unbundle By Name(w328) -> ("OnLineLD"=w327:dbl)
                        n240 = To Double Precision Float(number=w326) -> (double precision float=w323:dbl)
                        n241 = To Double Precision Float(number=w325) -> (double precision float=w322:dbl)
                        n242 = To Double Precision Float(number=w324) -> (double precision float=w321:dbl)
                        n243 = call "Julian_Date_2.vi"() -> ("Julian Date"=w351:dbl)  [unwired: 11 in]
                        n244 = Build Array (concatenate)(w351, w350, w327, w349, w323, w322, w321, w352) -> (w343:dbl[])
                        n245 = Build Array (concatenate)(w351, w350, w327, w349, w323, w322, w321, w348) -> (w333:dbl[])
                        n246 = local read "NF_On_Ref"() -> (w331:refnum<file>)
                        n247 = local read "FF_On_Ref"() -> (w347:refnum<file>)
                        n248 = local read "NF_On_Ptr"() -> (w332:i64)
                        n249 = local read "FF_On_Ptr"() -> (w346:i64)
                        n250 = Set File Position(offset (in bytes) (0)=w346, refnum=w347) -> (refnum out=w344:refnum<file>, error out=w341:errorcluster)  [unwired: 2 in]
                        n251 = Set File Position(offset (in bytes) (0)=w332, refnum=w331) -> (refnum out=w337:refnum<file>, error out=w335:errorcluster)  [unwired: 2 in]
                        n252 = Write to Binary File(file (use dialog)=w337, data=w333, error in=w335, 5:FALSE ("prepend array or string size? (T)")) -> (refnum out=w336:refnum<file>, error out=w334:errorcluster)  [unwired: 2 in, 1 out]
                        n253 = Write to Binary File(file (use dialog)=w344, data=w343, error in=w341, 5:FALSE ("prepend array or string size? (T)")) -> (refnum out=w342:refnum<file>, error out=w340:errorcluster)  [unwired: 2 in, 1 out]
                        n254 = Get File Position(4:w334, 7:w336) -> (2:w330:i64)  [unwired: 2 out]
                        n255 = Get File Position(4:w340, 7:w342) -> (2:w339:i64)  [unwired: 2 out]
                        n256 = local write "NF_On_Ptr"(w330) -> ()
                        n257 = local write "FF_On_Ptr"(w339) -> ()
                      }
                    }
                  }
                }
              }
              frame #3 {
                # "Frame 3: Read offline data, calculate aerosol data, and plot offline and normalized relative backscatter\nFrame 4: Swich to online DBR\nFrame 5: Save the offline data and related information"
                # "Frame 0: Read the offline wavelength and lock if necessary, though code is not finished to do so\nFrame 1: Read the output power from the Newport power meter\nFrame 2: Wait 'Scalar Wait Time' for buffers to clear of online contiminated data"
                # "offline"
                n258 = stacked-sequence {
                  frame #0 {
                    # "Every 60 data collection cycles, read the offline DBR wavelength, and if outside of wavelength tolerance, adjust DBR current until within tolerance"
                    n259 = local read "L_Count"() -> (w354:i32)
                    n260 = Quotient & Remainder(x=w354, y=60.0) -> (x-y*floor(x/y)=w355:dbl)  [unwired: 1 out]
                    n261 = Equal To 0?(x=w355) -> (x = 0?=w353:bool)
                    n262 = case shown="True" w353 {
                      frame False {
                      }
                      frame True {
                        n263 = while {
                          i -> [w360]
                          stop <- w358 stop-if-true
                          # "Frame 5 Increment ofline DBR current if below tolerance\nFrame 6: update ILX settings to front pannel"
                          # "Frame 3: Calculating the wavelength difference\nFrame 4:Decrement offline DBR current if above tolerance"
                          # "Frame 0: Read the offline laser wavelength (settle if t=0)"
                          n264 = stacked-sequence {
                            tunnel: w360 -> [w362 _ _ _ _]
                            tunnel: [_ _ w372 _ _] -> w359
                            frame #0 {
                              n265 = Equal To 0?(x=w362) -> (x = 0?=w361:bool)
                              n266 = case shown="True" w361 {
                                frame False {
                                }
                                frame True {
                                w363 = TRUE ("Boolean")
                                # "SWITCH to NON-ABSORBING and wait to settle"
                                n267 = Build Array(w363) -> (w368:bool[])
                                n268 = local write "WM Switch"(w363) -> ()
                                n269 = call-poly <vilib>:"DAQmx Write.vi"("task/channels in"=refnum<k21> "BristolWM", "data"=w368) -> ()  [unwired: 11 in, 3 out]
                                n270 = call "TL_Driver.vi"("Device In"=refnum<visa-resource-name> "ThorLabs", "Commands"=T9."Read_Status") -> ("Readings"=w366:T5)  [unwired: 10 in, 3 out]
                                n271 = local write "Readings"(w366) -> ()
                                n272 = Wait (ms)(milliseconds to wait=u32 3200) -> ()  [unwired: 1 out]
                                }
                              }
                            }
                            frame #1 {
                              # "Read Bristol WM"
                              n273 = local read "Bristol Out"() -> (w370:i32)
                              n274 = dll-call lib="C:/H2O_DIAL/LabVIEW-2012/Bristol WM V2_31b/CLDevIface.dll" fn="CLGetLambdaReading"("devHandle"=w370) -> ("return type"=→"Lambda Off Read (nm)":dbl)  [unwired: 4 in, 2 out]
                            }
                            frame #2 {
                              # "Once locked, stop looping and illuminate 'Wavelength Lock Offline'"
                              # "While loop continues locking process until the wavelength is within tolerance"
                              # "Calculating the difference between the actual and desired \noffline wavelength"
                              n275 = local read "Lambda Off Read (nm)"() -> (w380:dbl)
                              n276 = Subtract(x=w380, y="Lambda Off Set (nm)") -> (x-y=w373:dbl)
                              "WL Difference off" <- w373
                              n277 = local read "NONAB_DIF"() -> (w377:dbl)
                              n278 = Multiply(x=-1.0, y=w377) -> (x*y=w378:dbl)
                              n279 = Greater?(x=w373, y=w378) -> (0:w374:bool)
                              n280 = Less?(x=w373, y=w377) -> (x < y?=w375:bool)
                              n281 = And(x=w374, y=w375) -> (x .and. y?=w372:bool)
                              "Wavelength Lock Offline" <- w372
                              n282 = case shown="True" w372 {
                                frame False {
                                }
                                frame True {
                                w381 = FALSE ("Boolean")
                                # "SWITCH back to ABSORBING and wait to settle"
                                n283 = Build Array(w381) -> (w383:bool[])
                                n284 = local write "WM Switch"(w381) -> ()
                                n285 = call-poly <vilib>:"DAQmx Write.vi"("task/channels in"=refnum<k21> "BristolWM", "data"=w383) -> ()  [unwired: 11 in, 3 out]
                                n286 = Wait (ms)(milliseconds to wait=u32 3200) -> ()  [unwired: 1 out]
                                }
                              }
                            }
                            frame #3 {
                              # "Would adjust the offline wavelength if code was finished"
                              n287 = local read "WL Difference off"() -> (w387:dbl)
                              n288 = Greater Or Equal?(x=w387, y="NONAB_DIF") -> (x >= y?=w385:bool)
                              n289 = case shown="True" w385 {
                                frame False {
                                # "WL difference is not out of range, do nothing"
                                }
                                frame True {
                                # "Generating a command string\nto decrement the current"
                                # "WL difference is greater than 0.0002 nm,\ndecrement the DBR current by 0.01 mA"
                                # "WL difference is out of range, this is where you would decrement\nthe laser current"
                                n290 = local read "Settings"() -> (w392:T6)
                                n291 = Unbundle By Name(w392) -> ("OffLineLD"=w393:dbl)
                                n292 = Subtract(x=w393, y=3e-06) -> (x-y=w394:dbl)
                                n293 = Bundle By Name(cluster=w392, "OffLineLD"=w394, "Module"=T11."Off Line LD") -> (w391:T6)
                                n294 = call "TL_Driver.vi"("Device In"=refnum<visa-resource-name> "ThorLabs", "Commands"=T9."SET", "Settings"=w391) -> ("Readings"=w388:T5)  [unwired: 9 in, 3 out]
                                n295 = local write "Settings"(w391) -> ()
                                n296 = local write "Readings"(w388) -> ()
                                }
                              }
                            }
                            frame #4 {
                              # "This is where you would increment the offline current if below tolerance"
                              n297 = local read "NONAB_DIF"() -> (w398:dbl)
                              n298 = local read "WL Difference off"() -> (w401:dbl)
                              n299 = Multiply(x=-1.0, y=w398) -> (x*y=w397:dbl)
                              n300 = Less Or Equal?(x=w401, y=w397) -> (x <= y?=w400:bool)
                              n301 = case shown="True" w400 {
                                frame False {
                                # "WL difference is not outisde tolerance, do nothing"
                                }
                                frame True {
                                # "Generating a command string\nto decrement the current"
                                # "WL difference is less than 0.0002 nm,\nincrement the DBR current by 0.01 mA"
                                # "Incrementing the current if below tolerance"
                                n302 = local read "Settings"() -> (w405:T6)
                                n303 = Unbundle By Name(w405) -> ("OffLineLD"=w407:dbl)
                                n304 = Add(x=w407, y=3e-06) -> (x+y=w408:dbl)
                                n305 = Bundle By Name(cluster=w405, "OffLineLD"=w408, "Module"=T11."Off Line LD") -> (w406:T6)
                                n306 = call "TL_Driver.vi"("Device In"=refnum<visa-resource-name> "ThorLabs", "Commands"=T9."SET", "Settings"=w406) -> ("Readings"=w402:T5)  [unwired: 9 in, 3 out]
                                n307 = local write "Settings"(w406) -> ()
                                n308 = local write "Readings"(w402) -> ()
                                }
                              }
                            }
                          }
                          n309 = Or(x=w359, y="Cancel Offline") -> (x .or. y?=w358:bool)
                        }
                      }
                    }
                  }
                  frame #1 {
                    # "CODE REMOVED!!!"
                    # "Reading the output power of the laser transmitter from the Ophir power meter, once read, convert to corresponding pulse energy and plot"
                  }
                  frame #2 {
                    # "CODE REMOVED!!!"
                    # "Wait 'Scalar Wait Time' for buffers to clear of online contiminated offline data"
                  }
                  frame #3 {
                    w442 = 1 ("dimension size")
                    w446 = 1
                    # "Plotting the normalized relative \nbackscatter"
                    # "Calculating the normalized relative backscatter"
                    # "Calculating/Plotting smoothed data,\ncross sections etc."
                    # "Pick off data with\nout header"
                    # "Calculate mean bin by bin mean"
                    # "Reading in 'Integration Period (Seconds)' of data"
                    # "Read the offline data from the scalar card, perform smoothing, calculate normalized relative backscatter, and plot"
                    # "File path in MATLAB script is of old dial is:\nF:\\Micropulse DIAL\\Micropulse DIAL Matlab\\\nFinal Overlap Function.mat')];"
                    # "Collects Data From Card,\nSends It To The Chart,\nAnd Saves A Copy As A\nFile If Option Selected On\nFront Panel"
                    n310 = for {
                      N: "Data Reads (number of loops)" -> [_]
                      tunnel: [w480] -> w477 mode=indexing
                      tunnel: [w479] -> w459 mode=indexing
                      # "Read in latest scalar card data from \n'Scalar Data' global variable that \nscaler.vi is writing to, then wait 1 sec\nfor next batch of data"
                      n311 = disable-structure shown="Disabled" {
                        frame Disabled {
                          n312 = global read "Scalar_Data.vi" "Scalar Data  2"() -> ()  [unwired: 1 out]
                          n313 = global read "Scalar_Data.vi" "Scalar Data  4"() -> ()  [unwired: 1 out]
                        }
                        frame Enabled {
                        }
                      }
                      n314 = global read "AMCS_Data.vi" "AMCS_Data"() -> (w483:u16[][])
                      n315 = Index Array(array=w483, index (row) #1=1 ("index (row)"), index (row) #2=3 ("index (row)")) -> (element #1=w480:u16[], element #2=w479:u16[])  [unwired: 2 in]
                    }
                    n316 = local read "Total DIAL Integration Time (Minutes)"() -> (w468:i32)
                    n317 = Divide(x=w468, y="Data Reads (number of loops)") -> (x/y=w466:dbl)
                    n318 = local read "Total Aerosol Integration Time (Minutes)"() -> (w470:dbl)
                    n319 = local read "background length"() -> (w414:i32)
                    n320 = Multiply(x=w466, y=60.0) -> (x*y=w452:dbl)
                    n321 = local read "background start"() -> (w415:u32)
                    n322 = Transpose 2D Array(2D array=w477) -> (transposed array=w476:u16[][])
                    n323 = Transpose 2D Array(2D array=w459) -> (transposed array=w458:u16[][])
                    n324 = Divide(x=w470, y="Data Reads (number of loops)") -> (x/y=w471:dbl)
                    n325 = for {
                      tunnel: w476 -> [w487] mode=indexing
                      tunnel: [w486] -> w478 mode=indexing
                      tunnel: w458 -> [w485] mode=indexing
                      tunnel: [w484] -> _ mode=indexing
                      tunnel: [w484] -> w455 mode=indexing
                      n326 = call-poly <vilib>:"Mean.vi"("X"=w487) -> ("mean"=w486:dbl)  [unwired: 1 out]
                      n327 = call-poly <vilib>:"Mean.vi"("X"=w485) -> ("mean"=w484:dbl)  [unwired: 1 out]
                    }
                    n328 = local read "bins"() -> (w443:u32)
                    n329 = Multiply(x=w471, y=60.0) -> (x*y=w433:dbl)
                    n330 = Array Subset(array=w455, index=w442, length=w443) -> (w456:dbl[])
                    "Off-Line Bin Readings 2" <- w456
                    n331 = Array Subset(array=w478, index=w442, length=w443) -> (w454:dbl[])
                    "Off-Line  Bin Readings" <- w454
                    n332 = Array Subset(array=w456, index=w415, length=w414) -> (w457:dbl[])
                    n333 = Array Subset(array=w454, index=w415, length=w414) -> (w475:dbl[])
                    n334 = local read "Smoothed Bins"() -> (w411:dbl)
                    n335 = call-poly <vilib>:"Mean.vi"("X"=w457) -> ("mean"=w421:dbl)  [unwired: 1 out]
                    n336 = call-poly <vilib>:"Mean.vi"("X"=w475) -> ("mean"=w422:dbl)  [unwired: 1 out]
                    n337 = local read "Index"() -> (w432:i32)
                    n338 = Subtract(x=w456, y=w421) -> (x-y=w434:dbl[])
                    n339 = Subtract(x=w454, y=w422) -> (x-y=w450:dbl[])
                    n340 = call "Ring Buffer Offline Far.vi"("Index"=w432, "Profiles to Average"=w452, "Input Array"=w450) -> ("AvgArray"=w473:dbl[], "RingBufferOut"=→"RingBuffer offline far":dbl[][])  [unwired: 7 in]
                    n341 = call "Ring Buffer Aerosol Far.vi"("Index"=w432, "Profiles to Average"=w433, "Input Array"=w450) -> ("AvgArray"=w469:dbl[], "RingBufferOut"=→"RingBuffer aerosol far":dbl[][])  [unwired: 7 in]
                    n342 = call "Ring Buffer Offline Near.vi"("Index"=w432, "Profiles to Average"=w452, "Input Array"=w434) -> ("AvgArray"=w453:dbl[], "RingBufferOut"=→"RingBuffer offline near":dbl[][])  [unwired: 7 in]
                    n343 = call "Ring Buffer Aerosol Near.vi"("Index"=w432, "Profiles to Average"=w433, "Input Array"=w434) -> ("AvgArray"=w430:dbl[], "RingBufferOut"=→"RingBuffer aerosol near":dbl[][])  [unwired: 7 in]
                    n344 = Reshape Array(w450, w442, w443) -> (→"raw counts":dbl[][])
                    n345 = Reshape Array(w434, w442, w443) -> (→"raw counts near":dbl[][])
                    n346 = call "Smooth Arrray.vi"("smooth size"=w411, "Raw Array"=w473) -> ("Smoothed Array"=→"Off-Line Smoothed":dbl[])  [unwired: 9 in]
                    n347 = call "Smooth Arrray.vi"("smooth size"=w411, "Raw Array"=w469) -> ("Smoothed Array"=w441:dbl[])  [unwired: 9 in]
                    "Aerosol Smoothed" <- w441
                    n348 = call "Smooth Arrray.vi"("smooth size"=w411, "Raw Array"=w453) -> ("Smoothed Array"=→"Off-Line Smoothed 2":dbl[])  [unwired: 9 in]
                    n349 = call "Smooth Arrray.vi"("smooth size"=w411, "Raw Array"=w430) -> ("Smoothed Array"=w413:dbl[])  [unwired: 9 in]
                    "Aerosol Smoothed 2" <- w413
                    n350 = local read "Number of Accumulates"() -> (w417:u32)
                    n351 = local read "Temperature (C)"() -> (w465:dbl)
                    n352 = local read "Pressure (mb)"() -> (w464:dbl)
                    n353 = script code="%accum_num=10000;     % scaler card setting number of accumulations\nt_bin = 500e-9                 % scaler card setting time per bin\n%t_d = 37.3e-9;                % APD dead time from spec sheet\n\n% conversion from accumulated counts to count rate  (c/s)\nc_convert = 1./t_bin./accum_num;\nCR_far = p_raw_far.*c_convert;\nCR_near = p_raw_near.*c_convert;\nCR_total_far = (p_raw_far+b_far).*c_convert;\nCR_total_near = (p_raw_near+b_near).*c_convert;\nb_CR_far =b_far.*c_convert;\nb_CR_near =b_near.*c_convert;\n\n% create a range array\nsize_p =  size(p_raw_far,2);\nr = (75:75:size_p*75)./1e3; \n    \n%APD correction factor\n D_far = 1./(1-(t_d*CR_total_far));\n D_near = 1./(1-(t_d*CR_total_near));\n\n %Calculating normalize relative backscatter profile\n nrb_far = CR_far.*D_far.*r.^2./E.*1e-6;\n nrb_near = CR_near.*D_near.*r.^2./E.*1e-6;"("E"=6.0 ("Real"), "temp"=w465, "press"=w464, "p_raw_far"=w441, "b_far"=w422, "b_near"=w421, "p_raw_near"=w413, "accum_num"=w417, "t_d"="dead time") -> ("nrb_far"=w436:cdb[], "D_far"=w427:dbl[], "nrb_near"=w435:cdb[], "D_near"=w426:dbl[], "b_CR_far"=w419:dbl, "b_CR_near"=w418:dbl)  [unwired: 1 in, 1 out]
                    n354 = local read "bins"() -> (w445:u32)
                    n355 = local read "Altitude Array (km)"() -> (w438:dbl[])
                    n356 = Bundle(w419, w418) -> (→"?":cluster{dbl, dbl})  [unwired: 1 in]
                    n357 = Build Array(w436, w435) -> (w440:cdb[][])
                    n358 = Build Array(w427, w426) -> (w425:dbl[][])
                    n359 = Reshape Array(w435, w446, w445) -> (→"NRB 2":cdb[][])
                    n360 = Reshape Array(w436, w446, w445) -> (→"NRB":cdb[][])
                    n361 = Build Array(w438, w438) -> (w437:dbl[][])
                    n362 = call "Convert to Dynamic Data7"("2D Array"=w425) -> ("Dynamic Data Type"=w424:dynamicdata)  [unwired: 3 in]
                    n363 = call "Convert to Dynamic Data3"("2D Array"=w440) -> ("Dynamic Data Type"=w439:dynamicdata)  [unwired: 3 in]
                    n364 = call "Convert to Dynamic Data4"("2D Array"=w437) -> ("Dynamic Data Type"=w428:dynamicdata)  [unwired: 3 in]
                    n365 = call "Build XY Graph2"("Y Input"=w428, "X Input"=w439) -> ("XY Graph"=→"NRB plot":cluster{"Y":dbl[], "Y":dbl[]}[])  [unwired: 3 in, 6 out]
                    n366 = call "Build XY Graph4"("Y Input"=w428, "X Input"=w424) -> ("XY Graph"=→"Correction":cluster{"Y":dbl[], "Y":dbl[]}[])  [unwired: 3 in, 6 out]
                  }
                  frame #4 {
                    # "CODE REMOVED!!!"
                    # "Toggle Agiltron switch to online DBR"
                  }
                  frame #5 {
                    # "If 'Save Data?' is true, save all relavant offline info"
                    n367 = local read "Save Data?"() -> (w488:bool)
                    n368 = case shown="True" w488 {
                      frame False {
                        # "'Save Data?' is false, do nothing"
                      }
                      frame True {
                        # "Write only one data file at this time"
                        # "Retrive Julian Date"
                        # "'Save Data?' is true, save offline data to the Data Disk"
                        n369 = local read "Readings"() -> (w490:T5)
                        n370 = local read "Off-Line Bin Readings 2"() -> (w509:dbl[])
                        n371 = local read "Lambda Off Read (nm)"() -> (w511:dbl)
                        n372 = local read "Off-Line  Bin Readings"() -> (w516:dbl[])
                        n373 = local read "Relative Humdity (%)"() -> (w515:dbl)
                        n374 = local read "Average Diode Power"() -> (w512:dbl)
                        n375 = local read "Temperature (C)"() -> (w513:dbl)
                        n376 = Unbundle By Name(w490) -> ("OffLineLD"=w489:dbl)
                        n377 = local read "Pressure (mb)"() -> (w514:dbl)
                        n378 = call "Julian_Date_2.vi"() -> ("Julian Date"=w510:dbl)  [unwired: 11 in]
                        n379 = Build Array (concatenate)(w510, w511, w489, w512, w513, w514, w515, w516) -> (w495:dbl[])
                        n380 = Build Array (concatenate)(w510, w511, w489, w512, w513, w514, w515, w509) -> (w492:dbl[])
                        n381 = local read "FF_Off_Ref"() -> (w497:refnum<file>)
                        n382 = local read "NF_Off_Ref"() -> (w494:refnum<file>)
                        n383 = local read "FF_Off_Ptr"() -> (w496:i64)
                        n384 = local read "NF_Off_Ptr"() -> (w493:i64)
                        n385 = Set File Position(offset (in bytes) (0)=w496, refnum=w497) -> (refnum out=w508:refnum<file>, error out=w506:errorcluster)  [unwired: 2 in]
                        n386 = Set File Position(offset (in bytes) (0)=w493, refnum=w494) -> (refnum out=w504:refnum<file>, error out=w502:errorcluster)  [unwired: 2 in]
                        n387 = Write to Binary File(file (use dialog)=w508, data=w495, error in=w506, 5:FALSE ("prepend array or string size? (T)")) -> (refnum out=w507:refnum<file>, error out=w505:errorcluster)  [unwired: 2 in, 1 out]
                        n388 = Write to Binary File(file (use dialog)=w504, data=w492, error in=w502, 5:FALSE ("prepend array or string size? (T)")) -> (refnum out=w503:refnum<file>, error out=w501:errorcluster)  [unwired: 2 in, 1 out]
                        n389 = Get File Position(4:w505, 7:w507) -> (2:w498:i64)  [unwired: 2 out]
                        n390 = Get File Position(4:w501, 7:w503) -> (2:w491:i64)  [unwired: 2 out]
                        n391 = local write "FF_Off_Ptr"(w498) -> ()
                        n392 = local write "NF_Off_Ptr"(w491) -> ()
                      }
                    }
                  }
                }
              }
              frame #4 {
                n393 = First Call?() -> (First Call?: T/F=w519:bool)
                n394 = Or(x="calculate absorption cross sections", y=w519) -> (x .or. y?=w517:bool)
                n395 = case shown="True" w517 {
                  frame False {
                  }
                  frame True {
                    # "calculate absorption cross sections from HITRAN data base"
                    n396 = local read "Off-Line Smoothed"() -> (w520:dbl[])
                    n397 = local read "Lambda On Read (nm)"() -> (w523:dbl)
                    n398 = local read "Lambda Off Set (nm)"() -> (w526:dbl)
                    n399 = local read "Temperature (C)"() -> (w524:dbl)
                    n400 = local read "Pressure (mb)"() -> (w525:dbl)
                    n401 = script code="hitran = dlmread('C:\\H2O_DIAL\\LabVIEW-2012\\Micropulse DIAL Matlab\\815nm_841nm_HITRAN_2008.csv', ',',[1 1 1676 8]);\n%hitran = dlmread('C:\\H2O_DIAL\\LabVIEW-2012\\Micropulse DIAL Matlab\\824nm_841nm_H2O_Spectral_Calc.csv', ',',[1 1 1209 7]);\n\n\n\n%Range vector in meters\nrange = ([75:75:size(Online,2)*75]);\n\nif lambda< 828\nlambda=828.195;\nelse\nlambda=lambda;\nend;\n\n%%\n\n%Voigt profile calculation\nWNmin = 1/(828+4)*1e7;  % 832.0 nm converted to wavenumber\nWNmax = 1/(828-4)*1e7;  % 824.0 nm converted to wavenumber\n\n%Find lines from WNmin to WNmax to calculate voigt profile\nline_indices = hitran(1:size(hitran,1),1)>WNmin & hitran(1:size(hitran,1),1)<WNmax;\n\nline = double(hitran(line_indices, 1:size(hitran,2)));\n\n%Calculate temperature and pressure profile\nT0 = 273+25; % surface temperature\nT0 = 273+T0_C;\nT = T0-0.0065.*range; % set to match the sounding\n\n% pressure in atmospheres\nP0  = 0.83; % surface pressure\nP0  = P0_mb/1000*0.986; %pressure in mb converted to atm\nP = P0.*(T0./T).^-5.5;   % set this value to match sounding\n\nT00 = 296;              % HITRAN reference temperature [K]\nP00 = 1;                % HITRAN reference pressure [atm]\nnu0_0 = line(:,1);      % absorption line center wavenumber from HITRAN [cm^-1]\nS0 = line(:,2);         % initial linestrength from HITRAN [cm^-1/(mol*cm^-2)]   \ngammal0 = line(:,4);    % air-broadened halfwidth at T_ref and P_ref from HITRAN [cm^-1/atm]\ngamma_s = line(:,5);    % self-broadened halfwidth at T_ref and P_ref from HITRAN [cm^-1/atm]\nE = line(:,6);          % ground state transition energy from HITRAN [cm^-1]  \nalpha = line(:,7);      % linewidth temperature dependence factor from HITRAN\ndelta = line(:,8);      % pressure shift from HiTRAN [cm^-1 atm^-1]\n\nnu_on = 1/(lambda)*1e7;\nnu_off = 1/(lambda_off)*1e7;\n\nfor i = 1:size(Online,2); % calculate the absorption cross section at each range\n  \n    nu0 = nu0_0+delta.*(P(i)./P00); % unclear if it should be Pi/P00  \n    gammal = gammal0.*(P(i)./P00).*((T00./T(i)).^alpha);    %Calculate Lorentz lineweidth at P(i) and T(i)\n\n    const.m = 18.015E-3./6.022E23; % mass of a single water molecule\n    const.k_B = 1.3806488e-23; % (J/K)\n    const.c = 299792458; % (m/s) (exact)\n \n    gammad = (nu0).*((2.0.*const.k_B.*T(i).*log(2.0))./(const.m.*const.c^2)).^(0.5);  %Calculate HWHM Doppler linewidth at T(i)\n     \n    % term 1 in the Voigt profile\n    y = (gammal./gammad).*((log(2.0)).^(0.5));\n    \n    % term 2 in the Voigt profile\n    x_on = ((nu_on-nu0)./gammad).*(log(2.0)).^(0.5);\n    x_off = ((nu_off-nu0)./gammad).*(log(2.0)).^(0.5);\n    \n    %setting up Voigt convolution\n    t = (-(size(line,1))/2:1:size(line,1)/2-1); %set up the integration spectral step size\n    t = repmat(t',1,length(x_on))';\n    x_on = repmat(x_on,1,length(t));\n    x_off = repmat(x_off,1,length(t));\n    y = repmat(y,1,length(t));\n    f_on = (exp(-t.^2.0))./(y.^2.0+(x_on-t).^2.0);  % combined Voigt term 1 and 2\n    f_off = (exp(-t.^2.0))./(y.^2.0+(x_off-t).^2.0);\n    %Voigt integration over all of the lines at the on and offline locations\n    z_on = trapz(t(1,:),f_on,2);\n    z_off =  trapz(t(1,:),f_off,2);\n    integral_on = z_on;\n    integral_off = z_off;\n    %Calculate linestrength at temperature T\n    S = S0.*((T00./T(i)).^(1.5)).*exp(1.439.*E.*((1./T00)-(1./T(i))));\n \n    %Calculate the Voigt profile\n    K_on = (y(:,1)./pi).*integral_on;\n    K_off = (y(:,1)./pi).*integral_off;\n    \n    %Calculate the Voigt profile absorption cross section [cm^2]\n    sigmav_on = S.*(1./gammad).*(((log(2.0))./pi).^(0.5)).*K_on; %.*far_wing_on;\n    sigmav_off = S.*(1./gammad).*(((log(2.0))./pi).^(0.5)).*K_off; %.*far_wing_off;\n    \n    %Sum contributions from all of the surrounding lines\n    sigma_on_total(i) = sum(sigmav_on);\n    sigma_off_total(i) = sum(sigmav_off);\n    \nend;"("lambda"=w523, "lambda_off"=w526, "P0_mb"=w525, "T0_C"=w524, "Online"=w520) -> ("sigma_on_total"=→"sigma_on_total":dbl[], "sigma_off_total"=→"sigma_off_total":dbl[])  [unwired: 1 in, 1 out]
                  }
                }
              }
              frame #5 {
                w537 = 1
                # "normalization factor\nfrom 300 to 450m"
                # "OPTICAL DEPTH PLOT"
                # "new rainbow color bar display"
                # "Data Processing Far Channel"
                # "new rainbow color bar display"
                # "Calculating the range resolved water vapor number density and plotting"
                n402 = local read "sigma_off_total"() -> (w560:dbl[])
                n403 = local read "sigma_on_total"() -> (w557:dbl[])
                n404 = local read "On-Line  Smoothed"() -> (w535:dbl[])
                n405 = local read "Off-Line Smoothed"() -> (w534:dbl[])
                n406 = local read "Off-Line Smoothed 2"() -> (w558:dbl[])
                n407 = local read "On-Line Smoothed 2"() -> (w559:dbl[])
                n408 = script code="%Time averaging in seconds.  180 Seconds =3 minutes\ntemporal_average = 180;\n\n%Spatial averaging in bins.  2 bins = 150 meters\nspatial_average = 2;\n\n%Creating r and r+deltar vectors..this can also be acsomplished using the\n%diff command\np_oni = Online(:,1:size(Online,2)-1);\n\np_onii = Online(:,2:size(Online,2));\n\np_offi = Offline(:,1:size(Offline,2)-1);\n\np_offii = Offline(:,2:size(Offline,2));\n\nInside = (p_oni.*p_offii)./(p_onii.*p_offi);\n\ndel_cross = 1./(2.*(sigma_on_total(1:size(Online,2)-1)-sigma_off_total(1:size(Offline,2)-1)).*75*100);\n\ndel_cross(isinf(del_cross)) = 0;\n\n%Calculating Number density\nN = del_cross.*log(Inside);\n\n%Spatial smoothing of the profiles\nfilter1 = ones(1,2)./2;\n\nN_1 = N;\n\nN_1_avg = filter2(filter1,N_1);\n\nfilter1 = ones(1,10)./10;\n\nN_2 = N;\n\nN_2_avg = filter2(filter1,N_2);\n\nN_new = zeros(size(N,1),size(N,2));\n \n%Using different averaging windows for different altitudes \nN_avg=[N_1_avg(:,1:40)';N_2_avg(:,41:size(N,2))']';\n\n\nw = N_avg.*1e6.*18.015./6.022e23"("Online"=w559, "Offline"=w558, "sigma_on_total"=w557, "sigma_off_total"=w560) -> ("N_avg"=w561:cdb[], "w"=w570:cdb[])  [unwired: 1 in, 1 out]
                n409 = script code="%Time averaging in seconds.  180 Seconds = 3 minutes\ntemporal_average = 180;\n\n%Spatial averaging in bins.  2 bins = 150 meters\nspatial_average = 2;\n\n%Creating r and r+deltar vectors..this can also be acsomplished using the\n%diff command\np_oni = Online(:,1:size(Online,2)-1);\n\np_onii = Online(:,2:size(Online,2));\n\np_offi = Offline(:,1:size(Offline,2)-1);\n\np_offii = Offline(:,2:size(Offline,2));\n\nInside = (p_oni.*p_offii)./(p_onii.*p_offi);\n\ndel_cross = 1./(2.*(sigma_on_total(1:size(Online,2)-1)-sigma_off_total(1:size(Offline,2)-1)).*75*100);\n\ndel_cross(isinf(del_cross)) = 0;\n\n%Calculating Number density\nN = del_cross.*log(Inside);\n\n%Spatial smoothing of the profiles\nfilter1 = ones(1,2)./2;\n\nN_1 = N;\n\nN_1_avg = filter2(filter1,N_1);\n\nfilter1 = ones(1,10)./10;\n\nN_2 = N;\n\nN_2_avg = filter2(filter1,N_2);\n\nN_new = zeros(size(N,1),size(N,2));\n \n%Using different averaging windows for different altitudes \nN_avg=[N_1_avg(:,1:40)';N_2_avg(:,41:size(N,2))']';\n\n \nw = N_avg.*1e6.*18.015./6.022e23"("Online"=w535, "Offline"=w534, "sigma_on_total"=w557, "sigma_off_total"=w560) -> ("N_avg"=w566:cdb[], "w"=w567:cdb[])  [unwired: 1 in, 1 out]
                n410 = local read "Time Resolution Per Bin(ns)"() -> (w536:u32)
                n411 = local read "bins"() -> (w562:u32)
                n412 = local read "Altitude Array (km)"() -> (w532:dbl[])
                n413 = Build Array(w567, w570) -> (w573:cdb[][])
                n414 = To Double Precision Float(number=w536) -> (double precision float=w555:dbl)
                n415 = Reshape Array(w566, w537, w562) -> (w577:cdb[][])
                n416 = Reshape Array(w561, w537, w562) -> (w564:cdb[][])
                n417 = Multiply(x=0.15, y=w555) -> (x*y=w553:dbl)
                n418 = Build Array(w566, w561) -> (w571:cdb[][])
                n419 = Divide(x=300.0, y=w553) -> (x/y=w550:dbl)
                n420 = Divide(x=450.0, y=w553) -> (x/y=w549:dbl)
                n421 = Build Array(w532, w532) -> (w556:dbl[][])
                n422 = call "Convert to Dynamic Data5"("2D Array"=w573) -> ("Dynamic Data Type"=w572:dynamicdata)  [unwired: 3 in]
                n423 = call "Convert to Dynamic Data2"("2D Array"=w571) -> ("Dynamic Data Type"=w568:dynamicdata)  [unwired: 3 in]
                n424 = Divide(x=w577, y=1e+17) -> (x/y=→"Water Vapor Number Density":cdb[][])
                n425 = Divide(x=w564, y=1e+17) -> (x/y=→"Water Vapor Number Density 2":cdb[][])
                n426 = call "Convert to Dynamic Data6"("Array"=w532) -> ("Dynamic Data Type"=w533:dynamicdata)  [unwired: 3 in]
                n427 = To Long Integer(number=w550) -> (32bit integer=w548:i32)
                n428 = To Long Integer(number=w549) -> (32bit integer=w547:i32)
                n429 = call "Convert to Dynamic Data"("2D Array"=w556) -> ("Dynamic Data Type"=w569:dynamicdata)  [unwired: 3 in]
                n430 = call "Convert to Dynamic Data8"("2D Array"=w556) -> ("Dynamic Data Type"=w574:dynamicdata)  [unwired: 3 in]
                n431 = Decrement(x=w548) -> (x-1=w545:i32)
                n432 = Decrement(x=w547) -> (x-1=w546:i32)
                n433 = call "Build XY Graph"("Y Input"=w569, "X Input"=w568) -> ("XY Graph"=→"Water Vapor Number Density  2":cluster{"Y":dbl[], "Y":dbl[]}[])  [unwired: 3 in, 6 out]
                n434 = call "Build XY Graph3"("Y Input"=w574, "X Input"=w572) -> ("XY Graph"=→"Absolute Humidity":cluster{"Y":dbl[], "Y":dbl[]}[])  [unwired: 3 in, 6 out]
                n435 = Array Subset(array=w535, index=w545, length=w546) -> (w544:dbl[])
                n436 = Array Subset(array=w534, index=w545, length=w546) -> (w543:dbl[])
                n437 = call-poly <vilib>:"Mean.vi"("X"=w544) -> ("mean"=w542:dbl)  [unwired: 1 out]
                n438 = call-poly <vilib>:"Mean.vi"("X"=w543) -> ("mean"=w541:dbl)  [unwired: 1 out]
                n439 = Divide(x=w542, y=w541) -> (x/y=w540:dbl)
                n440 = Multiply(x=w534, y=w540) -> (x*y=w539:dbl[])
                n441 = Divide(x=w535, y=w539) -> (x/y=w538:dbl[])
                n442 = Natural Logarithm(1:w538) -> (0:w529:dbl[])
                n443 = Multiply(x=-1.0, y=w529) -> (x*y=w528:dbl[])
                n444 = call "Convert to Dynamic Data9"("Array"=w528) -> ("Dynamic Data Type"=w531:dynamicdata)  [unwired: 3 in]
                n445 = call "Build OD Plot"("Y Input"=w533, "X Input"=w531) -> ("XY Graph"=→"Optical Depth":cluster{"Y":dbl[], "Y":dbl[]}[])  [unwired: 3 in, 6 out]
              }
            }
          }
        }
        "L_Count" <- w93
      }
    }
  }
  n446 = case shown="True" w3 {
    frame False {
    }
    frame True {
      # "close data files"
      # "Close Bristol WM"
      n447 = local read "Bristol Out"() -> (w587:i32)
      n448 = local read "NF_Off_Ref"() -> (w583:refnum<file>)
      n449 = local read "WS visa"() -> (w581:refnum<visa-resource-name>)
      n450 = local read "NF_On_Ref"() -> (w584:refnum<file>)
      n451 = local read "FF_Off_Ref"() -> (w585:refnum<file>)
      n452 = local read "FF_On_Ref"() -> (w586:refnum<file>)
      n453 = local read "OphirPM"() -> (w582:T7)
      n454 = dll-call lib="C:/H2O_DIAL/LabVIEW-2012/Bristol WM V2_31b/CLDevIFace.dll" fn="CLCloseDevice"("CommPort"=w587) -> ()  [unwired: 5 in, 2 out]
      n455 = call "OphirClose.vi"("OphirPM"=w582) -> ()  [unwired: 18 in, 1 out]
      n456 = Close File(refnum=w586) -> ()  [unwired: 1 in, 2 out]
      n457 = Close File(refnum=w585) -> ()  [unwired: 1 in, 2 out]
      n458 = Close File(refnum=w584) -> ()  [unwired: 1 in, 2 out]
      n459 = Close File(refnum=w583) -> ()  [unwired: 1 in, 2 out]
      n460 = call "T_RH_P.vi"("VISA in"=w581, "WS_Commands"=enum16{"OpenWS", "ReadTRHP", "CloseWS"}."CloseWS") -> ()  [unwired: 11 in, 3 out]
    }
  }
  "FileHour" <- -1 ("FileHour")
  "DataOpen" <- FALSE
